vi "main.vi"() -> ()   [LabVIEW 2012]
uses:
  <vilib>/Utility/error.llb/DialogType.ctl
  <instrlib>/Tektronix DPO MSO 2000 4000 Series/Public/Configure/Configure Trigger (Edge).vi
  <instrlib>/Tektronix DPO MSO 2000 4000 Series/Public/Data/Data_Low Level/Fetch Waveform (Waveform Data Type).vi
  <vilib>/regexp/Match Regular Expression.xnode
  <instrlib>/Tektronix DPO MSO 2000 4000 Series/Tektronix DPO MSO 2000 4000 Series.lvlib
panel:
  in  "tabs":T1(tab)=enum."Scope"
  in  "frames":i32=20 caption="Repeated Frames"
  out "current frame":i32=20 caption="Current Frame"
  in  "repetition rate":dbl caption="Max Repetition Rate (mHz)"
  in  "dio64:resource name":refnum<visa-resource-name>="PXI4::0::INSTR"
  out "chop display":picture[](array[picture])=[bytes[78], bytes[76], bytes[76], bytes[80], bytes[84], bytes[72], bytes[72]] caption="Chop Display"
  in  "dio64":T2(array[cluster])=[{"Task"="Gas Pulse", "begin time"=19.288099999999993, "begin edge"=TRUE, "begin reference"="T0", "end time"=0.045, "end edge"=TRUE, "end reference"="<SELF>", "Chops"=[FALSE, FALSE, FALSE, FALSE, FALSE, FALSE, FALSE, FALSE, FALSE, FALSE, FALSE, FALSE]}, {"Task"="Abby Flashlamp", "begin time"=-0.001, "begin edge"=TRUE, "begin reference"="Gas Pulse", "end time"=0.01, "end edge"=TRUE, "end reference"="<SELF>", "Chops"=[FALSE, FALSE, FALSE, FALSE, FALSE, FALSE, FALSE, FALSE, FALSE, FALSE, FALSE, FALSE]}, {"Task"="Abby Q-switch", "begin time"=0.11509999999999998, "begin edge"=FALSE, "begin reference"="Abby Flashlamp", "end time"=0.01, "end edge"=TRUE, "end reference"="<SELF>", "Chops"=[FALSE, FALSE, FALSE, FALSE, FALSE, FALSE, FALSE, FALSE, FALSE, FALSE, FALSE, FALSE]}, {"Task"="Trap", "begin time"=20.1722, "begin edge"=TRUE, "begin reference"="T0", "end time"=500.12, "end edge"=TRUE, "end reference"="<SELF>", "Chops"=[FALSE, FALSE, FALSE, FALSE, FALSE, FALSE, FALSE, FALSE, FALSE, FALSE, FALSE, FALSE]}, {"Task"="Zero DAC", "begin time"=-0.04, "begin edge"=FALSE, "begin reference"="Zero DAC", "end time"=0.0, "end edge"=TRUE, "end reference"="Stop Ions", "Chops"=[FALSE, FALSE, FALSE, FALSE, FALSE, FALSE, FALSE, FALSE, FALSE, FALSE, FALSE, FALSE]}, {"Task"="Stop Ions", "begin time"=-0.001, "begin edge"=FALSE, "begin reference"="Stop Ions", "end time"=0.0, "end edge"=TRUE, "end reference"="Trap", "Chops"=[FALSE, FALSE, FALSE, FALSE, FALSE, FALSE, FALSE, FALSE, FALSE, FALSE, FALSE, FALSE]}, {"Task"="Kick to MCP", "begin time"=0.0, "begin edge"=FALSE, "begin reference"="Trap", "end time"=0.005, "end edge"=TRUE, "end reference"="<SELF>", "Chops"=[FALSE, FALSE, FALSE, FALSE, FALSE, FALSE, FALSE, FALSE, FALSE, FALSE, FALSE, FALSE]}, {"Task"="Img MCP Trigger", "begin time"=0.07001, "begin edge"=FALSE, "begin reference"="Kick to MCP", "end time"=0.01, "end edge"=TRUE, "end reference"="<SELF>", "Chops"=[TRUE, TRUE, TRUE, TRUE, TRUE, TRUE, FALSE, FALSE, FALSE, FALSE, FALSE, FALSE]}, {"Task"="Framegrabber Trigger", "begin time"=-18.0, "begin edge"=TRUE, "begin reference"="Img MCP Trigger", "end time"=0.01, "end edge"=TRUE, "end reference"="<SELF>", "Chops"=[TRUE, TRUE, TRUE, TRUE, TRUE, TRUE, FALSE, FALSE, FALSE, FALSE, FALSE, FALSE]}, {"Task"="Trigger Scope", "begin time"=0.015000000000000006, "begin edge"=FALSE, "begin reference"="Trap", "end time"=0.01, "end edge"=TRUE, "end reference"="<SELF>", "Chops"=[FALSE, FALSE, FALSE, FALSE, FALSE, FALSE, TRUE, FALSE, FALSE, FALSE, FALSE, FALSE]}, {"Task"="Trigger DAC", "begin time"=-1.0, "begin edge"=TRUE, "begin reference"="Trap", "end time"=0.01, "end edge"=TRUE, "end reference"="<SELF>", "Chops"=[FALSE, FALSE, FALSE, FALSE, FALSE, FALSE, FALSE, FALSE, FALSE, FALSE, FALSE, FALSE]}, {"Task"="Zero DAC", "begin time"=0.0, "begin edge"=FALSE, "begin reference"="Kick to MCP", "end time"=10.0, "end edge"=FALSE, "end reference"="Kick to MCP", "Chops"=[FALSE, FALSE, FALSE, FALSE, FALSE, FALSE, FALSE, FALSE, FALSE, FALSE, FALSE, FALSE]}, {"Task"="IOUpdate", "begin time"=-1.9976, "begin edge"=TRUE, "begin reference"="Trap", "end time"=0.01, "end edge"=TRUE, "end reference"="<SELF>", "Chops"=[FALSE, FALSE, FALSE, FALSE, FALSE, FALSE, FALSE, FALSE, FALSE, FALSE, FALSE, FALSE]}, {"Task"="Jessica Shutter", "begin time"=-20.0, "begin edge"=TRUE, "begin reference"="Trap", "end time"=100.0, "end edge"=TRUE, "end reference"="<SELF>", "Chops"=[FALSE, FALSE, FALSE, FALSE, FALSE, FALSE, FALSE, FALSE, FALSE, FALSE, FALSE, FALSE]}, {"Task"="Bertha UV Shutter", "begin time"=-20.0, "begin edge"=TRUE, "begin reference"="Trap", "end time"=100.0, "end edge"=TRUE, "end reference"="<SELF>", "Chops"=[FALSE, FALSE, FALSE, FALSE, FALSE, FALSE, FALSE, FALSE, FALSE, FALSE, FALSE, FALSE]}, {"Task"="Scope trigger 2", "begin time"=0.0, "begin edge"=FALSE, "begin reference"="Trap", "end time"=0.01, "end edge"=TRUE, "end reference"="<SELF>", "Chops"=[TRUE, TRUE, TRUE, FALSE, FALSE, FALSE, FALSE, FALSE, FALSE, FALSE, FALSE, FALSE]}, {"Task"="DDS Ramp 1", "begin time"=11.0, "begin edge"=TRUE, "begin reference"="Trap", "end time"=-1.0, "end edge"=TRUE, "end reference"="Unchillax", "Chops"=[FALSE, FALSE, FALSE, FALSE, TRUE, TRUE, TRUE, FALSE, FALSE, FALSE, FALSE, FALSE]}, {"Task"="Stella Fiber Switch", "begin time"=12.0, "begin edge"=TRUE, "begin reference"="Trap", "end time"=80.0, "end edge"=TRUE, "end reference"="<SELF>", "Chops"=[FALSE, FALSE, FALSE, TRUE, TRUE, TRUE, TRUE, FALSE, FALSE, FALSE, FALSE, FALSE]}, {"Task"="Toptica Fiber Switch", "begin time"=0.0, "begin edge"=TRUE, "begin reference"="Stella Fiber Switch", "end time"=85.0, "end edge"=TRUE, "end reference"="<SELF>", "Chops"=[FALSE, FALSE, FALSE, TRUE, TRUE, TRUE, TRUE, FALSE, FALSE, FALSE, FALSE, FALSE]}, {"Task"="Scope trigger 2 transfer", "begin time"=0.0, "begin edge"=FALSE, "begin reference"="Stella Fiber Switch", "end time"=0.01, "end edge"=TRUE, "end reference"="<SELF>", "Chops"=[TRUE, TRUE, FALSE, TRUE, TRUE, TRUE, TRUE, FALSE, FALSE, FALSE, FALSE, FALSE]}, {"Task"="Change Toptica Wavelength", "begin time"=-10.0, "begin edge"=TRUE, "begin reference"="Trigger Depletion", "end time"=100.0, "end edge"=FALSE, "end reference"="Trigger Depletion 2", "Chops"=[FALSE, FALSE, FALSE, FALSE, TRUE, TRUE, TRUE, FALSE, FALSE, FALSE, FALSE, FALSE]}, {"Task"="Trigger Depletion", "begin time"=110.0, "begin edge"=TRUE, "begin reference"="Trap", "end time"=3.0, "end edge"=TRUE, "end reference"="<SELF>", "Chops"=[FALSE, FALSE, TRUE, TRUE, TRUE, TRUE, TRUE, FALSE, FALSE, FALSE, FALSE, FALSE]}, {"Task"="Trigger Depletion 2", "begin time"=6.0, "begin edge"=FALSE, "begin reference"="Pi/2 Pulse 2", "end time"=3.0, "end edge"=TRUE, "end reference"="<SELF>", "Chops"=[TRUE, FALSE, TRUE, TRUE, TRUE, TRUE, TRUE, FALSE, FALSE, FALSE, FALSE, FALSE]}, {"Task"="Trigger Depletion 2-dephase", "begin time"=0.002, "begin edge"=TRUE, "begin reference"="Trigger Depletion 2", "end time"=3.0, "end edge"=TRUE, "end reference"="<SELF>", "Chops"=[FALSE, TRUE, TRUE, TRUE, TRUE, TRUE, TRUE, FALSE, FALSE, FALSE, FALSE, FALSE]}, {"Task"="Scope trigger 2 depletion", "begin time"=0.0, "begin edge"=TRUE, "begin reference"="Trigger Depletion", "end time"=0.01, "end edge"=TRUE, "end reference"="<SELF>", "Chops"=[FALSE, FALSE, TRUE, TRUE, TRUE, TRUE, TRUE, FALSE, FALSE, FALSE, FALSE, FALSE]}, {"Task"="Cora Shutter", "begin time"=0.0, "begin edge"=TRUE, "begin reference"="266nm Shutter", "end time"=1.0, "end edge"=FALSE, "end reference"="Trap", "Chops"=[FALSE, FALSE, FALSE, FALSE, TRUE, TRUE, TRUE, FALSE, FALSE, FALSE, FALSE, FALSE]}, {"Task"="266nm Shutter", "begin time"=-20.0, "begin edge"=TRUE, "begin reference"="End Ramp", "end time"=0.0, "end edge"=FALSE, "end reference"="Cora Shutter", "Chops"=[FALSE, FALSE, FALSE, FALSE, FALSE, TRUE, TRUE, FALSE, FALSE, FALSE, FALSE, FALSE]}, {"Task"="Chillax", "begin time"=-1.0, "begin edge"=TRUE, "begin reference"="Trap", "end time"=0.01, "end edge"=TRUE, "end reference"="<SELF>", "Chops"=[FALSE, FALSE, FALSE, FALSE, FALSE, FALSE, FALSE, FALSE, FALSE, FALSE, FALSE, FALSE]}, {"Task"="Unchillax", "begin time"=-6.0, "begin edge"=TRUE, "begin reference"="End Ramp", "end time"=0.01, "end edge"=TRUE, "end reference"="<SELF>", "Chops"=[FALSE, FALSE, FALSE, FALSE, FALSE, TRUE, TRUE, FALSE, FALSE, FALSE, FALSE, FALSE]}, {"Task"="End Ramp", "begin time"=-102.0, "begin edge"=FALSE, "begin reference"="Trap", "end time"=0.01, "end edge"=TRUE, "end reference"="<SELF>", "Chops"=[FALSE, FALSE, FALSE, FALSE, FALSE, TRUE, TRUE, FALSE, FALSE, FALSE, FALSE, FALSE]}, {"Task"="End Ramp 2", "begin time"=33.33, "begin edge"=TRUE, "begin reference"="End Ramp", "end time"=33.34, "end edge"=TRUE, "end reference"="End Ramp", "Chops"=[FALSE, FALSE, FALSE, FALSE, FALSE, TRUE, TRUE, FALSE, FALSE, FALSE, FALSE, FALSE]}, {"Task"="End Ramp 2", "begin time"=66.67, "begin edge"=TRUE, "begin reference"="End Ramp", "end time"=66.68, "end edge"=TRUE, "end reference"="End Ramp", "Chops"=[FALSE, FALSE, FALSE, FALSE, FALSE, TRUE, TRUE, FALSE, FALSE, FALSE, FALSE, FALSE]}, {"Task"="End Ramp 2", "begin time"=100.0, "begin edge"=TRUE, "begin reference"="End Ramp", "end time"=100.01, "end edge"=TRUE, "end reference"="End Ramp", "Chops"=[FALSE, FALSE, FALSE, FALSE, FALSE, TRUE, TRUE, FALSE, FALSE, FALSE, FALSE, FALSE]}, {"Task"="Pi/2 Pulse", "begin time"=5.0, "begin edge"=FALSE, "begin reference"="Trigger Depletion", "end time"=0.95, "end edge"=TRUE, "end reference"="<SELF>", "Chops"=[FALSE, FALSE, FALSE, FALSE, TRUE, TRUE, TRUE, FALSE, FALSE, FALSE, FALSE, FALSE]}, {"Task"="Pi/2 Pulse 2", "begin time"=256.0, "begin edge"=FALSE, "begin reference"="Pi/2 Pulse", "end time"=0.95, "end edge"=TRUE, "end reference"="<SELF>", "Chops"=[FALSE, FALSE, FALSE, FALSE, TRUE, TRUE, TRUE, FALSE, FALSE, FALSE, FALSE, FALSE]}] caption="DIO64" {"end time" format="%#_8g"; "begin time" format="%#_8g"}
  in  "dio64:tasks":T3(array[cluster])=[{"Name"="Gas Pulse", "DIO64 Line 1"=[FALSE, FALSE, FALSE, FALSE, FALSE, FALSE, FALSE, FALSE, FALSE, FALSE, FALSE, FALSE, FALSE, FALSE, TRUE, FALSE], "DIO64 Line 2"=[FALSE, FALSE, FALSE, FALSE, FALSE, FALSE, FALSE, FALSE, FALSE, FALSE, FALSE, FALSE, FALSE, FALSE, FALSE, FALSE], "DIO64 Line 3"=[FALSE, FALSE, FALSE, FALSE, FALSE, FALSE, FALSE, FALSE, FALSE, FALSE, FALSE, FALSE, FALSE, FALSE, FALSE, FALSE], "DIO64 Line 4"=[FALSE, FALSE, FALSE, FALSE, FALSE, FALSE, FALSE, FALSE, FALSE, FALSE, FALSE, FALSE, FALSE, FALSE, FALSE, FALSE]}, {"Name"="Abby Flashlamp", "DIO64 Line 1"=[FALSE, FALSE, FALSE, TRUE, FALSE, FALSE, FALSE, FALSE, FALSE, FALSE, FALSE, FALSE, FALSE, FALSE, FALSE, FALSE], "DIO64 Line 2"=[FALSE, FALSE, FALSE, FALSE, FALSE, FALSE, FALSE, FALSE, FALSE, FALSE, FALSE, FALSE, FALSE, FALSE, FALSE, FALSE], "DIO64 Line 3"=[FALSE, FALSE, FALSE, FALSE, FALSE, FALSE, FALSE, FALSE, FALSE, FALSE, FALSE, FALSE, FALSE, FALSE, FALSE, FALSE], "DIO64 Line 4"=[FALSE, FALSE, FALSE, FALSE, FALSE, FALSE, FALSE, FALSE, FALSE, FALSE, FALSE, FALSE, FALSE, FALSE, FALSE, FALSE]}, {"Name"="Abby Q-switch", "DIO64 Line 1"=[FALSE, FALSE, FALSE, FALSE, TRUE, FALSE, FALSE, FALSE, FALSE, FALSE, FALSE, FALSE, FALSE, FALSE, FALSE, FALSE], "DIO64 Line 2"=[FALSE, FALSE, FALSE, FALSE, FALSE, FALSE, FALSE, FALSE, FALSE, FALSE, FALSE, FALSE, FALSE, FALSE, FALSE, FALSE], "DIO64 Line 3"=[FALSE, FALSE, FALSE, FALSE, FALSE, FALSE, FALSE, FALSE, FALSE, FALSE, FALSE, FALSE, FALSE, FALSE, FALSE, FALSE], "DIO64 Line 4"=[FALSE, FALSE, FALSE, FALSE, FALSE, FALSE, FALSE, FALSE, FALSE, FALSE, FALSE, FALSE, FALSE, FALSE, FALSE, FALSE]}, {"Name"="Stop Ions", "DIO64 Line 1"=[FALSE, FALSE, FALSE, FALSE, FALSE, FALSE, FALSE, FALSE, FALSE, TRUE, FALSE, FALSE, FALSE, FALSE, FALSE, FALSE], "DIO64 Line 2"=[FALSE, FALSE, FALSE, FALSE, FALSE, FALSE, FALSE, FALSE, FALSE, FALSE, FALSE, FALSE, FALSE, FALSE, FALSE, FALSE], "DIO64 Line 3"=[FALSE, FALSE, FALSE, FALSE, FALSE, FALSE, FALSE, FALSE, FALSE, FALSE, FALSE, FALSE, FALSE, FALSE, FALSE, FALSE], "DIO64 Line 4"=[FALSE, FALSE, FALSE, FALSE, FALSE, FALSE, FALSE, FALSE, FALSE, FALSE, FALSE, FALSE, FALSE, FALSE, FALSE, FALSE]}, {"Name"="Trap", "DIO64 Line 1"=[FALSE, FALSE, FALSE, FALSE, FALSE, FALSE, TRUE, FALSE, FALSE, FALSE, FALSE, FALSE, FALSE, FALSE, FALSE, FALSE], "DIO64 Line 2"=[FALSE, FALSE, FALSE, FALSE, TRUE, FALSE, FALSE, FALSE, FALSE, FALSE, FALSE, FALSE, FALSE, TRUE, FALSE, FALSE], "DIO64 Line 3"=[FALSE, FALSE, FALSE, TRUE, FALSE, FALSE, FALSE, FALSE, FALSE, FALSE, FALSE, FALSE, FALSE, FALSE, FALSE, FALSE], "DIO64 Line 4"=[FALSE, FALSE, FALSE, FALSE, FALSE, FALSE, FALSE, FALSE, FALSE, FALSE, FALSE, FALSE, FALSE, FALSE, FALSE, TRUE]}, {"Name"="Zero DAC", "DIO64 Line 1"=[FALSE, FALSE, FALSE, FALSE, FALSE, FALSE, FALSE, FALSE, FALSE, TRUE, TRUE, FALSE, FALSE, FALSE, FALSE, FALSE], "DIO64 Line 2"=[FALSE, FALSE, FALSE, FALSE, FALSE, FALSE, FALSE, FALSE, FALSE, FALSE, FALSE, FALSE, FALSE, FALSE, FALSE, FALSE], "DIO64 Line 3"=[FALSE, FALSE, FALSE, FALSE, FALSE, FALSE, FALSE, FALSE, FALSE, FALSE, FALSE, FALSE, FALSE, FALSE, FALSE, FALSE], "DIO64 Line 4"=[FALSE, FALSE, FALSE, FALSE, FALSE, FALSE, FALSE, FALSE, FALSE, FALSE, FALSE, FALSE, FALSE, FALSE, FALSE, FALSE]}, {"Name"="Kick to MCP", "DIO64 Line 1"=[FALSE, FALSE, FALSE, FALSE, FALSE, FALSE, FALSE, FALSE, FALSE, TRUE, FALSE, FALSE, FALSE, FALSE, FALSE, FALSE], "DIO64 Line 2"=[FALSE, FALSE, FALSE, FALSE, FALSE, FALSE, FALSE, FALSE, FALSE, FALSE, FALSE, FALSE, FALSE, FALSE, FALSE, FALSE], "DIO64 Line 3"=[FALSE, FALSE, FALSE, FALSE, FALSE, FALSE, FALSE, FALSE, FALSE, FALSE, FALSE, FALSE, FALSE, FALSE, FALSE, FALSE], "DIO64 Line 4"=[FALSE, FALSE, FALSE, FALSE, FALSE, FALSE, FALSE, FALSE, FALSE, FALSE, FALSE, FALSE, FALSE, FALSE, FALSE, FALSE]}, {"Name"="Trap Frequency", "DIO64 Line 1"=[FALSE, FALSE, FALSE, FALSE, FALSE, FALSE, FALSE, FALSE, FALSE, FALSE, FALSE, FALSE, FALSE, FALSE, FALSE, FALSE], "DIO64 Line 2"=[FALSE, FALSE, FALSE, FALSE, FALSE, FALSE, FALSE, FALSE, FALSE, FALSE, FALSE, FALSE, FALSE, FALSE, FALSE, FALSE], "DIO64 Line 3"=[FALSE, FALSE, FALSE, FALSE, FALSE, FALSE, FALSE, FALSE, FALSE, FALSE, FALSE, FALSE, FALSE, FALSE, FALSE, FALSE], "DIO64 Line 4"=[FALSE, FALSE, FALSE, FALSE, FALSE, FALSE, FALSE, FALSE, FALSE, FALSE, FALSE, FALSE, FALSE, FALSE, FALSE, FALSE]}, {"Name"="Trigger Scope", "DIO64 Line 1"=[FALSE, FALSE, FALSE, FALSE, FALSE, FALSE, FALSE, TRUE, FALSE, FALSE, FALSE, FALSE, FALSE, FALSE, FALSE, FALSE], "DIO64 Line 2"=[FALSE, FALSE, FALSE, FALSE, FALSE, FALSE, FALSE, FALSE, FALSE, FALSE, FALSE, FALSE, FALSE, FALSE, FALSE, FALSE], "DIO64 Line 3"=[FALSE, FALSE, FALSE, FALSE, FALSE, FALSE, FALSE, FALSE, FALSE, FALSE, FALSE, FALSE, FALSE, FALSE, FALSE, FALSE], "DIO64 Line 4"=[FALSE, TRUE, FALSE, FALSE, FALSE, FALSE, FALSE, FALSE, FALSE, FALSE, FALSE, FALSE, FALSE, FALSE, FALSE, FALSE]}, {"Name"="End Cap SW0", "DIO64 Line 1"=[FALSE, FALSE, FALSE, FALSE, FALSE, FALSE, FALSE, FALSE, FALSE, FALSE, FALSE, FALSE, FALSE, FALSE, FALSE, FALSE], "DIO64 Line 2"=[FALSE, FALSE, FALSE, FALSE, TRUE, FALSE, FALSE, FALSE, FALSE, FALSE, FALSE, FALSE, FALSE, FALSE, FALSE, FALSE], "DIO64 Line 3"=[FALSE, FALSE, FALSE, FALSE, FALSE, FALSE, FALSE, FALSE, FALSE, FALSE, FALSE, FALSE, FALSE, FALSE, FALSE, FALSE], "DIO64 Line 4"=[FALSE, FALSE, FALSE, FALSE, FALSE, FALSE, FALSE, FALSE, FALSE, FALSE, FALSE, FALSE, FALSE, FALSE, FALSE, FALSE]}, {"Name"="Framegrabber Trigger", "DIO64 Line 1"=[FALSE, FALSE, FALSE, FALSE, FALSE, FALSE, FALSE, FALSE, FALSE, FALSE, FALSE, FALSE, FALSE, FALSE, FALSE, TRUE], "DIO64 Line 2"=[FALSE, FALSE, FALSE, FALSE, FALSE, FALSE, FALSE, FALSE, FALSE, FALSE, FALSE, FALSE, FALSE, FALSE, FALSE, FALSE], "DIO64 Line 3"=[FALSE, FALSE, FALSE, FALSE, FALSE, FALSE, FALSE, FALSE, FALSE, FALSE, FALSE, FALSE, FALSE, FALSE, FALSE, FALSE], "DIO64 Line 4"=[FALSE, FALSE, TRUE, FALSE, FALSE, FALSE, FALSE, FALSE, FALSE, FALSE, FALSE, FALSE, FALSE, FALSE, FALSE, FALSE]}, {"Name"="Lisa Shutter", "DIO64 Line 1"=[FALSE, FALSE, FALSE, FALSE, FALSE, FALSE, FALSE, FALSE, FALSE, FALSE, FALSE, FALSE, FALSE, FALSE, FALSE, FALSE], "DIO64 Line 2"=[TRUE, FALSE, FALSE, FALSE, FALSE, FALSE, FALSE, FALSE, FALSE, FALSE, FALSE, FALSE, FALSE, FALSE, FALSE, FALSE], "DIO64 Line 3"=[FALSE, FALSE, FALSE, FALSE, FALSE, FALSE, FALSE, FALSE, FALSE, FALSE, FALSE, FALSE, FALSE, FALSE, FALSE, FALSE], "DIO64 Line 4"=[FALSE, FALSE, FALSE, FALSE, FALSE, FALSE, FALSE, FALSE, FALSE, FALSE, FALSE, FALSE, FALSE, FALSE, FALSE, FALSE]}, {"Name"="Trigger DAC", "DIO64 Line 1"=[FALSE, FALSE, FALSE, FALSE, FALSE, FALSE, FALSE, FALSE, FALSE, FALSE, FALSE, FALSE, FALSE, FALSE, FALSE, FALSE], "DIO64 Line 2"=[FALSE, FALSE, FALSE, FALSE, FALSE, FALSE, FALSE, FALSE, FALSE, TRUE, FALSE, FALSE, FALSE, FALSE, FALSE, FALSE], "DIO64 Line 3"=[FALSE, FALSE, FALSE, FALSE, FALSE, FALSE, FALSE, FALSE, FALSE, FALSE, FALSE, FALSE, FALSE, FALSE, FALSE, FALSE], "DIO64 Line 4"=[FALSE, FALSE, FALSE, FALSE, FALSE, FALSE, FALSE, FALSE, FALSE, FALSE, FALSE, FALSE, FALSE, FALSE, FALSE, FALSE]}, {"Name"="Jessica Shutter", "DIO64 Line 1"=[FALSE, FALSE, FALSE, FALSE, FALSE, FALSE, FALSE, FALSE, FALSE, FALSE, FALSE, FALSE, FALSE, TRUE, FALSE, FALSE], "DIO64 Line 2"=[FALSE, FALSE, FALSE, FALSE, FALSE, FALSE, FALSE, FALSE, FALSE, FALSE, FALSE, FALSE, FALSE, FALSE, FALSE, FALSE], "DIO64 Line 3"=[FALSE, FALSE, FALSE, FALSE, FALSE, FALSE, FALSE, FALSE, FALSE, FALSE, FALSE, FALSE, FALSE, FALSE, FALSE, FALSE], "DIO64 Line 4"=[FALSE, FALSE, FALSE, FALSE, FALSE, FALSE, FALSE, FALSE, FALSE, FALSE, FALSE, FALSE, FALSE, FALSE, FALSE, FALSE]}, {"Name"="Img MCP Trigger", "DIO64 Line 1"=[FALSE, FALSE, FALSE, FALSE, FALSE, TRUE, FALSE, FALSE, FALSE, FALSE, FALSE, FALSE, FALSE, FALSE, FALSE, FALSE], "DIO64 Line 2"=[FALSE, FALSE, FALSE, FALSE, FALSE, FALSE, FALSE, FALSE, FALSE, FALSE, FALSE, FALSE, FALSE, FALSE, FALSE, FALSE], "DIO64 Line 3"=[FALSE, FALSE, FALSE, FALSE, FALSE, FALSE, FALSE, FALSE, FALSE, FALSE, FALSE, FALSE, FALSE, FALSE, FALSE, FALSE], "DIO64 Line 4"=[FALSE, FALSE, FALSE, FALSE, FALSE, FALSE, FALSE, FALSE, FALSE, FALSE, FALSE, FALSE, FALSE, FALSE, FALSE, FALSE]}, {"Name"="Nothing", "DIO64 Line 1"=[FALSE, FALSE, FALSE, FALSE, FALSE, FALSE, FALSE, FALSE, FALSE, FALSE, FALSE, FALSE, FALSE, FALSE, FALSE, FALSE], "DIO64 Line 2"=[FALSE, FALSE, FALSE, FALSE, FALSE, FALSE, FALSE, FALSE, FALSE, FALSE, FALSE, FALSE, FALSE, FALSE, FALSE, FALSE], "DIO64 Line 3"=[FALSE, FALSE, FALSE, FALSE, FALSE, FALSE, FALSE, FALSE, FALSE, FALSE, FALSE, FALSE, FALSE, FALSE, FALSE, FALSE], "DIO64 Line 4"=[FALSE, FALSE, FALSE, FALSE, FALSE, FALSE, FALSE, FALSE, FALSE, FALSE, FALSE, FALSE, FALSE, FALSE, FALSE, FALSE]}, {"Name"="End Ramp", "DIO64 Line 1"=[FALSE, FALSE, FALSE, FALSE, FALSE, FALSE, FALSE, FALSE, FALSE, FALSE, FALSE, FALSE, TRUE, FALSE, FALSE, FALSE], "DIO64 Line 2"=[FALSE, FALSE, FALSE, FALSE, FALSE, FALSE, FALSE, FALSE, FALSE, FALSE, FALSE, FALSE, FALSE, FALSE, FALSE, FALSE], "DIO64 Line 3"=[FALSE, FALSE, FALSE, FALSE, FALSE, FALSE, FALSE, FALSE, FALSE, FALSE, FALSE, FALSE, FALSE, FALSE, FALSE, FALSE], "DIO64 Line 4"=[FALSE, FALSE, FALSE, FALSE, FALSE, FALSE, FALSE, FALSE, FALSE, FALSE, FALSE, FALSE, FALSE, FALSE, FALSE, FALSE]}, {"Name"="End Ramp 2", "DIO64 Line 1"=[FALSE, FALSE, FALSE, FALSE, FALSE, FALSE, FALSE, FALSE, FALSE, FALSE, FALSE, FALSE, TRUE, FALSE, FALSE, FALSE], "DIO64 Line 2"=[FALSE, FALSE, FALSE, FALSE, FALSE, FALSE, FALSE, FALSE, FALSE, FALSE, FALSE, FALSE, FALSE, FALSE, FALSE, FALSE], "DIO64 Line 3"=[FALSE, FALSE, FALSE, FALSE, FALSE, FALSE, FALSE, FALSE, FALSE, FALSE, FALSE, FALSE, FALSE, FALSE, FALSE, FALSE], "DIO64 Line 4"=[FALSE, FALSE, FALSE, FALSE, FALSE, FALSE, FALSE, FALSE, FALSE, FALSE, FALSE, FALSE, FALSE, FALSE, FALSE, FALSE]}, {"Name"="Step Bertha Scan", "DIO64 Line 1"=[FALSE, FALSE, FALSE, FALSE, FALSE, FALSE, FALSE, FALSE, FALSE, FALSE, FALSE, FALSE, FALSE, FALSE, FALSE, FALSE], "DIO64 Line 2"=[FALSE, FALSE, FALSE, FALSE, FALSE, FALSE, FALSE, FALSE, FALSE, FALSE, FALSE, TRUE, FALSE, FALSE, FALSE, FALSE], "DIO64 Line 3"=[FALSE, FALSE, FALSE, FALSE, FALSE, FALSE, FALSE, FALSE, FALSE, FALSE, FALSE, FALSE, FALSE, FALSE, FALSE, FALSE], "DIO64 Line 4"=[FALSE, FALSE, FALSE, FALSE, FALSE, FALSE, FALSE, FALSE, FALSE, FALSE, FALSE, FALSE, FALSE, FALSE, FALSE, FALSE]}, {"Name"="Bertha UV Shutter", "DIO64 Line 1"=[FALSE, FALSE, FALSE, FALSE, FALSE, FALSE, FALSE, FALSE, FALSE, FALSE, FALSE, FALSE, FALSE, FALSE, FALSE, FALSE], "DIO64 Line 2"=[FALSE, FALSE, FALSE, FALSE, FALSE, FALSE, FALSE, FALSE, FALSE, FALSE, FALSE, FALSE, FALSE, FALSE, FALSE, TRUE], "DIO64 Line 3"=[FALSE, FALSE, FALSE, FALSE, FALSE, FALSE, FALSE, FALSE, FALSE, FALSE, FALSE, FALSE, FALSE, FALSE, FALSE, FALSE], "DIO64 Line 4"=[FALSE, FALSE, FALSE, FALSE, FALSE, FALSE, FALSE, FALSE, FALSE, FALSE, FALSE, FALSE, FALSE, FALSE, FALSE, FALSE]}, {"Name"="Kick to Fast MCP TOFMS", "DIO64 Line 1"=[FALSE, FALSE, FALSE, FALSE, FALSE, TRUE, FALSE, FALSE, FALSE, FALSE, FALSE, FALSE, FALSE, FALSE, FALSE, FALSE], "DIO64 Line 2"=[FALSE, FALSE, FALSE, FALSE, FALSE, FALSE, FALSE, FALSE, FALSE, FALSE, FALSE, FALSE, FALSE, FALSE, FALSE, FALSE], "DIO64 Line 3"=[FALSE, FALSE, FALSE, FALSE, FALSE, FALSE, FALSE, FALSE, FALSE, FALSE, FALSE, FALSE, FALSE, FALSE, FALSE, FALSE], "DIO64 Line 4"=[FALSE, FALSE, FALSE, FALSE, FALSE, FALSE, FALSE, FALSE, FALSE, FALSE, FALSE, FALSE, FALSE, FALSE, FALSE, FALSE]}, {"Name"="End Cap SW1", "DIO64 Line 1"=[FALSE, FALSE, FALSE, FALSE, FALSE, FALSE, FALSE, FALSE, FALSE, FALSE, FALSE, FALSE, FALSE, FALSE, FALSE, FALSE], "DIO64 Line 2"=[FALSE, FALSE, FALSE, FALSE, FALSE, FALSE, FALSE, FALSE, FALSE, FALSE, FALSE, FALSE, FALSE, TRUE, FALSE, FALSE], "DIO64 Line 3"=[FALSE, FALSE, FALSE, FALSE, FALSE, FALSE, FALSE, FALSE, FALSE, FALSE, FALSE, FALSE, FALSE, FALSE, FALSE, FALSE], "DIO64 Line 4"=[FALSE, FALSE, FALSE, FALSE, FALSE, FALSE, FALSE, FALSE, FALSE, FALSE, FALSE, FALSE, FALSE, FALSE, FALSE, FALSE]}, {"Name"="Scope trigger 2", "DIO64 Line 1"=[FALSE, FALSE, FALSE, FALSE, FALSE, FALSE, FALSE, FALSE, FALSE, FALSE, FALSE, FALSE, FALSE, FALSE, FALSE, FALSE], "DIO64 Line 2"=[FALSE, FALSE, FALSE, FALSE, FALSE, FALSE, FALSE, FALSE, FALSE, FALSE, FALSE, TRUE, FALSE, FALSE, FALSE, FALSE], "DIO64 Line 3"=[FALSE, FALSE, FALSE, FALSE, FALSE, FALSE, FALSE, FALSE, FALSE, FALSE, FALSE, FALSE, FALSE, FALSE, FALSE, FALSE], "DIO64 Line 4"=[FALSE, FALSE, FALSE, FALSE, FALSE, FALSE, FALSE, FALSE, FALSE, FALSE, FALSE, FALSE, FALSE, FALSE, FALSE, FALSE]}, {"Name"="266nm Shutter", "DIO64 Line 1"=[FALSE, FALSE, FALSE, FALSE, FALSE, FALSE, FALSE, FALSE, FALSE, FALSE, FALSE, FALSE, FALSE, FALSE, FALSE, FALSE], "DIO64 Line 2"=[FALSE, FALSE, FALSE, FALSE, FALSE, TRUE, FALSE, FALSE, FALSE, FALSE, FALSE, FALSE, FALSE, FALSE, FALSE, FALSE], "DIO64 Line 3"=[FALSE, FALSE, FALSE, FALSE, FALSE, FALSE, FALSE, FALSE, FALSE, FALSE, FALSE, FALSE, FALSE, FALSE, FALSE, FALSE], "DIO64 Line 4"=[FALSE, FALSE, FALSE, FALSE, FALSE, FALSE, FALSE, FALSE, FALSE, FALSE, FALSE, FALSE, FALSE, FALSE, FALSE, FALSE]}, {"Name"="532/1064nm Shutter", "DIO64 Line 1"=[FALSE, FALSE, FALSE, FALSE, FALSE, FALSE, FALSE, FALSE, FALSE, FALSE, FALSE, FALSE, FALSE, FALSE, FALSE, FALSE], "DIO64 Line 2"=[FALSE, FALSE, FALSE, FALSE, FALSE, FALSE, TRUE, FALSE, FALSE, FALSE, FALSE, FALSE, FALSE, FALSE, FALSE, FALSE], "DIO64 Line 3"=[FALSE, FALSE, FALSE, FALSE, FALSE, FALSE, FALSE, FALSE, FALSE, FALSE, FALSE, FALSE, FALSE, FALSE, FALSE, FALSE], "DIO64 Line 4"=[FALSE, FALSE, FALSE, FALSE, FALSE, FALSE, FALSE, FALSE, FALSE, FALSE, FALSE, FALSE, FALSE, FALSE, FALSE, FALSE]}, {"Name"="Bertha Fund Shutter", "DIO64 Line 1"=[FALSE, FALSE, FALSE, FALSE, FALSE, FALSE, FALSE, FALSE, FALSE, FALSE, FALSE, FALSE, FALSE, FALSE, FALSE, FALSE], "DIO64 Line 2"=[FALSE, FALSE, FALSE, FALSE, FALSE, FALSE, FALSE, FALSE, FALSE, FALSE, FALSE, FALSE, FALSE, FALSE, FALSE, FALSE], "DIO64 Line 3"=[FALSE, FALSE, FALSE, FALSE, FALSE, FALSE, FALSE, FALSE, FALSE, FALSE, FALSE, FALSE, FALSE, FALSE, FALSE, FALSE], "DIO64 Line 4"=[FALSE, FALSE, FALSE, FALSE, FALSE, FALSE, FALSE, FALSE, FALSE, FALSE, FALSE, FALSE, FALSE, FALSE, FALSE, FALSE]}, {"Name"="toptica aom switch", "DIO64 Line 1"=[FALSE, TRUE, FALSE, FALSE, FALSE, FALSE, FALSE, FALSE, FALSE, FALSE, FALSE, FALSE, FALSE, FALSE, FALSE, FALSE], "DIO64 Line 2"=[FALSE, FALSE, FALSE, FALSE, FALSE, FALSE, FALSE, FALSE, FALSE, FALSE, FALSE, FALSE, FALSE, FALSE, FALSE, FALSE], "DIO64 Line 3"=[FALSE, FALSE, FALSE, FALSE, FALSE, FALSE, FALSE, FALSE, FALSE, FALSE, FALSE, TRUE, FALSE, FALSE, FALSE, FALSE], "DIO64 Line 4"=[FALSE, FALSE, FALSE, FALSE, FALSE, FALSE, FALSE, FALSE, FALSE, FALSE, FALSE, FALSE, FALSE, FALSE, FALSE, FALSE]}, {"Name"="Stop Voltage", "DIO64 Line 1"=[FALSE, FALSE, FALSE, FALSE, FALSE, FALSE, FALSE, FALSE, FALSE, FALSE, FALSE, FALSE, FALSE, FALSE, FALSE, FALSE], "DIO64 Line 2"=[FALSE, FALSE, FALSE, FALSE, TRUE, FALSE, FALSE, FALSE, FALSE, FALSE, FALSE, FALSE, FALSE, FALSE, FALSE, FALSE], "DIO64 Line 3"=[FALSE, FALSE, FALSE, FALSE, FALSE, FALSE, FALSE, FALSE, FALSE, FALSE, FALSE, FALSE, FALSE, FALSE, FALSE, FALSE], "DIO64 Line 4"=[FALSE, FALSE, FALSE, FALSE, FALSE, FALSE, FALSE, FALSE, FALSE, FALSE, FALSE, FALSE, FALSE, FALSE, FALSE, FALSE]}, {"Name"="Kick Voltage", "DIO64 Line 1"=[FALSE, FALSE, FALSE, FALSE, FALSE, FALSE, FALSE, FALSE, FALSE, FALSE, FALSE, FALSE, FALSE, FALSE, FALSE, FALSE], "DIO64 Line 2"=[FALSE, FALSE, FALSE, FALSE, FALSE, FALSE, FALSE, FALSE, FALSE, FALSE, FALSE, FALSE, FALSE, FALSE, FALSE, FALSE], "DIO64 Line 3"=[FALSE, FALSE, FALSE, FALSE, FALSE, FALSE, FALSE, FALSE, FALSE, FALSE, FALSE, FALSE, FALSE, FALSE, FALSE, FALSE], "DIO64 Line 4"=[FALSE, FALSE, FALSE, FALSE, FALSE, FALSE, FALSE, FALSE, FALSE, FALSE, FALSE, FALSE, FALSE, FALSE, FALSE, FALSE]}, {"Name"="Stella Fiber Switch", "DIO64 Line 1"=[FALSE, FALSE, FALSE, FALSE, FALSE, FALSE, FALSE, FALSE, FALSE, FALSE, FALSE, FALSE, FALSE, FALSE, FALSE, FALSE], "DIO64 Line 2"=[FALSE, FALSE, FALSE, FALSE, FALSE, FALSE, FALSE, FALSE, FALSE, FALSE, FALSE, FALSE, FALSE, FALSE, TRUE, FALSE], "DIO64 Line 3"=[FALSE, FALSE, FALSE, FALSE, FALSE, FALSE, FALSE, FALSE, FALSE, FALSE, FALSE, FALSE, FALSE, FALSE, FALSE, FALSE], "DIO64 Line 4"=[FALSE, FALSE, FALSE, FALSE, FALSE, FALSE, FALSE, FALSE, FALSE, FALSE, FALSE, FALSE, FALSE, FALSE, FALSE, FALSE]}, {"Name"="Trigger Depletion 2-dephase", "DIO64 Line 1"=[FALSE, FALSE, FALSE, FALSE, FALSE, FALSE, FALSE, FALSE, FALSE, FALSE, FALSE, FALSE, FALSE, FALSE, FALSE, FALSE], "DIO64 Line 2"=[FALSE, FALSE, FALSE, FALSE, FALSE, FALSE, FALSE, FALSE, TRUE, FALSE, FALSE, FALSE, FALSE, FALSE, FALSE, FALSE], "DIO64 Line 3"=[FALSE, FALSE, FALSE, FALSE, FALSE, FALSE, FALSE, FALSE, FALSE, FALSE, FALSE, FALSE, FALSE, FALSE, FALSE, FALSE], "DIO64 Line 4"=[FALSE, FALSE, FALSE, FALSE, FALSE, FALSE, FALSE, FALSE, FALSE, FALSE, FALSE, FALSE, FALSE, FALSE, FALSE, FALSE]}, {"Name"="Cora Shutter", "DIO64 Line 1"=[FALSE, FALSE, FALSE, FALSE, FALSE, FALSE, FALSE, FALSE, FALSE, FALSE, FALSE, FALSE, FALSE, FALSE, FALSE, FALSE], "DIO64 Line 2"=[FALSE, TRUE, FALSE, FALSE, FALSE, FALSE, FALSE, FALSE, FALSE, FALSE, FALSE, FALSE, FALSE, FALSE, FALSE, FALSE], "DIO64 Line 3"=[FALSE, FALSE, FALSE, FALSE, FALSE, FALSE, FALSE, FALSE, FALSE, FALSE, FALSE, FALSE, FALSE, FALSE, FALSE, FALSE], "DIO64 Line 4"=[FALSE, FALSE, FALSE, FALSE, FALSE, FALSE, FALSE, FALSE, FALSE, FALSE, FALSE, FALSE, FALSE, FALSE, FALSE, FALSE]}, {"Name"="Step Cora Scan", "DIO64 Line 1"=[FALSE, FALSE, FALSE, FALSE, FALSE, FALSE, FALSE, FALSE, TRUE, FALSE, FALSE, FALSE, FALSE, FALSE, FALSE, FALSE], "DIO64 Line 2"=[FALSE, FALSE, FALSE, FALSE, FALSE, FALSE, FALSE, FALSE, FALSE, FALSE, FALSE, FALSE, FALSE, FALSE, FALSE, FALSE], "DIO64 Line 3"=[FALSE, FALSE, FALSE, FALSE, FALSE, FALSE, FALSE, FALSE, FALSE, FALSE, FALSE, FALSE, FALSE, FALSE, FALSE, FALSE], "DIO64 Line 4"=[FALSE, FALSE, FALSE, FALSE, FALSE, FALSE, FALSE, FALSE, FALSE, FALSE, FALSE, FALSE, FALSE, FALSE, FALSE, FALSE]}, {"Name"="DDS Ramp 1", "DIO64 Line 1"=[FALSE, FALSE, FALSE, FALSE, FALSE, FALSE, FALSE, FALSE, FALSE, FALSE, FALSE, FALSE, FALSE, FALSE, FALSE, FALSE], "DIO64 Line 2"=[TRUE, FALSE, FALSE, FALSE, FALSE, FALSE, FALSE, FALSE, FALSE, FALSE, FALSE, FALSE, FALSE, FALSE, FALSE, FALSE], "DIO64 Line 3"=[FALSE, FALSE, FALSE, FALSE, FALSE, FALSE, FALSE, FALSE, FALSE, FALSE, FALSE, FALSE, FALSE, FALSE, FALSE, FALSE], "DIO64 Line 4"=[FALSE, FALSE, FALSE, FALSE, FALSE, FALSE, FALSE, FALSE, FALSE, FALSE, FALSE, FALSE, FALSE, FALSE, FALSE, FALSE]}, {"Name"="Toptica Fiber Switch", "DIO64 Line 1"=[FALSE, FALSE, FALSE, FALSE, FALSE, FALSE, FALSE, FALSE, FALSE, FALSE, FALSE, TRUE, FALSE, FALSE, FALSE, FALSE], "DIO64 Line 2"=[FALSE, FALSE, FALSE, FALSE, FALSE, FALSE, FALSE, FALSE, FALSE, FALSE, FALSE, FALSE, FALSE, FALSE, FALSE, FALSE], "DIO64 Line 3"=[FALSE, FALSE, FALSE, FALSE, FALSE, FALSE, FALSE, FALSE, FALSE, FALSE, FALSE, FALSE, FALSE, FALSE, FALSE, FALSE], "DIO64 Line 4"=[FALSE, FALSE, FALSE, FALSE, FALSE, FALSE, FALSE, FALSE, FALSE, FALSE, FALSE, FALSE, FALSE, FALSE, FALSE, FALSE]}, {"Name"="Trigger Rotating", "DIO64 Line 1"=[FALSE, FALSE, FALSE, FALSE, FALSE, FALSE, FALSE, FALSE, FALSE, FALSE, FALSE, FALSE, FALSE, FALSE, FALSE, FALSE], "DIO64 Line 2"=[FALSE, FALSE, TRUE, FALSE, FALSE, FALSE, FALSE, FALSE, FALSE, FALSE, FALSE, FALSE, FALSE, FALSE, FALSE, FALSE], "DIO64 Line 3"=[FALSE, FALSE, FALSE, FALSE, FALSE, FALSE, FALSE, FALSE, FALSE, FALSE, FALSE, FALSE, FALSE, FALSE, FALSE, FALSE], "DIO64 Line 4"=[FALSE, FALSE, FALSE, FALSE, FALSE, FALSE, FALSE, FALSE, FALSE, FALSE, FALSE, FALSE, FALSE, FALSE, FALSE, FALSE]}, {"Name"="IOUpdate", "DIO64 Line 1"=[FALSE, FALSE, FALSE, FALSE, FALSE, FALSE, FALSE, FALSE, FALSE, FALSE, FALSE, FALSE, FALSE, FALSE, FALSE, FALSE], "DIO64 Line 2"=[FALSE, FALSE, FALSE, FALSE, FALSE, FALSE, FALSE, FALSE, FALSE, FALSE, FALSE, FALSE, FALSE, FALSE, FALSE, FALSE], "DIO64 Line 3"=[FALSE, FALSE, FALSE, FALSE, FALSE, FALSE, FALSE, FALSE, FALSE, FALSE, FALSE, FALSE, FALSE, FALSE, FALSE, FALSE], "DIO64 Line 4"=[TRUE, FALSE, FALSE, FALSE, FALSE, FALSE, FALSE, FALSE, FALSE, FALSE, FALSE, FALSE, FALSE, FALSE, FALSE, FALSE]}, {"Name"="Trigger Depletion", "DIO64 Line 1"=[FALSE, FALSE, FALSE, FALSE, FALSE, FALSE, FALSE, FALSE, FALSE, FALSE, FALSE, FALSE, FALSE, FALSE, FALSE, FALSE], "DIO64 Line 2"=[FALSE, FALSE, FALSE, FALSE, FALSE, FALSE, FALSE, FALSE, TRUE, FALSE, FALSE, FALSE, FALSE, FALSE, FALSE, FALSE], "DIO64 Line 3"=[FALSE, FALSE, FALSE, FALSE, FALSE, FALSE, FALSE, FALSE, FALSE, FALSE, FALSE, FALSE, FALSE, FALSE, FALSE, FALSE], "DIO64 Line 4"=[FALSE, FALSE, FALSE, FALSE, FALSE, FALSE, FALSE, FALSE, FALSE, FALSE, FALSE, FALSE, FALSE, FALSE, FALSE, FALSE]}, {"Name"="Trigger Depletion 2", "DIO64 Line 1"=[FALSE, FALSE, FALSE, FALSE, FALSE, FALSE, FALSE, FALSE, FALSE, FALSE, FALSE, FALSE, FALSE, FALSE, FALSE, FALSE], "DIO64 Line 2"=[FALSE, FALSE, FALSE, FALSE, FALSE, FALSE, FALSE, FALSE, TRUE, FALSE, FALSE, FALSE, FALSE, FALSE, FALSE, FALSE], "DIO64 Line 3"=[FALSE, FALSE, FALSE, FALSE, FALSE, FALSE, FALSE, FALSE, FALSE, FALSE, FALSE, FALSE, FALSE, FALSE, FALSE, FALSE], "DIO64 Line 4"=[FALSE, FALSE, FALSE, FALSE, FALSE, FALSE, FALSE, FALSE, FALSE, FALSE, FALSE, FALSE, FALSE, FALSE, FALSE, FALSE]}, {"Name"="Vertical Depletion", "DIO64 Line 1"=[FALSE, FALSE, FALSE, FALSE, FALSE, FALSE, FALSE, FALSE, FALSE, FALSE, FALSE, TRUE, FALSE, FALSE, FALSE, FALSE], "DIO64 Line 2"=[FALSE, FALSE, FALSE, FALSE, FALSE, FALSE, FALSE, FALSE, FALSE, FALSE, FALSE, FALSE, FALSE, FALSE, FALSE, FALSE], "DIO64 Line 3"=[FALSE, FALSE, FALSE, FALSE, FALSE, FALSE, FALSE, FALSE, FALSE, FALSE, FALSE, FALSE, FALSE, FALSE, FALSE, FALSE], "DIO64 Line 4"=[FALSE, FALSE, FALSE, FALSE, FALSE, FALSE, FALSE, FALSE, FALSE, FALSE, FALSE, FALSE, FALSE, FALSE, FALSE, FALSE]}, {"Name"="Scope trigger 2 transfer", "DIO64 Line 1"=[FALSE, FALSE, FALSE, FALSE, FALSE, FALSE, FALSE, FALSE, FALSE, FALSE, FALSE, FALSE, FALSE, FALSE, FALSE, FALSE], "DIO64 Line 2"=[FALSE, FALSE, FALSE, FALSE, FALSE, FALSE, FALSE, FALSE, FALSE, FALSE, FALSE, TRUE, FALSE, FALSE, FALSE, FALSE], "DIO64 Line 3"=[FALSE, FALSE, FALSE, FALSE, FALSE, FALSE, FALSE, FALSE, FALSE, FALSE, FALSE, FALSE, FALSE, FALSE, FALSE, FALSE], "DIO64 Line 4"=[FALSE, FALSE, FALSE, FALSE, FALSE, FALSE, FALSE, FALSE, FALSE, FALSE, FALSE, FALSE, FALSE, FALSE, FALSE, FALSE]}, {"Name"="Unchillax", "DIO64 Line 1"=[FALSE, FALSE, FALSE, FALSE, FALSE, FALSE, FALSE, FALSE, FALSE, FALSE, FALSE, FALSE, FALSE, FALSE, FALSE, FALSE], "DIO64 Line 2"=[FALSE, FALSE, FALSE, FALSE, FALSE, FALSE, FALSE, FALSE, FALSE, FALSE, FALSE, FALSE, FALSE, FALSE, FALSE, FALSE], "DIO64 Line 3"=[TRUE, FALSE, FALSE, FALSE, FALSE, FALSE, FALSE, FALSE, FALSE, FALSE, FALSE, FALSE, FALSE, FALSE, FALSE, FALSE], "DIO64 Line 4"=[FALSE, FALSE, FALSE, FALSE, FALSE, FALSE, FALSE, FALSE, FALSE, FALSE, FALSE, FALSE, FALSE, FALSE, FALSE, FALSE]}, {"Name"="Pi/2 Pulse", "DIO64 Line 1"=[FALSE, FALSE, FALSE, FALSE, FALSE, FALSE, FALSE, FALSE, FALSE, FALSE, FALSE, FALSE, FALSE, FALSE, FALSE, FALSE], "DIO64 Line 2"=[FALSE, FALSE, FALSE, FALSE, FALSE, FALSE, FALSE, FALSE, FALSE, FALSE, FALSE, FALSE, TRUE, FALSE, FALSE, FALSE], "DIO64 Line 3"=[FALSE, FALSE, FALSE, FALSE, FALSE, FALSE, FALSE, FALSE, FALSE, FALSE, FALSE, FALSE, FALSE, FALSE, FALSE, FALSE], "DIO64 Line 4"=[FALSE, FALSE, FALSE, FALSE, FALSE, FALSE, FALSE, FALSE, FALSE, FALSE, FALSE, FALSE, FALSE, FALSE, FALSE, FALSE]}, {"Name"="Pi/2 Pulse 2", "DIO64 Line 1"=[FALSE, FALSE, FALSE, FALSE, FALSE, FALSE, FALSE, FALSE, FALSE, FALSE, FALSE, FALSE, FALSE, FALSE, FALSE, FALSE], "DIO64 Line 2"=[FALSE, FALSE, FALSE, FALSE, FALSE, FALSE, FALSE, FALSE, FALSE, FALSE, FALSE, FALSE, TRUE, FALSE, FALSE, FALSE], "DIO64 Line 3"=[FALSE, FALSE, FALSE, FALSE, FALSE, FALSE, FALSE, FALSE, FALSE, FALSE, FALSE, FALSE, FALSE, FALSE, FALSE, FALSE], "DIO64 Line 4"=[FALSE, FALSE, FALSE, FALSE, FALSE, FALSE, FALSE, FALSE, FALSE, FALSE, FALSE, FALSE, FALSE, FALSE, FALSE, FALSE]}, {"Name"="Scope trigger 2 depletion", "DIO64 Line 1"=[FALSE, FALSE, FALSE, FALSE, FALSE, FALSE, FALSE, FALSE, FALSE, FALSE, FALSE, FALSE, FALSE, FALSE, FALSE, FALSE], "DIO64 Line 2"=[FALSE, FALSE, FALSE, FALSE, FALSE, FALSE, FALSE, FALSE, FALSE, FALSE, FALSE, TRUE, FALSE, FALSE, FALSE, FALSE], "DIO64 Line 3"=[FALSE, FALSE, FALSE, FALSE, FALSE, FALSE, FALSE, FALSE, FALSE, FALSE, FALSE, FALSE, FALSE, FALSE, FALSE, FALSE], "DIO64 Line 4"=[FALSE, FALSE, FALSE, FALSE, FALSE, FALSE, FALSE, FALSE, FALSE, FALSE, FALSE, FALSE, FALSE, FALSE, FALSE, FALSE]}, {"Name"="Chillax", "DIO64 Line 1"=[FALSE, FALSE, FALSE, FALSE, FALSE, FALSE, FALSE, FALSE, FALSE, FALSE, FALSE, FALSE, FALSE, FALSE, FALSE, FALSE], "DIO64 Line 2"=[FALSE, FALSE, FALSE, FALSE, FALSE, FALSE, FALSE, FALSE, FALSE, FALSE, FALSE, FALSE, FALSE, FALSE, FALSE, FALSE], "DIO64 Line 3"=[FALSE, TRUE, FALSE, FALSE, FALSE, FALSE, FALSE, FALSE, FALSE, FALSE, FALSE, FALSE, FALSE, FALSE, FALSE, FALSE], "DIO64 Line 4"=[FALSE, FALSE, FALSE, FALSE, FALSE, FALSE, FALSE, FALSE, FALSE, FALSE, FALSE, FALSE, FALSE, FALSE, FALSE, FALSE]}, {"Name"="Trigger Rotating 2", "DIO64 Line 1"=[FALSE, FALSE, FALSE, FALSE, FALSE, FALSE, FALSE, FALSE, FALSE, FALSE, FALSE, FALSE, FALSE, FALSE, FALSE, FALSE], "DIO64 Line 2"=[TRUE, FALSE, FALSE, FALSE, FALSE, FALSE, FALSE, FALSE, FALSE, FALSE, FALSE, FALSE, FALSE, FALSE, FALSE, FALSE], "DIO64 Line 3"=[FALSE, FALSE, FALSE, FALSE, FALSE, FALSE, FALSE, FALSE, FALSE, FALSE, FALSE, FALSE, FALSE, FALSE, FALSE, FALSE], "DIO64 Line 4"=[FALSE, FALSE, FALSE, FALSE, FALSE, FALSE, FALSE, FALSE, FALSE, FALSE, FALSE, FALSE, FALSE, FALSE, FALSE, FALSE]}, {"Name"="Ramp rotating", "DIO64 Line 1"=[FALSE, FALSE, FALSE, FALSE, FALSE, FALSE, FALSE, FALSE, FALSE, FALSE, FALSE, FALSE, FALSE, FALSE, FALSE, FALSE], "DIO64 Line 2"=[FALSE, FALSE, FALSE, FALSE, FALSE, FALSE, FALSE, FALSE, FALSE, FALSE, TRUE, FALSE, FALSE, FALSE, FALSE, FALSE], "DIO64 Line 3"=[FALSE, FALSE, FALSE, FALSE, FALSE, FALSE, FALSE, FALSE, FALSE, FALSE, FALSE, FALSE, FALSE, FALSE, FALSE, FALSE], "DIO64 Line 4"=[FALSE, FALSE, FALSE, FALSE, FALSE, FALSE, FALSE, FALSE, FALSE, FALSE, FALSE, FALSE, FALSE, FALSE, FALSE, FALSE]}, {"Name"="Squeeze trap", "DIO64 Line 1"=[FALSE, FALSE, FALSE, FALSE, FALSE, FALSE, FALSE, FALSE, FALSE, FALSE, FALSE, FALSE, TRUE, FALSE, FALSE, FALSE], "DIO64 Line 2"=[FALSE, FALSE, FALSE, FALSE, FALSE, FALSE, FALSE, FALSE, FALSE, FALSE, FALSE, FALSE, FALSE, FALSE, FALSE, FALSE], "DIO64 Line 3"=[FALSE, FALSE, FALSE, FALSE, FALSE, FALSE, FALSE, FALSE, FALSE, FALSE, FALSE, FALSE, FALSE, FALSE, FALSE, FALSE], "DIO64 Line 4"=[FALSE, FALSE, FALSE, FALSE, FALSE, FALSE, FALSE, FALSE, FALSE, FALSE, FALSE, FALSE, FALSE, FALSE, FALSE, FALSE]}, {"Name"="Change Toptica Wavelength", "DIO64 Line 1"=[FALSE, FALSE, FALSE, FALSE, FALSE, FALSE, FALSE, FALSE, FALSE, FALSE, FALSE, FALSE, FALSE, FALSE, FALSE, FALSE], "DIO64 Line 2"=[FALSE, FALSE, FALSE, TRUE, FALSE, FALSE, FALSE, FALSE, FALSE, FALSE, FALSE, FALSE, FALSE, FALSE, FALSE, FALSE], "DIO64 Line 3"=[FALSE, FALSE, FALSE, FALSE, FALSE, FALSE, FALSE, FALSE, FALSE, FALSE, FALSE, FALSE, FALSE, FALSE, FALSE, FALSE], "DIO64 Line 4"=[FALSE, FALSE, FALSE, FALSE, FALSE, FALSE, FALSE, FALSE, FALSE, FALSE, FALSE, FALSE, FALSE, FALSE, FALSE, FALSE]}, {"Name"="Disable Topica Lock", "DIO64 Line 1"=[FALSE, FALSE, FALSE, FALSE, FALSE, FALSE, FALSE, FALSE, FALSE, FALSE, FALSE, FALSE, FALSE, FALSE, FALSE, FALSE], "DIO64 Line 2"=[FALSE, FALSE, FALSE, FALSE, FALSE, FALSE, TRUE, FALSE, FALSE, FALSE, FALSE, FALSE, FALSE, FALSE, FALSE, FALSE], "DIO64 Line 3"=[FALSE, FALSE, FALSE, FALSE, FALSE, FALSE, FALSE, FALSE, FALSE, FALSE, FALSE, FALSE, FALSE, FALSE, FALSE, FALSE], "DIO64 Line 4"=[FALSE, FALSE, FALSE, FALSE, FALSE, FALSE, FALSE, FALSE, FALSE, FALSE, FALSE, FALSE, FALSE, FALSE, FALSE, FALSE]}, {"Name"="Microwave On", "DIO64 Line 1"=[FALSE, FALSE, FALSE, FALSE, FALSE, FALSE, FALSE, FALSE, FALSE, FALSE, FALSE, FALSE, FALSE, FALSE, FALSE, FALSE], "DIO64 Line 2"=[FALSE, FALSE, FALSE, FALSE, FALSE, FALSE, FALSE, FALSE, FALSE, FALSE, FALSE, FALSE, FALSE, FALSE, FALSE, FALSE], "DIO64 Line 3"=[FALSE, FALSE, FALSE, FALSE, TRUE, FALSE, FALSE, FALSE, FALSE, FALSE, FALSE, FALSE, FALSE, FALSE, FALSE, FALSE], "DIO64 Line 4"=[FALSE, FALSE, FALSE, FALSE, FALSE, FALSE, FALSE, FALSE, FALSE, FALSE, FALSE, FALSE, FALSE, FALSE, FALSE, FALSE]}, {"Name"="Microwave Sweep", "DIO64 Line 1"=[FALSE, FALSE, FALSE, FALSE, FALSE, FALSE, FALSE, FALSE, FALSE, FALSE, FALSE, FALSE, FALSE, FALSE, FALSE, FALSE], "DIO64 Line 2"=[FALSE, FALSE, FALSE, FALSE, FALSE, FALSE, FALSE, FALSE, FALSE, FALSE, FALSE, FALSE, FALSE, FALSE, FALSE, FALSE], "DIO64 Line 3"=[FALSE, FALSE, FALSE, FALSE, FALSE, TRUE, FALSE, FALSE, FALSE, FALSE, FALSE, FALSE, FALSE, FALSE, FALSE, FALSE], "DIO64 Line 4"=[FALSE, FALSE, FALSE, FALSE, FALSE, FALSE, FALSE, FALSE, FALSE, FALSE, FALSE, FALSE, FALSE, FALSE, FALSE, FALSE]}, {"Name"="Depletion Shutter", "DIO64 Line 1"=[FALSE, FALSE, FALSE, FALSE, FALSE, FALSE, FALSE, FALSE, FALSE, FALSE, FALSE, FALSE, FALSE, FALSE, FALSE, FALSE], "DIO64 Line 2"=[FALSE, FALSE, FALSE, FALSE, FALSE, FALSE, FALSE, TRUE, FALSE, FALSE, FALSE, FALSE, FALSE, FALSE, FALSE, FALSE], "DIO64 Line 3"=[FALSE, FALSE, FALSE, FALSE, FALSE, FALSE, FALSE, FALSE, FALSE, FALSE, FALSE, FALSE, FALSE, FALSE, FALSE, FALSE], "DIO64 Line 4"=[FALSE, FALSE, FALSE, FALSE, FALSE, FALSE, FALSE, FALSE, FALSE, FALSE, FALSE, FALSE, FALSE, FALSE, FALSE, FALSE]}, {"Name"="Depletion Shutter 2", "DIO64 Line 1"=[FALSE, FALSE, FALSE, FALSE, FALSE, FALSE, FALSE, FALSE, FALSE, FALSE, FALSE, FALSE, FALSE, FALSE, FALSE, FALSE], "DIO64 Line 2"=[FALSE, FALSE, FALSE, FALSE, FALSE, FALSE, FALSE, TRUE, FALSE, FALSE, FALSE, FALSE, FALSE, FALSE, FALSE, FALSE], "DIO64 Line 3"=[FALSE, FALSE, FALSE, FALSE, FALSE, FALSE, FALSE, FALSE, FALSE, FALSE, FALSE, FALSE, FALSE, FALSE, FALSE, FALSE], "DIO64 Line 4"=[FALSE, FALSE, FALSE, FALSE, FALSE, FALSE, FALSE, FALSE, FALSE, FALSE, FALSE, FALSE, FALSE, FALSE, FALSE, FALSE]}] caption="DIO64 Tasks"
  out "dio64:channel display":T4={"Channel 1"=[bytes[74], bytes[92], bytes[92], bytes[88], bytes[88], bytes[90], bytes[82], bytes[88], bytes[84], bytes[80], bytes[80], bytes[88], bytes[82], bytes[90], bytes[90], bytes[90]], "Channel 2"=[bytes[86], bytes[86], bytes[86], bytes[100], bytes[86], bytes[88], bytes[90], bytes[90], bytes[92], bytes[86], bytes[88], bytes[86], bytes[86], bytes[86], bytes[88], bytes[92]], "Channel 3"=[bytes[82], bytes[82], bytes[74], bytes[84], bytes[74], bytes[74], bytes[74], bytes[74], bytes[88], bytes[74], bytes[74], bytes[74], bytes[74], bytes[74], bytes[74], bytes[74]], "Channel 4"=[bytes[84], bytes[74], bytes[74], bytes[74], bytes[74], bytes[74], bytes[74], bytes[74], bytes[74], bytes[74], bytes[74], bytes[74], bytes[74], bytes[74], bytes[74], bytes[74]]}
  in  "dio64:chops":cluster{"Chops":u16[]}[](array[cluster])=[{"Chops"=[0, 1]}, {"Chops"=[2, 3]}] caption="Chops"
  in  "dio64:chop labels":string[](array[string])=["Antiphase", "Inphase", "Transfer", "Dissociation", "Not Dissociation", "Fast", "IMG"] caption="DIO64 Chop Labels"
  in  "dio64:channel labels":T5(array[cluster])=[[{"Channel"="A00:", "Name"="", "plot"=FALSE}, {"Channel"="B00:", "Name"="DDS Ramp 0-1", "plot"=TRUE}, {"Channel"="C00:", "Name"="Unrelax", "plot"=TRUE}, {"Channel"="D00:", "Name"="I/O Update", "plot"=FALSE}], [{"Channel"="A01:", "Name"="Stella AOM shutter", "plot"=FALSE}, {"Channel"="B01:", "Name"="Cora Shutter", "plot"=FALSE}, {"Channel"="C01:", "Name"="Chillax", "plot"=TRUE}, {"Channel"="D01:", "Name"="", "plot"=FALSE}], [{"Channel"="A02:", "Name"="Depletion shutter", "plot"=FALSE}, {"Channel"="B02:", "Name"="DDS Ramp 2-3", "plot"=FALSE}, {"Channel"="C02:", "Name"="", "plot"=FALSE}, {"Channel"="D02:", "Name"="", "plot"=FALSE}], [{"Channel"="A03:", "Name"="Abby Flashlamp", "plot"=FALSE}, {"Channel"="B03:", "Name"="Toptica wavelength switch", "plot"=TRUE}, {"Channel"="C03:", "Name"="Trap Gate", "plot"=FALSE}, {"Channel"="D03:", "Name"="", "plot"=FALSE}], [{"Channel"="A04:", "Name"="Abby Q-Switch", "plot"=FALSE}, {"Channel"="B04:", "Name"="End Cap SW0", "plot"=FALSE}, {"Channel"="C04:", "Name"="", "plot"=FALSE}, {"Channel"="D04:", "Name"="", "plot"=FALSE}], [{"Channel"="A05:", "Name"="Img MCP Trigger", "plot"=FALSE}, {"Channel"="B05:", "Name"="266nm Shutter", "plot"=TRUE}, {"Channel"="C05:", "Name"="", "plot"=FALSE}, {"Channel"="D05:", "Name"="", "plot"=FALSE}], [{"Channel"="A06:", "Name"="Trap DDS", "plot"=TRUE}, {"Channel"="B06:", "Name"="B field switch 1", "plot"=FALSE}, {"Channel"="C06:", "Name"="", "plot"=FALSE}, {"Channel"="D06:", "Name"="", "plot"=FALSE}], [{"Channel"="A07:", "Name"="Trigger Scope", "plot"=FALSE}, {"Channel"="B07:", "Name"="B field switch 2", "plot"=FALSE}, {"Channel"="C07:", "Name"="", "plot"=FALSE}, {"Channel"="D07:", "Name"="", "plot"=FALSE}], [{"Channel"="A08:", "Name"="Cora Scan", "plot"=FALSE}, {"Channel"="B08:", "Name"="Trigger Depletion", "plot"=TRUE}, {"Channel"="C08:", "Name"="Far align tool", "plot"=FALSE}, {"Channel"="D08:", "Name"="", "plot"=FALSE}], [{"Channel"="A09:", "Name"="DAC A0", "plot"=FALSE}, {"Channel"="B09:", "Name"="Trigger DAC", "plot"=FALSE}, {"Channel"="C09:", "Name"="", "plot"=FALSE}, {"Channel"="D09:", "Name"="", "plot"=FALSE}], [{"Channel"="A10:", "Name"="DAC A1", "plot"=FALSE}, {"Channel"="B10:", "Name"="DDS Ramp 8-9 ", "plot"=TRUE}, {"Channel"="C10:", "Name"="", "plot"=FALSE}, {"Channel"="D10:", "Name"="", "plot"=FALSE}], [{"Channel"="A11:", "Name"="Toptica Switch", "plot"=TRUE}, {"Channel"="B11:", "Name"="Bertha Scan", "plot"=FALSE}, {"Channel"="C11:", "Name"="", "plot"=FALSE}, {"Channel"="D11:", "Name"="", "plot"=FALSE}], [{"Channel"="A12:", "Name"="End Ramp", "plot"=TRUE}, {"Channel"="B12:", "Name"="DDS Ramp 6-7", "plot"=TRUE}, {"Channel"="C12:", "Name"="", "plot"=FALSE}, {"Channel"="D12:", "Name"="", "plot"=FALSE}], [{"Channel"="A13:", "Name"="Jessica Shutter", "plot"=FALSE}, {"Channel"="B13:", "Name"="End Cap SW1", "plot"=FALSE}, {"Channel"="C13:", "Name"="", "plot"=FALSE}, {"Channel"="D13:", "Name"="", "plot"=FALSE}], [{"Channel"="A14:", "Name"="Gas Pulse Valve", "plot"=FALSE}, {"Channel"="B14:", "Name"="Stella Switch", "plot"=TRUE}, {"Channel"="C14:", "Name"="", "plot"=FALSE}, {"Channel"="D14:", "Name"="", "plot"=FALSE}], [{"Channel"="A15:", "Name"="MCP Framegrabber", "plot"=FALSE}, {"Channel"="B15:", "Name"="Bertha UV Shutter", "plot"=TRUE}, {"Channel"="C15:", "Name"="", "plot"=FALSE}, {"Channel"="D15:", "Name"="", "plot"=FALSE}]] caption="DIO64 Channel Labels"
  in  "dio64:display chop":u32(ring)=5 caption="Display Chop"
  in  "dio64:update display":bool caption="update"
  out "dio64:timing graph":cluster{dbl[], dbl[]}[](graph)=[{[0.0, 0.17220000000000013, 18.1746, 18.1846, 19.1722, 19.1822, 19.28709999999999, 19.288099999999993, 19.297099999999993, 19.333099999999995, 19.41219999999999, 19.422199999999993, 20.1312, 20.1712, 20.1722, 31.1722, 32.172200000000004, 100.1722, 112.1722, 112.18220000000001, 117.1722, 120.1722, 130.1722, 130.1822, 133.1722, 138.1722, 139.1222, 395.12219999999996, 396.07219999999995, 398.2922, 402.07219999999995, 402.07419999999996, 405.07219999999995, 405.07419999999996, 411.2922, 412.2922, 412.30219999999997, 418.2922, 418.30219999999997, 451.62219999999996, 451.6322, 484.9622, 484.9722, 502.36721, 502.37721, 505.07219999999995, 518.2922, 518.3022, 520.2922, 520.2972, 520.3022, 520.3072, 520.3172, 520.36721, 520.37721, 521.2922], [0.0, 0.0, 0.0, 0.0, 0.0, 0.0, 0.0, 0.0, 0.0, 0.0, 0.0, 0.0, 0.0, 0.0, 1.0, 1.0, 1.0, 1.0, 1.0, 1.0, 1.0, 1.0, 1.0, 1.0, 1.0, 1.0, 1.0, 1.0, 1.0, 1.0, 1.0, 1.0, 1.0, 1.0, 1.0, 1.0, 1.0, 1.0, 1.0, 1.0, 1.0, 1.0, 1.0, 1.0, 1.0, 1.0, 1.0, 1.0, 0.0, 0.0, 0.0, 0.0, 0.0, 0.0, 0.0, 0.0]}, {[0.0, 0.17220000000000013, 18.1746, 18.1846, 19.1722, 19.1822, 19.28709999999999, 19.288099999999993, 19.297099999999993, 19.333099999999995, 19.41219999999999, 19.422199999999993, 20.1312, 20.1712, 20.1722, 31.1722, 32.172200000000004, 100.1722, 112.1722, 112.18220000000001, 117.1722, 120.1722, 130.1722, 130.1822, 133.1722, 138.1722, 139.1222, 395.12219999999996, 396.07219999999995, 398.2922, 402.07219999999995, 402.07419999999996, 405.07219999999995, 405.07419999999996, 411.2922, 412.2922, 412.30219999999997, 418.2922, 418.30219999999997, 451.62219999999996, 451.6322, 484.9622, 484.9722, 502.36721, 502.37721, 505.07219999999995, 518.2922, 518.3022, 520.2922, 520.2972, 520.3022, 520.3072, 520.3172, 520.36721, 520.37721, 521.2922], [-1.2, -1.2, -1.2, -1.2, -1.2, -1.2, -1.2, -1.2, -1.2, -1.2, -1.2, -1.2, -1.2, -1.2, -1.2, -1.2, -1.2, -1.2, -1.2, -1.2, -1.2, -1.2, -1.2, -1.2, -1.2, -1.2, -1.2, -1.2, -1.2, -1.2, -1.2, -1.2, -1.2, -1.2, -1.2, -1.2, -1.2, -1.2, -1.2, -1.2, -1.2, -1.2, -1.2, -1.2, -1.2, -1.2, -1.2, -1.2, -1.2, -1.2, -1.2, -1.2, -1.2, -1.2, -1.2, -1.2]}, {[0.0, 0.17220000000000013, 18.1746, 18.1846, 19.1722, 19.1822, 19.28709999999999, 19.288099999999993, 19.297099999999993, 19.333099999999995, 19.41219999999999, 19.422199999999993, 20.1312, 20.1712, 20.1722, 31.1722, 32.172200000000004, 100.1722, 112.1722, 112.18220000000001, 117.1722, 120.1722, 130.1722, 130.1822, 133.1722, 138.1722, 139.1222, 395.12219999999996, 396.07219999999995, 398.2922, 402.07219999999995, 402.07419999999996, 405.07219999999995, 405.07419999999996, 411.2922, 412.2922, 412.30219999999997, 418.2922, 418.30219999999997, 451.62219999999996, 451.6322, 484.9622, 484.9722, 502.36721, 502.37721, 505.07219999999995, 518.2922, 518.3022, 520.2922, 520.2972, 520.3022, 520.3072, 520.3172, 520.36721, 520.37721, 521.2922], [-2.4, -2.4, -2.4, -2.4, -2.4, -2.4, -2.4, -2.4, -2.4, -2.4, -2.4, -2.4, -2.4, -2.4, -2.4, -2.4, -2.4, -2.4, -2.4, -2.4, -2.4, -2.4, -2.4, -2.4, -2.4, -2.4, -2.4, -2.4, -2.4, -2.4, -2.4, -2.4, -2.4, -2.4, -2.4, -2.4, -2.4, -2.4, -2.4, -2.4, -2.4, -2.4, -2.4, -2.4, -2.4, -2.4, -2.4, -2.4, -2.4, -2.4, -2.4, -2.4, -2.4, -2.4, -2.4, -2.4]}, {[0.0, 0.17220000000000013, 18.1746, 18.1846, 19.1722, 19.1822, 19.28709999999999, 19.288099999999993, 19.297099999999993, 19.333099999999995, 19.41219999999999, 19.422199999999993, 20.1312, 20.1712, 20.1722, 31.1722, 32.172200000000004, 100.1722, 112.1722, 112.18220000000001, 117.1722, 120.1722, 130.1722, 130.1822, 133.1722, 138.1722, 139.1222, 395.12219999999996, 396.07219999999995, 398.2922, 402.07219999999995, 402.07419999999996, 405.07219999999995, 405.07419999999996, 411.2922, 412.2922, 412.30219999999997, 418.2922, 418.30219999999997, 451.62219999999996, 451.6322, 484.9622, 484.9722, 502.36721, 502.37721, 505.07219999999995, 518.2922, 518.3022, 520.2922, 520.2972, 520.3022, 520.3072, 520.3172, 520.36721, 520.37721, 521.2922], [-3.5999999999999996, -3.5999999999999996, -3.5999999999999996, -3.5999999999999996, -3.5999999999999996, -3.5999999999999996, -3.5999999999999996, -3.5999999999999996, -3.5999999999999996, -3.5999999999999996, -3.5999999999999996, -3.5999999999999996, -3.5999999999999996, -3.5999999999999996, -3.5999999999999996, -3.5999999999999996, -3.5999999999999996, -3.5999999999999996, -3.5999999999999996, -3.5999999999999996, -3.5999999999999996, -3.5999999999999996, -3.5999999999999996, -3.5999999999999996, -3.5999999999999996, -3.5999999999999996, -3.5999999999999996, -3.5999999999999996, -3.5999999999999996, -3.5999999999999996, -3.5999999999999996, -3.5999999999999996, -3.5999999999999996, -3.5999999999999996, -3.5999999999999996, -3.5999999999999996, -3.5999999999999996, -3.5999999999999996, -3.5999999999999996, -3.5999999999999996, -3.5999999999999996, -3.5999999999999996, -3.5999999999999996, -3.5999999999999996, -3.5999999999999996, -3.5999999999999996, -3.5999999999999996, -3.5999999999999996, -3.5999999999999996, -3.5999999999999996, -3.5999999999999996, -3.5999999999999996, -3.5999999999999996, -3.5999999999999996, -3.5999999999999996, -3.5999999999999996]}, {[0.0, 0.17220000000000013, 18.1746, 18.1846, 19.1722, 19.1822, 19.28709999999999, 19.288099999999993, 19.297099999999993, 19.333099999999995, 19.41219999999999, 19.422199999999993, 20.1312, 20.1712, 20.1722, 31.1722, 32.172200000000004, 100.1722, 112.1722, 112.18220000000001, 117.1722, 120.1722, 130.1722, 130.1822, 133.1722, 138.1722, 139.1222, 395.12219999999996, 396.07219999999995, 398.2922, 402.07219999999995, 402.07419999999996, 405.07219999999995, 405.07419999999996, 411.2922, 412.2922, 412.30219999999997, 418.2922, 418.30219999999997, 451.62219999999996, 451.6322, 484.9622, 484.9722, 502.36721, 502.37721, 505.07219999999995, 518.2922, 518.3022, 520.2922, 520.2972, 520.3022, 520.3072, 520.3172, 520.36721, 520.37721, 521.2922], [-4.8, -4.8, -4.8, -4.8, -4.8, -4.8, -4.8, -4.8, -4.8, -4.8, -4.8, -4.8, -4.8, -4.8, -4.8, -4.8, -4.8, -4.8, -4.8, -4.8, -4.8, -4.8, -4.8, -4.8, -4.8, -4.8, -4.8, -4.8, -4.8, -4.8, -4.8, -4.8, -4.8, -4.8, -4.8, -4.8, -4.8, -4.8, -4.8, -4.8, -4.8, -4.8, -4.8, -4.8, -4.8, -4.8, -4.8, -4.8, -4.8, -4.8, -4.8, -4.8, -4.8, -4.8, -4.8, -4.8]}, {[0.0, 0.17220000000000013, 18.1746, 18.1846, 19.1722, 19.1822, 19.28709999999999, 19.288099999999993, 19.297099999999993, 19.333099999999995, 19.41219999999999, 19.422199999999993, 20.1312, 20.1712, 20.1722, 31.1722, 32.172200000000004, 100.1722, 112.1722, 112.18220000000001, 117.1722, 120.1722, 130.1722, 130.1822, 133.1722, 138.1722, 139.1222, 395.12219999999996, 396.07219999999995, 398.2922, 402.07219999999995, 402.07419999999996, 405.07219999999995, 405.07419999999996, 411.2922, 412.2922, 412.30219999999997, 418.2922, 418.30219999999997, 451.62219999999996, 451.6322, 484.9622, 484.9722, 502.36721, 502.37721, 505.07219999999995, 518.2922, 518.3022, 520.2922, 520.2972, 520.3022, 520.3072, 520.3172, 520.36721, 520.37721, 521.2922], [-6.0, -6.0, -6.0, -6.0, -6.0, -6.0, -6.0, -6.0, -6.0, -6.0, -6.0, -6.0, -6.0, -6.0, -6.0, -6.0, -6.0, -6.0, -6.0, -6.0, -6.0, -6.0, -6.0, -6.0, -6.0, -6.0, -6.0, -6.0, -6.0, -6.0, -6.0, -6.0, -6.0, -6.0, -6.0, -6.0, -6.0, -6.0, -6.0, -6.0, -6.0, -6.0, -6.0, -6.0, -6.0, -6.0, -6.0, -6.0, -6.0, -6.0, -6.0, -6.0, -6.0, -6.0, -6.0, -6.0]}, {[0.0, 0.17220000000000013, 18.1746, 18.1846, 19.1722, 19.1822, 19.28709999999999, 19.288099999999993, 19.297099999999993, 19.333099999999995, 19.41219999999999, 19.422199999999993, 20.1312, 20.1712, 20.1722, 31.1722, 32.172200000000004, 100.1722, 112.1722, 112.18220000000001, 117.1722, 120.1722, 130.1722, 130.1822, 133.1722, 138.1722, 139.1222, 395.12219999999996, 396.07219999999995, 398.2922, 402.07219999999995, 402.07419999999996, 405.07219999999995, 405.07419999999996, 411.2922, 412.2922, 412.30219999999997, 418.2922, 418.30219999999997, 451.62219999999996, 451.6322, 484.9622, 484.9722, 502.36721, 502.37721, 505.07219999999995, 518.2922, 518.3022, 520.2922, 520.2972, 520.3022, 520.3072, 520.3172, 520.36721, 520.37721, 521.2922], [-7.2, -7.2, -7.2, -7.2, -7.2, -7.2, -7.2, -7.2, -7.2, -7.2, -7.2, -7.2, -7.2, -7.2, -7.2, -7.2, -7.2, -7.2, -7.2, -7.2, -7.2, -7.2, -7.2, -7.2, -7.2, -7.2, -7.2, -7.2, -7.2, -7.2, -7.2, -7.2, -7.2, -7.2, -7.2, -7.2, -7.2, -7.2, -7.2, -7.2, -7.2, -7.2, -7.2, -7.2, -7.2, -7.2, -7.2, -7.2, -7.2, -7.2, -7.2, -7.2, -7.2, -7.2, -7.2, -7.2]}, {[0.0, 0.17220000000000013, 18.1746, 18.1846, 19.1722, 19.1822, 19.28709999999999, 19.288099999999993, 19.297099999999993, 19.333099999999995, 19.41219999999999, 19.422199999999993, 20.1312, 20.1712, 20.1722, 31.1722, 32.172200000000004, 100.1722, 112.1722, 112.18220000000001, 117.1722, 120.1722, 130.1722, 130.1822, 133.1722, 138.1722, 139.1222, 395.12219999999996, 396.07219999999995, 398.2922, 402.07219999999995, 402.07419999999996, 405.07219999999995, 405.07419999999996, 411.2922, 412.2922, 412.30219999999997, 418.2922, 418.30219999999997, 451.62219999999996, 451.6322, 484.9622, 484.9722, 502.36721, 502.37721, 505.07219999999995, 518.2922, 518.3022, 520.2922, 520.2972, 520.3022, 520.3072, 520.3172, 520.36721, 520.37721, 521.2922], [-8.4, -8.4, -8.4, -8.4, -8.4, -8.4, -8.4, -8.4, -8.4, -8.4, -8.4, -8.4, -8.4, -8.4, -8.4, -8.4, -8.4, -8.4, -8.4, -8.4, -8.4, -8.4, -8.4, -8.4, -8.4, -8.4, -8.4, -8.4, -8.4, -8.4, -8.4, -8.4, -8.4, -8.4, -8.4, -8.4, -8.4, -8.4, -8.4, -8.4, -8.4, -8.4, -8.4, -8.4, -8.4, -8.4, -8.4, -8.4, -8.4, -8.4, -8.4, -8.4, -8.4, -8.4, -8.4, -8.4]}, {[0.0, 0.17220000000000013, 18.1746, 18.1846, 19.1722, 19.1822, 19.28709999999999, 19.288099999999993, 19.297099999999993, 19.333099999999995, 19.41219999999999, 19.422199999999993, 20.1312, 20.1712, 20.1722, 31.1722, 32.172200000000004, 100.1722, 112.1722, 112.18220000000001, 117.1722, 120.1722, 130.1722, 130.1822, 133.1722, 138.1722, 139.1222, 395.12219999999996, 396.07219999999995, 398.2922, 402.07219999999995, 402.07419999999996, 405.07219999999995, 405.07419999999996, 411.2922, 412.2922, 412.30219999999997, 418.2922, 418.30219999999997, 451.62219999999996, 451.6322, 484.9622, 484.9722, 502.36721, 502.37721, 505.07219999999995, 518.2922, 518.3022, 520.2922, 520.2972, 520.3022, 520.3072, 520.3172, 520.36721, 520.37721, 521.2922], [-9.6, -9.6, -9.6, -9.6, -9.6, -9.6, -9.6, -9.6, -9.6, -9.6, -9.6, -9.6, -9.6, -9.6, -9.6, -9.6, -9.6, -9.6, -9.6, -9.6, -9.6, -9.6, -9.6, -9.6, -9.6, -9.6, -9.6, -9.6, -9.6, -9.6, -9.6, -9.6, -9.6, -9.6, -9.6, -9.6, -9.6, -9.6, -9.6, -9.6, -9.6, -9.6, -9.6, -9.6, -9.6, -9.6, -9.6, -9.6, -9.6, -9.6, -9.6, -9.6, -9.6, -9.6, -9.6, -9.6]}, {[0.0, 0.17220000000000013, 18.1746, 18.1846, 19.1722, 19.1822, 19.28709999999999, 19.288099999999993, 19.297099999999993, 19.333099999999995, 19.41219999999999, 19.422199999999993, 20.1312, 20.1712, 20.1722, 31.1722, 32.172200000000004, 100.1722, 112.1722, 112.18220000000001, 117.1722, 120.1722, 130.1722, 130.1822, 133.1722, 138.1722, 139.1222, 395.12219999999996, 396.07219999999995, 398.2922, 402.07219999999995, 402.07419999999996, 405.07219999999995, 405.07419999999996, 411.2922, 412.2922, 412.30219999999997, 418.2922, 418.30219999999997, 451.62219999999996, 451.6322, 484.9622, 484.9722, 502.36721, 502.37721, 505.07219999999995, 518.2922, 518.3022, 520.2922, 520.2972, 520.3022, 520.3072, 520.3172, 520.36721, 520.37721, 521.2922], [-10.799999999999999, -10.799999999999999, -10.799999999999999, -10.799999999999999, -10.799999999999999, -10.799999999999999, -10.799999999999999, -10.799999999999999, -10.799999999999999, -10.799999999999999, -10.799999999999999, -10.799999999999999, -10.799999999999999, -10.799999999999999, -10.799999999999999, -10.799999999999999, -10.799999999999999, -10.799999999999999, -10.799999999999999, -10.799999999999999, -10.799999999999999, -10.799999999999999, -10.799999999999999, -10.799999999999999, -10.799999999999999, -10.799999999999999, -10.799999999999999, -10.799999999999999, -10.799999999999999, -10.799999999999999, -10.799999999999999, -10.799999999999999, -10.799999999999999, -10.799999999999999, -10.799999999999999, -10.799999999999999, -10.799999999999999, -10.799999999999999, -10.799999999999999, -10.799999999999999, -10.799999999999999, -10.799999999999999, -10.799999999999999, -10.799999999999999, -10.799999999999999, -10.799999999999999, -10.799999999999999, -10.799999999999999, -10.799999999999999, -10.799999999999999, -10.799999999999999, -10.799999999999999, -10.799999999999999, -10.799999999999999, -10.799999999999999, -10.799999999999999]}, {[0.0, 0.17220000000000013, 18.1746, 18.1846, 19.1722, 19.1822, 19.28709999999999, 19.288099999999993, 19.297099999999993, 19.333099999999995, 19.41219999999999, 19.422199999999993, 20.1312, 20.1712, 20.1722, 31.1722, 32.172200000000004, 100.1722, 112.1722, 112.18220000000001, 117.1722, 120.1722, 130.1722, 130.1822, 133.1722, 138.1722, 139.1222, 395.12219999999996, 396.07219999999995, 398.2922, 402.07219999999995, 402.07419999999996, 405.07219999999995, 405.07419999999996, 411.2922, 412.2922, 412.30219999999997, 418.2922, 418.30219999999997, 451.62219999999996, 451.6322, 484.9622, 484.9722, 502.36721, 502.37721, 505.07219999999995, 518.2922, 518.3022, 520.2922, 520.2972, 520.3022, 520.3072, 520.3172, 520.36721, 520.37721, 521.2922], [-11.999999999999998, -10.999999999999998, -10.999999999999998, -10.999999999999998, -10.999999999999998, -10.999999999999998, -10.999999999999998, -10.999999999999998, -10.999999999999998, -10.999999999999998, -10.999999999999998, -10.999999999999998, -10.999999999999998, -10.999999999999998, -10.999999999999998, -10.999999999999998, -10.999999999999998, -11.999999999999998, -11.999999999999998, -11.999999999999998, -11.999999999999998, -11.999999999999998, -11.999999999999998, -11.999999999999998, -11.999999999999998, -11.999999999999998, -11.999999999999998, -11.999999999999998, -11.999999999999998, -11.999999999999998, -11.999999999999998, -11.999999999999998, -11.999999999999998, -11.999999999999998, -11.999999999999998, -11.999999999999998, -11.999999999999998, -11.999999999999998, -11.999999999999998, -11.999999999999998, -11.999999999999998, -11.999999999999998, -11.999999999999998, -11.999999999999998, -11.999999999999998, -11.999999999999998, -11.999999999999998, -11.999999999999998, -11.999999999999998, -11.999999999999998, -11.999999999999998, -11.999999999999998, -11.999999999999998, -11.999999999999998, -11.999999999999998, -11.999999999999998]}, {[0.0, 0.17220000000000013, 18.1746, 18.1846, 19.1722, 19.1822, 19.28709999999999, 19.288099999999993, 19.297099999999993, 19.333099999999995, 19.41219999999999, 19.422199999999993, 20.1312, 20.1712, 20.1722, 31.1722, 32.172200000000004, 100.1722, 112.1722, 112.18220000000001, 117.1722, 120.1722, 130.1722, 130.1822, 133.1722, 138.1722, 139.1222, 395.12219999999996, 396.07219999999995, 398.2922, 402.07219999999995, 402.07419999999996, 405.07219999999995, 405.07419999999996, 411.2922, 412.2922, 412.30219999999997, 418.2922, 418.30219999999997, 451.62219999999996, 451.6322, 484.9622, 484.9722, 502.36721, 502.37721, 505.07219999999995, 518.2922, 518.3022, 520.2922, 520.2972, 520.3022, 520.3072, 520.3172, 520.36721, 520.37721, 521.2922], [-13.199999999999998, -13.199999999999998, -13.199999999999998, -13.199999999999998, -13.199999999999998, -13.199999999999998, -13.199999999999998, -13.199999999999998, -13.199999999999998, -13.199999999999998, -13.199999999999998, -13.199999999999998, -13.199999999999998, -13.199999999999998, -13.199999999999998, -13.199999999999998, -13.199999999999998, -13.199999999999998, -13.199999999999998, -13.199999999999998, -13.199999999999998, -13.199999999999998, -13.199999999999998, -13.199999999999998, -13.199999999999998, -13.199999999999998, -13.199999999999998, -13.199999999999998, -13.199999999999998, -13.199999999999998, -13.199999999999998, -13.199999999999998, -13.199999999999998, -13.199999999999998, -13.199999999999998, -13.199999999999998, -13.199999999999998, -13.199999999999998, -13.199999999999998, -13.199999999999998, -13.199999999999998, -13.199999999999998, -13.199999999999998, -13.199999999999998, -13.199999999999998, -13.199999999999998, -13.199999999999998, -13.199999999999998, -13.199999999999998, -13.199999999999998, -13.199999999999998, -13.199999999999998, -13.199999999999998, -13.199999999999998, -13.199999999999998, -13.199999999999998]}, {[0.0, 0.17220000000000013, 18.1746, 18.1846, 19.1722, 19.1822, 19.28709999999999, 19.288099999999993, 19.297099999999993, 19.333099999999995, 19.41219999999999, 19.422199999999993, 20.1312, 20.1712, 20.1722, 31.1722, 32.172200000000004, 100.1722, 112.1722, 112.18220000000001, 117.1722, 120.1722, 130.1722, 130.1822, 133.1722, 138.1722, 139.1222, 395.12219999999996, 396.07219999999995, 398.2922, 402.07219999999995, 402.07419999999996, 405.07219999999995, 405.07419999999996, 411.2922, 412.2922, 412.30219999999997, 418.2922, 418.30219999999997, 451.62219999999996, 451.6322, 484.9622, 484.9722, 502.36721, 502.37721, 505.07219999999995, 518.2922, 518.3022, 520.2922, 520.2972, 520.3022, 520.3072, 520.3172, 520.36721, 520.37721, 521.2922], [-14.399999999999997, -14.399999999999997, -14.399999999999997, -14.399999999999997, -13.399999999999997, -14.399999999999997, -14.399999999999997, -14.399999999999997, -14.399999999999997, -14.399999999999997, -14.399999999999997, -14.399999999999997, -14.399999999999997, -14.399999999999997, -14.399999999999997, -14.399999999999997, -14.399999999999997, -14.399999999999997, -14.399999999999997, -14.399999999999997, -14.399999999999997, -14.399999999999997, -14.399999999999997, -14.399999999999997, -14.399999999999997, -14.399999999999997, -14.399999999999997, -14.399999999999997, -14.399999999999997, -14.399999999999997, -14.399999999999997, -14.399999999999997, -14.399999999999997, -14.399999999999997, -14.399999999999997, -14.399999999999997, -14.399999999999997, -14.399999999999997, -14.399999999999997, -14.399999999999997, -14.399999999999997, -14.399999999999997, -14.399999999999997, -14.399999999999997, -14.399999999999997, -14.399999999999997, -14.399999999999997, -14.399999999999997, -14.399999999999997, -14.399999999999997, -14.399999999999997, -14.399999999999997, -14.399999999999997, -14.399999999999997, -14.399999999999997, -14.399999999999997]}]
  in  "dio64:override":T6={"DIO64 Line 1"=[FALSE, FALSE, FALSE, FALSE, FALSE, FALSE, FALSE, FALSE, FALSE, FALSE, FALSE, FALSE, FALSE, FALSE, FALSE, FALSE], "DIO64 Line 2"=[FALSE, FALSE, FALSE, FALSE, FALSE, FALSE, TRUE, FALSE, FALSE, FALSE, FALSE, FALSE, FALSE, FALSE, FALSE, FALSE], "DIO64 Line 3"=[FALSE, FALSE, FALSE, FALSE, FALSE, FALSE, FALSE, FALSE, FALSE, FALSE, FALSE, FALSE, FALSE, FALSE, FALSE, FALSE], "DIO64 Line 4"=[FALSE, FALSE, FALSE, FALSE, FALSE, FALSE, FALSE, FALSE, FALSE, FALSE, FALSE, FALSE, FALSE, FALSE, FALSE, FALSE]} caption="DIO64 Override"
  out "dio64:debug2":T7(array[cluster])=[{"Task"="T0", "begin time"=0.0, "end time"=0.0, "Chops"=[FALSE, FALSE, FALSE, FALSE, FALSE, FALSE, FALSE, FALSE, FALSE, FALSE, FALSE]}, {"Task"="Bertha UV Shutter", "begin time"=0.17220000000000013, "end time"=100.1722, "Chops"=[FALSE, FALSE, FALSE, FALSE, FALSE, FALSE, FALSE, FALSE, FALSE, FALSE, FALSE, FALSE]}, {"Task"="Jessica Shutter", "begin time"=0.17220000000000013, "end time"=100.1722, "Chops"=[FALSE, FALSE, FALSE, FALSE, FALSE, FALSE, FALSE, FALSE, FALSE, FALSE, FALSE, FALSE]}, {"Task"="IOUpdate", "begin time"=18.1746, "end time"=18.1846, "Chops"=[FALSE, FALSE, FALSE, FALSE, FALSE, FALSE, FALSE, FALSE, FALSE, FALSE, FALSE, FALSE]}, {"Task"="Chillax", "begin time"=19.1722, "end time"=19.1822, "Chops"=[FALSE, FALSE, FALSE, FALSE, FALSE, FALSE, FALSE, FALSE, FALSE, FALSE, FALSE, FALSE]}, {"Task"="Trigger DAC", "begin time"=19.1722, "end time"=19.1822, "Chops"=[FALSE, FALSE, FALSE, FALSE, FALSE, FALSE, FALSE, FALSE, FALSE, FALSE, FALSE, FALSE]}, {"Task"="Abby Flashlamp", "begin time"=19.28709999999999, "end time"=19.297099999999993, "Chops"=[FALSE, FALSE, FALSE, FALSE, FALSE, FALSE, FALSE, FALSE, FALSE, FALSE, FALSE, FALSE]}, {"Task"="Gas Pulse", "begin time"=19.288099999999993, "end time"=19.333099999999995, "Chops"=[FALSE, FALSE, FALSE, FALSE, FALSE, FALSE, FALSE, FALSE, FALSE, FALSE, FALSE, FALSE]}, {"Task"="Abby Q-switch", "begin time"=19.41219999999999, "end time"=19.422199999999993, "Chops"=[FALSE, FALSE, FALSE, FALSE, FALSE, FALSE, FALSE, FALSE, FALSE, FALSE, FALSE, FALSE]}, {"Task"="Zero DAC", "begin time"=20.1312, "end time"=20.1712, "Chops"=[FALSE, FALSE, FALSE, FALSE, FALSE, FALSE, FALSE, FALSE, FALSE, FALSE, FALSE, FALSE]}, {"Task"="Stop Ions", "begin time"=20.1712, "end time"=20.1722, "Chops"=[FALSE, FALSE, FALSE, FALSE, FALSE, FALSE, FALSE, FALSE, FALSE, FALSE, FALSE, FALSE]}, {"Task"="Trap", "begin time"=20.1722, "end time"=520.2922, "Chops"=[FALSE, FALSE, FALSE, FALSE, FALSE, FALSE, FALSE, FALSE, FALSE, FALSE, FALSE, FALSE]}, {"Task"="DDS Ramp 1", "begin time"=31.1722, "end time"=411.2922, "Chops"=[FALSE, FALSE, FALSE, FALSE, TRUE, TRUE, TRUE, FALSE, FALSE, FALSE, FALSE, FALSE]}, {"Task"="Stella Fiber Switch", "begin time"=32.172200000000004, "end time"=112.1722, "Chops"=[FALSE, FALSE, FALSE, TRUE, TRUE, TRUE, TRUE, FALSE, FALSE, FALSE, FALSE, FALSE]}, {"Task"="Toptica Fiber Switch", "begin time"=32.172200000000004, "end time"=117.1722, "Chops"=[FALSE, FALSE, FALSE, TRUE, TRUE, TRUE, TRUE, FALSE, FALSE, FALSE, FALSE, FALSE]}, {"Task"="Scope trigger 2 transfer", "begin time"=112.1722, "end time"=112.18220000000001, "Chops"=[TRUE, TRUE, FALSE, TRUE, TRUE, TRUE, TRUE, FALSE, FALSE, FALSE, FALSE, FALSE]}, {"Task"="Change Toptica Wavelength", "begin time"=120.1722, "end time"=505.07219999999995, "Chops"=[FALSE, FALSE, FALSE, FALSE, TRUE, TRUE, TRUE, FALSE, FALSE, FALSE, FALSE, FALSE]}, {"Task"="Scope trigger 2 depletion", "begin time"=130.1722, "end time"=130.1822, "Chops"=[FALSE, FALSE, TRUE, TRUE, TRUE, TRUE, TRUE, FALSE, FALSE, FALSE, FALSE, FALSE]}, {"Task"="Trigger Depletion", "begin time"=130.1722, "end time"=133.1722, "Chops"=[FALSE, FALSE, TRUE, TRUE, TRUE, TRUE, TRUE, FALSE, FALSE, FALSE, FALSE, FALSE]}, {"Task"="Pi/2 Pulse", "begin time"=138.1722, "end time"=139.1222, "Chops"=[FALSE, FALSE, FALSE, FALSE, TRUE, TRUE, TRUE, FALSE, FALSE, FALSE, FALSE, FALSE]}, {"Task"="Pi/2 Pulse 2", "begin time"=395.12219999999996, "end time"=396.07219999999995, "Chops"=[FALSE, FALSE, FALSE, FALSE, TRUE, TRUE, TRUE, FALSE, FALSE, FALSE, FALSE, FALSE]}, {"Task"="266nm Shutter", "begin time"=398.2922, "end time"=521.2922, "Chops"=[FALSE, FALSE, FALSE, FALSE, FALSE, TRUE, TRUE, FALSE, FALSE, FALSE, FALSE, FALSE]}, {"Task"="Cora Shutter", "begin time"=398.2922, "end time"=521.2922, "Chops"=[FALSE, FALSE, FALSE, FALSE, TRUE, TRUE, TRUE, FALSE, FALSE, FALSE, FALSE, FALSE]}, {"Task"="Trigger Depletion 2", "begin time"=402.07219999999995, "end time"=405.07219999999995, "Chops"=[TRUE, FALSE, TRUE, TRUE, TRUE, TRUE, TRUE, FALSE, FALSE, FALSE, FALSE, FALSE]}, {"Task"="Trigger Depletion 2-dephase", "begin time"=402.07419999999996, "end time"=405.07419999999996, "Chops"=[FALSE, TRUE, TRUE, TRUE, TRUE, TRUE, TRUE, FALSE, FALSE, FALSE, FALSE, FALSE]}, {"Task"="Unchillax", "begin time"=412.2922, "end time"=412.30219999999997, "Chops"=[FALSE, FALSE, FALSE, FALSE, FALSE, TRUE, TRUE, FALSE, FALSE, FALSE, FALSE, FALSE]}, {"Task"="End Ramp", "begin time"=418.2922, "end time"=418.30219999999997, "Chops"=[FALSE, FALSE, FALSE, FALSE, FALSE, TRUE, TRUE, FALSE, FALSE, FALSE, FALSE, FALSE]}, {"Task"="End Ramp 2", "begin time"=451.62219999999996, "end time"=451.6322, "Chops"=[FALSE, FALSE, FALSE, FALSE, FALSE, TRUE, TRUE, FALSE, FALSE, FALSE, FALSE, FALSE]}, {"Task"="End Ramp 2", "begin time"=484.9622, "end time"=484.9722, "Chops"=[FALSE, FALSE, FALSE, FALSE, FALSE, TRUE, TRUE, FALSE, FALSE, FALSE, FALSE, FALSE]}, {"Task"="Framegrabber Trigger", "begin time"=502.36721, "end time"=502.37721, "Chops"=[TRUE, TRUE, TRUE, TRUE, TRUE, TRUE, FALSE, FALSE, FALSE, FALSE, FALSE, FALSE]}, {"Task"="End Ramp 2", "begin time"=518.2922, "end time"=518.3022, "Chops"=[FALSE, FALSE, FALSE, FALSE, FALSE, TRUE, TRUE, FALSE, FALSE, FALSE, FALSE, FALSE]}, {"Task"="Kick to MCP", "begin time"=520.2922, "end time"=520.2972, "Chops"=[FALSE, FALSE, FALSE, FALSE, FALSE, FALSE, FALSE, FALSE, FALSE, FALSE, FALSE, FALSE]}, {"Task"="Scope trigger 2", "begin time"=520.2922, "end time"=520.3022, "Chops"=[TRUE, TRUE, TRUE, FALSE, FALSE, FALSE, FALSE, FALSE, FALSE, FALSE, FALSE, FALSE]}, {"Task"="Zero DAC", "begin time"=520.2972, "end time"=530.2972, "Chops"=[FALSE, FALSE, FALSE, FALSE, FALSE, FALSE, FALSE, FALSE, FALSE, FALSE, FALSE, FALSE]}, {"Task"="Trigger Scope", "begin time"=520.3072, "end time"=520.3172, "Chops"=[FALSE, FALSE, FALSE, FALSE, FALSE, FALSE, TRUE, FALSE, FALSE, FALSE, FALSE, FALSE]}, {"Task"="Img MCP Trigger", "begin time"=520.36721, "end time"=520.37721, "Chops"=[TRUE, TRUE, TRUE, TRUE, TRUE, TRUE, FALSE, FALSE, FALSE, FALSE, FALSE, FALSE]}] caption="DIO64 Debug" {"end time" format="%#_8g"; "begin time" format="%#_8g"}
  out "dio64:debug1":T8(array[cluster])=[{"Begin (ms)"=0.0, "Duration (ms)"=0.17220000000000013, "DIO64 Line 1"=[FALSE, FALSE, FALSE, FALSE, FALSE, FALSE, FALSE, FALSE, FALSE, FALSE, FALSE, FALSE, FALSE, FALSE, FALSE, FALSE], "DIO64 Line 2"=[FALSE, FALSE, FALSE, FALSE, FALSE, FALSE, FALSE, FALSE, FALSE, FALSE, FALSE, FALSE, FALSE, FALSE, FALSE, FALSE], "DIO64 Line 3"=[FALSE, FALSE, FALSE, FALSE, FALSE, FALSE, FALSE, FALSE, FALSE, FALSE, FALSE, FALSE, FALSE, FALSE, FALSE, FALSE], "DIO64 Line 4"=[FALSE, FALSE, FALSE, FALSE, FALSE, FALSE, FALSE, FALSE, FALSE, FALSE, FALSE, FALSE, FALSE, FALSE, FALSE, FALSE]}, {"Begin (ms)"=0.17220000000000013, "Duration (ms)"=18.0024, "DIO64 Line 1"=[FALSE, FALSE, FALSE, FALSE, FALSE, FALSE, FALSE, FALSE, FALSE, FALSE, FALSE, FALSE, FALSE, TRUE, FALSE, FALSE], "DIO64 Line 2"=[FALSE, FALSE, FALSE, FALSE, FALSE, FALSE, FALSE, FALSE, FALSE, FALSE, FALSE, FALSE, FALSE, FALSE, FALSE, TRUE], "DIO64 Line 3"=[FALSE, FALSE, FALSE, FALSE, FALSE, FALSE, FALSE, FALSE, FALSE, FALSE, FALSE, FALSE, FALSE, FALSE, FALSE, FALSE], "DIO64 Line 4"=[FALSE, FALSE, FALSE, FALSE, FALSE, FALSE, FALSE, FALSE, FALSE, FALSE, FALSE, FALSE, FALSE, FALSE, FALSE, FALSE]}, {"Begin (ms)"=18.1746, "Duration (ms)"=0.00999999999999801, "DIO64 Line 1"=[FALSE, FALSE, FALSE, FALSE, FALSE, FALSE, FALSE, FALSE, FALSE, FALSE, FALSE, FALSE, FALSE, TRUE, FALSE, FALSE], "DIO64 Line 2"=[FALSE, FALSE, FALSE, FALSE, FALSE, FALSE, FALSE, FALSE, FALSE, FALSE, FALSE, FALSE, FALSE, FALSE, FALSE, TRUE], "DIO64 Line 3"=[FALSE, FALSE, FALSE, FALSE, FALSE, FALSE, FALSE, FALSE, FALSE, FALSE, FALSE, FALSE, FALSE, FALSE, FALSE, FALSE], "DIO64 Line 4"=[TRUE, FALSE, FALSE, FALSE, FALSE, FALSE, FALSE, FALSE, FALSE, FALSE, FALSE, FALSE, FALSE, FALSE, FALSE, FALSE]}, {"Begin (ms)"=18.1846, "Duration (ms)"=0.9876000000000005, "DIO64 Line 1"=[FALSE, FALSE, FALSE, FALSE, FALSE, FALSE, FALSE, FALSE, FALSE, FALSE, FALSE, FALSE, FALSE, TRUE, FALSE, FALSE], "DIO64 Line 2"=[FALSE, FALSE, FALSE, FALSE, FALSE, FALSE, FALSE, FALSE, FALSE, FALSE, FALSE, FALSE, FALSE, FALSE, FALSE, TRUE], "DIO64 Line 3"=[FALSE, FALSE, FALSE, FALSE, FALSE, FALSE, FALSE, FALSE, FALSE, FALSE, FALSE, FALSE, FALSE, FALSE, FALSE, FALSE], "DIO64 Line 4"=[FALSE, FALSE, FALSE, FALSE, FALSE, FALSE, FALSE, FALSE, FALSE, FALSE, FALSE, FALSE, FALSE, FALSE, FALSE, FALSE]}, {"Begin (ms)"=19.1722, "Duration (ms)"=0.010000000000001563, "DIO64 Line 1"=[FALSE, FALSE, FALSE, FALSE, FALSE, FALSE, FALSE, FALSE, FALSE, FALSE, FALSE, FALSE, FALSE, TRUE, FALSE, FALSE], "DIO64 Line 2"=[FALSE, FALSE, FALSE, FALSE, FALSE, FALSE, FALSE, FALSE, FALSE, TRUE, FALSE, FALSE, FALSE, FALSE, FALSE, TRUE], "DIO64 Line 3"=[FALSE, TRUE, FALSE, FALSE, FALSE, FALSE, FALSE, FALSE, FALSE, FALSE, FALSE, FALSE, FALSE, FALSE, FALSE, FALSE], "DIO64 Line 4"=[FALSE, FALSE, FALSE, FALSE, FALSE, FALSE, FALSE, FALSE, FALSE, FALSE, FALSE, FALSE, FALSE, FALSE, FALSE, FALSE]}, {"Begin (ms)"=19.1822, "Duration (ms)"=0.10489999999999, "DIO64 Line 1"=[FALSE, FALSE, FALSE, FALSE, FALSE, FALSE, FALSE, FALSE, FALSE, FALSE, FALSE, FALSE, FALSE, TRUE, FALSE, FALSE], "DIO64 Line 2"=[FALSE, FALSE, FALSE, FALSE, FALSE, FALSE, FALSE, FALSE, FALSE, FALSE, FALSE, FALSE, FALSE, FALSE, FALSE, TRUE], "DIO64 Line 3"=[FALSE, FALSE, FALSE, FALSE, FALSE, FALSE, FALSE, FALSE, FALSE, FALSE, FALSE, FALSE, FALSE, FALSE, FALSE, FALSE], "DIO64 Line 4"=[FALSE, FALSE, FALSE, FALSE, FALSE, FALSE, FALSE, FALSE, FALSE, FALSE, FALSE, FALSE, FALSE, FALSE, FALSE, FALSE]}, {"Begin (ms)"=19.28709999999999, "Duration (ms)"=0.0010000000000012221, "DIO64 Line 1"=[FALSE, FALSE, FALSE, TRUE, FALSE, FALSE, FALSE, FALSE, FALSE, FALSE, FALSE, FALSE, FALSE, TRUE, FALSE, FALSE], "DIO64 Line 2"=[FALSE, FALSE, FALSE, FALSE, FALSE, FALSE, FALSE, FALSE, FALSE, FALSE, FALSE, FALSE, FALSE, FALSE, FALSE, TRUE], "DIO64 Line 3"=[FALSE, FALSE, FALSE, FALSE, FALSE, FALSE, FALSE, FALSE, FALSE, FALSE, FALSE, FALSE, FALSE, FALSE, FALSE, FALSE], "DIO64 Line 4"=[FALSE, FALSE, FALSE, FALSE, FALSE, FALSE, FALSE, FALSE, FALSE, FALSE, FALSE, FALSE, FALSE, FALSE, FALSE, FALSE]}, {"Begin (ms)"=19.288099999999993, "Duration (ms)"=0.009000000000000341, "DIO64 Line 1"=[FALSE, FALSE, FALSE, TRUE, FALSE, FALSE, FALSE, FALSE, FALSE, FALSE, FALSE, FALSE, FALSE, TRUE, TRUE, FALSE], "DIO64 Line 2"=[FALSE, FALSE, FALSE, FALSE, FALSE, FALSE, FALSE, FALSE, FALSE, FALSE, FALSE, FALSE, FALSE, FALSE, FALSE, TRUE], "DIO64 Line 3"=[FALSE, FALSE, FALSE, FALSE, FALSE, FALSE, FALSE, FALSE, FALSE, FALSE, FALSE, FALSE, FALSE, FALSE, FALSE, FALSE], "DIO64 Line 4"=[FALSE, FALSE, FALSE, FALSE, FALSE, FALSE, FALSE, FALSE, FALSE, FALSE, FALSE, FALSE, FALSE, FALSE, FALSE, FALSE]}, {"Begin (ms)"=19.297099999999993, "Duration (ms)"=0.036000000000001364, "DIO64 Line 1"=[FALSE, FALSE, FALSE, FALSE, FALSE, FALSE, FALSE, FALSE, FALSE, FALSE, FALSE, FALSE, FALSE, TRUE, TRUE, FALSE], "DIO64 Line 2"=[FALSE, FALSE, FALSE, FALSE, FALSE, FALSE, FALSE, FALSE, FALSE, FALSE, FALSE, FALSE, FALSE, FALSE, FALSE, TRUE], "DIO64 Line 3"=[FALSE, FALSE, FALSE, FALSE, FALSE, FALSE, FALSE, FALSE, FALSE, FALSE, FALSE, FALSE, FALSE, FALSE, FALSE, FALSE], "DIO64 Line 4"=[FALSE, FALSE, FALSE, FALSE, FALSE, FALSE, FALSE, FALSE, FALSE, FALSE, FALSE, FALSE, FALSE, FALSE, FALSE, FALSE]}, {"Begin (ms)"=19.333099999999995, "Duration (ms)"=0.07909999999999684, "DIO64 Line 1"=[FALSE, FALSE, FALSE, FALSE, FALSE, FALSE, FALSE, FALSE, FALSE, FALSE, FALSE, FALSE, FALSE, TRUE, FALSE, FALSE], "DIO64 Line 2"=[FALSE, FALSE, FALSE, FALSE, FALSE, FALSE, FALSE, FALSE, FALSE, FALSE, FALSE, FALSE, FALSE, FALSE, FALSE, TRUE], "DIO64 Line 3"=[FALSE, FALSE, FALSE, FALSE, FALSE, FALSE, FALSE, FALSE, FALSE, FALSE, FALSE, FALSE, FALSE, FALSE, FALSE, FALSE], "DIO64 Line 4"=[FALSE, FALSE, FALSE, FALSE, FALSE, FALSE, FALSE, FALSE, FALSE, FALSE, FALSE, FALSE, FALSE, FALSE, FALSE, FALSE]}, {"Begin (ms)"=19.41219999999999, "Duration (ms)"=0.010000000000001563, "DIO64 Line 1"=[FALSE, FALSE, FALSE, FALSE, TRUE, FALSE, FALSE, FALSE, FALSE, FALSE, FALSE, FALSE, FALSE, TRUE, FALSE, FALSE], "DIO64 Line 2"=[FALSE, FALSE, FALSE, FALSE, FALSE, FALSE, FALSE, FALSE, FALSE, FALSE, FALSE, FALSE, FALSE, FALSE, FALSE, TRUE], "DIO64 Line 3"=[FALSE, FALSE, FALSE, FALSE, FALSE, FALSE, FALSE, FALSE, FALSE, FALSE, FALSE, FALSE, FALSE, FALSE, FALSE, FALSE], "DIO64 Line 4"=[FALSE, FALSE, FALSE, FALSE, FALSE, FALSE, FALSE, FALSE, FALSE, FALSE, FALSE, FALSE, FALSE, FALSE, FALSE, FALSE]}, {"Begin (ms)"=19.422199999999993, "Duration (ms)"=0.7090000000000067, "DIO64 Line 1"=[FALSE, FALSE, FALSE, FALSE, FALSE, FALSE, FALSE, FALSE, FALSE, FALSE, FALSE, FALSE, FALSE, TRUE, FALSE, FALSE], "DIO64 Line 2"=[FALSE, FALSE, FALSE, FALSE, FALSE, FALSE, FALSE, FALSE, FALSE, FALSE, FALSE, FALSE, FALSE, FALSE, FALSE, TRUE], "DIO64 Line 3"=[FALSE, FALSE, FALSE, FALSE, FALSE, FALSE, FALSE, FALSE, FALSE, FALSE, FALSE, FALSE, FALSE, FALSE, FALSE, FALSE], "DIO64 Line 4"=[FALSE, FALSE, FALSE, FALSE, FALSE, FALSE, FALSE, FALSE, FALSE, FALSE, FALSE, FALSE, FALSE, FALSE, FALSE, FALSE]}, {"Begin (ms)"=20.1312, "Duration (ms)"=0.03999999999999915, "DIO64 Line 1"=[FALSE, FALSE, FALSE, FALSE, FALSE, FALSE, FALSE, FALSE, FALSE, TRUE, TRUE, FALSE, FALSE, TRUE, FALSE, FALSE], "DIO64 Line 2"=[FALSE, FALSE, FALSE, FALSE, FALSE, FALSE, FALSE, FALSE, FALSE, FALSE, FALSE, FALSE, FALSE, FALSE, FALSE, TRUE], "DIO64 Line 3"=[FALSE, FALSE, FALSE, FALSE, FALSE, FALSE, FALSE, FALSE, FALSE, FALSE, FALSE, FALSE, FALSE, FALSE, FALSE, FALSE], "DIO64 Line 4"=[FALSE, FALSE, FALSE, FALSE, FALSE, FALSE, FALSE, FALSE, FALSE, FALSE, FALSE, FALSE, FALSE, FALSE, FALSE, FALSE]}, {"Begin (ms)"=20.1712, "Duration (ms)"=0.0010000000000012221, "DIO64 Line 1"=[FALSE, FALSE, FALSE, FALSE, FALSE, FALSE, FALSE, FALSE, FALSE, TRUE, FALSE, FALSE, FALSE, TRUE, FALSE, FALSE], "DIO64 Line 2"=[FALSE, FALSE, FALSE, FALSE, FALSE, FALSE, FALSE, FALSE, FALSE, FALSE, FALSE, FALSE, FALSE, FALSE, FALSE, TRUE], "DIO64 Line 3"=[FALSE, FALSE, FALSE, FALSE, FALSE, FALSE, FALSE, FALSE, FALSE, FALSE, FALSE, FALSE, FALSE, FALSE, FALSE, FALSE], "DIO64 Line 4"=[FALSE, FALSE, FALSE, FALSE, FALSE, FALSE, FALSE, FALSE, FALSE, FALSE, FALSE, FALSE, FALSE, FALSE, FALSE, FALSE]}, {"Begin (ms)"=20.1722, "Duration (ms)"=11.0, "DIO64 Line 1"=[FALSE, FALSE, FALSE, FALSE, FALSE, FALSE, TRUE, FALSE, FALSE, FALSE, FALSE, FALSE, FALSE, TRUE, FALSE, FALSE], "DIO64 Line 2"=[FALSE, FALSE, FALSE, FALSE, TRUE, FALSE, FALSE, FALSE, FALSE, FALSE, FALSE, FALSE, FALSE, TRUE, FALSE, TRUE], "DIO64 Line 3"=[FALSE, FALSE, FALSE, TRUE, FALSE, FALSE, FALSE, FALSE, FALSE, FALSE, FALSE, FALSE, FALSE, FALSE, FALSE, FALSE], "DIO64 Line 4"=[FALSE, FALSE, FALSE, FALSE, FALSE, FALSE, FALSE, FALSE, FALSE, FALSE, FALSE, FALSE, FALSE, FALSE, FALSE, TRUE]}, {"Begin (ms)"=31.1722, "Duration (ms)"=1.0000000000000036, "DIO64 Line 1"=[FALSE, FALSE, FALSE, FALSE, FALSE, FALSE, TRUE, FALSE, FALSE, FALSE, FALSE, FALSE, FALSE, TRUE, FALSE, FALSE], "DIO64 Line 2"=[TRUE, FALSE, FALSE, FALSE, TRUE, FALSE, FALSE, FALSE, FALSE, FALSE, FALSE, FALSE, FALSE, TRUE, FALSE, TRUE], "DIO64 Line 3"=[FALSE, FALSE, FALSE, TRUE, FALSE, FALSE, FALSE, FALSE, FALSE, FALSE, FALSE, FALSE, FALSE, FALSE, FALSE, FALSE], "DIO64 Line 4"=[FALSE, FALSE, FALSE, FALSE, FALSE, FALSE, FALSE, FALSE, FALSE, FALSE, FALSE, FALSE, FALSE, FALSE, FALSE, TRUE]}, {"Begin (ms)"=32.172200000000004, "Duration (ms)"=68.0, "DIO64 Line 1"=[FALSE, FALSE, FALSE, FALSE, FALSE, FALSE, TRUE, FALSE, FALSE, FALSE, FALSE, TRUE, FALSE, TRUE, FALSE, FALSE], "DIO64 Line 2"=[TRUE, FALSE, FALSE, FALSE, TRUE, FALSE, FALSE, FALSE, FALSE, FALSE, FALSE, FALSE, FALSE, TRUE, TRUE, TRUE], "DIO64 Line 3"=[FALSE, FALSE, FALSE, TRUE, FALSE, FALSE, FALSE, FALSE, FALSE, FALSE, FALSE, FALSE, FALSE, FALSE, FALSE, FALSE], "DIO64 Line 4"=[FALSE, FALSE, FALSE, FALSE, FALSE, FALSE, FALSE, FALSE, FALSE, FALSE, FALSE, FALSE, FALSE, FALSE, FALSE, TRUE]}, {"Begin (ms)"=100.1722, "Duration (ms)"=12.0, "DIO64 Line 1"=[FALSE, FALSE, FALSE, FALSE, FALSE, FALSE, TRUE, FALSE, FALSE, FALSE, FALSE, TRUE, FALSE, FALSE, FALSE, FALSE], "DIO64 Line 2"=[TRUE, FALSE, FALSE, FALSE, TRUE, FALSE, FALSE, FALSE, FALSE, FALSE, FALSE, FALSE, FALSE, TRUE, TRUE, FALSE], "DIO64 Line 3"=[FALSE, FALSE, FALSE, TRUE, FALSE, FALSE, FALSE, FALSE, FALSE, FALSE, FALSE, FALSE, FALSE, FALSE, FALSE, FALSE], "DIO64 Line 4"=[FALSE, FALSE, FALSE, FALSE, FALSE, FALSE, FALSE, FALSE, FALSE, FALSE, FALSE, FALSE, FALSE, FALSE, FALSE, TRUE]}, {"Begin (ms)"=112.1722, "Duration (ms)"=0.010000000000005116, "DIO64 Line 1"=[FALSE, FALSE, FALSE, FALSE, FALSE, FALSE, TRUE, FALSE, FALSE, FALSE, FALSE, TRUE, FALSE, FALSE, FALSE, FALSE], "DIO64 Line 2"=[TRUE, FALSE, FALSE, FALSE, TRUE, FALSE, FALSE, FALSE, FALSE, FALSE, FALSE, FALSE, FALSE, TRUE, FALSE, FALSE], "DIO64 Line 3"=[FALSE, FALSE, FALSE, TRUE, FALSE, FALSE, FALSE, FALSE, FALSE, FALSE, FALSE, FALSE, FALSE, FALSE, FALSE, FALSE], "DIO64 Line 4"=[FALSE, FALSE, FALSE, FALSE, FALSE, FALSE, FALSE, FALSE, FALSE, FALSE, FALSE, FALSE, FALSE, FALSE, FALSE, TRUE]}, {"Begin (ms)"=112.18220000000001, "Duration (ms)"=4.989999999999995, "DIO64 Line 1"=[FALSE, FALSE, FALSE, FALSE, FALSE, FALSE, TRUE, FALSE, FALSE, FALSE, FALSE, TRUE, FALSE, FALSE, FALSE, FALSE], "DIO64 Line 2"=[TRUE, FALSE, FALSE, FALSE, TRUE, FALSE, FALSE, FALSE, FALSE, FALSE, FALSE, FALSE, FALSE, TRUE, FALSE, FALSE], "DIO64 Line 3"=[FALSE, FALSE, FALSE, TRUE, FALSE, FALSE, FALSE, FALSE, FALSE, FALSE, FALSE, FALSE, FALSE, FALSE, FALSE, FALSE], "DIO64 Line 4"=[FALSE, FALSE, FALSE, FALSE, FALSE, FALSE, FALSE, FALSE, FALSE, FALSE, FALSE, FALSE, FALSE, FALSE, FALSE, TRUE]}, {"Begin (ms)"=117.1722, "Duration (ms)"=3.0, "DIO64 Line 1"=[FALSE, FALSE, FALSE, FALSE, FALSE, FALSE, TRUE, FALSE, FALSE, FALSE, FALSE, FALSE, FALSE, FALSE, FALSE, FALSE], "DIO64 Line 2"=[TRUE, FALSE, FALSE, FALSE, TRUE, FALSE, FALSE, FALSE, FALSE, FALSE, FALSE, FALSE, FALSE, TRUE, FALSE, FALSE], "DIO64 Line 3"=[FALSE, FALSE, FALSE, TRUE, FALSE, FALSE, FALSE, FALSE, FALSE, FALSE, FALSE, FALSE, FALSE, FALSE, FALSE, FALSE], "DIO64 Line 4"=[FALSE, FALSE, FALSE, FALSE, FALSE, FALSE, FALSE, FALSE, FALSE, FALSE, FALSE, FALSE, FALSE, FALSE, FALSE, TRUE]}, {"Begin (ms)"=120.1722, "Duration (ms)"=10.0, "DIO64 Line 1"=[FALSE, FALSE, FALSE, FALSE, FALSE, FALSE, TRUE, FALSE, FALSE, FALSE, FALSE, FALSE, FALSE, FALSE, FALSE, FALSE], "DIO64 Line 2"=[TRUE, FALSE, FALSE, TRUE, TRUE, FALSE, FALSE, FALSE, FALSE, FALSE, FALSE, FALSE, FALSE, TRUE, FALSE, FALSE], "DIO64 Line 3"=[FALSE, FALSE, FALSE, TRUE, FALSE, FALSE, FALSE, FALSE, FALSE, FALSE, FALSE, FALSE, FALSE, FALSE, FALSE, FALSE], "DIO64 Line 4"=[FALSE, FALSE, FALSE, FALSE, FALSE, FALSE, FALSE, FALSE, FALSE, FALSE, FALSE, FALSE, FALSE, FALSE, FALSE, TRUE]}, {"Begin (ms)"=130.1722, "Duration (ms)"=0.009999999999990905, "DIO64 Line 1"=[FALSE, FALSE, FALSE, FALSE, FALSE, FALSE, TRUE, FALSE, FALSE, FALSE, FALSE, FALSE, FALSE, FALSE, FALSE, FALSE], "DIO64 Line 2"=[TRUE, FALSE, FALSE, TRUE, TRUE, FALSE, FALSE, FALSE, TRUE, FALSE, FALSE, TRUE, FALSE, TRUE, FALSE, FALSE], "DIO64 Line 3"=[FALSE, FALSE, FALSE, TRUE, FALSE, FALSE, FALSE, FALSE, FALSE, FALSE, FALSE, FALSE, FALSE, FALSE, FALSE, FALSE], "DIO64 Line 4"=[FALSE, FALSE, FALSE, FALSE, FALSE, FALSE, FALSE, FALSE, FALSE, FALSE, FALSE, FALSE, FALSE, FALSE, FALSE, TRUE]}, {"Begin (ms)"=130.1822, "Duration (ms)"=2.990000000000009, "DIO64 Line 1"=[FALSE, FALSE, FALSE, FALSE, FALSE, FALSE, TRUE, FALSE, FALSE, FALSE, FALSE, FALSE, FALSE, FALSE, FALSE, FALSE], "DIO64 Line 2"=[TRUE, FALSE, FALSE, TRUE, TRUE, FALSE, FALSE, FALSE, TRUE, FALSE, FALSE, FALSE, FALSE, TRUE, FALSE, FALSE], "DIO64 Line 3"=[FALSE, FALSE, FALSE, TRUE, FALSE, FALSE, FALSE, FALSE, FALSE, FALSE, FALSE, FALSE, FALSE, FALSE, FALSE, FALSE], "DIO64 Line 4"=[FALSE, FALSE, FALSE, FALSE, FALSE, FALSE, FALSE, FALSE, FALSE, FALSE, FALSE, FALSE, FALSE, FALSE, FALSE, TRUE]}, {"Begin (ms)"=133.1722, "Duration (ms)"=5.0, "DIO64 Line 1"=[FALSE, FALSE, FALSE, FALSE, FALSE, FALSE, TRUE, FALSE, FALSE, FALSE, FALSE, FALSE, FALSE, FALSE, FALSE, FALSE], "DIO64 Line 2"=[TRUE, FALSE, FALSE, TRUE, TRUE, FALSE, FALSE, FALSE, FALSE, FALSE, FALSE, FALSE, FALSE, TRUE, FALSE, FALSE], "DIO64 Line 3"=[FALSE, FALSE, FALSE, TRUE, FALSE, FALSE, FALSE, FALSE, FALSE, FALSE, FALSE, FALSE, FALSE, FALSE, FALSE, FALSE], "DIO64 Line 4"=[FALSE, FALSE, FALSE, FALSE, FALSE, FALSE, FALSE, FALSE, FALSE, FALSE, FALSE, FALSE, FALSE, FALSE, FALSE, TRUE]}, {"Begin (ms)"=138.1722, "Duration (ms)"=0.9499999999999886, "DIO64 Line 1"=[FALSE, FALSE, FALSE, FALSE, FALSE, FALSE, TRUE, FALSE, FALSE, FALSE, FALSE, FALSE, FALSE, FALSE, FALSE, FALSE], "DIO64 Line 2"=[TRUE, FALSE, FALSE, TRUE, TRUE, FALSE, FALSE, FALSE, FALSE, FALSE, FALSE, FALSE, TRUE, TRUE, FALSE, FALSE], "DIO64 Line 3"=[FALSE, FALSE, FALSE, TRUE, FALSE, FALSE, FALSE, FALSE, FALSE, FALSE, FALSE, FALSE, FALSE, FALSE, FALSE, FALSE], "DIO64 Line 4"=[FALSE, FALSE, FALSE, FALSE, FALSE, FALSE, FALSE, FALSE, FALSE, FALSE, FALSE, FALSE, FALSE, FALSE, FALSE, TRUE]}, {"Begin (ms)"=139.1222, "Duration (ms)"=255.99999999999997, "DIO64 Line 1"=[FALSE, FALSE, FALSE, FALSE, FALSE, FALSE, TRUE, FALSE, FALSE, FALSE, FALSE, FALSE, FALSE, FALSE, FALSE, FALSE], "DIO64 Line 2"=[TRUE, FALSE, FALSE, TRUE, TRUE, FALSE, FALSE, FALSE, FALSE, FALSE, FALSE, FALSE, FALSE, TRUE, FALSE, FALSE], "DIO64 Line 3"=[FALSE, FALSE, FALSE, TRUE, FALSE, FALSE, FALSE, FALSE, FALSE, FALSE, FALSE, FALSE, FALSE, FALSE, FALSE, FALSE], "DIO64 Line 4"=[FALSE, FALSE, FALSE, FALSE, FALSE, FALSE, FALSE, FALSE, FALSE, FALSE, FALSE, FALSE, FALSE, FALSE, FALSE, TRUE]}, {"Begin (ms)"=395.12219999999996, "Duration (ms)"=0.9499999999999886, "DIO64 Line 1"=[FALSE, FALSE, FALSE, FALSE, FALSE, FALSE, TRUE, FALSE, FALSE, FALSE, FALSE, FALSE, FALSE, FALSE, FALSE, FALSE], "DIO64 Line 2"=[TRUE, FALSE, FALSE, TRUE, TRUE, FALSE, FALSE, FALSE, FALSE, FALSE, FALSE, FALSE, TRUE, TRUE, FALSE, FALSE], "DIO64 Line 3"=[FALSE, FALSE, FALSE, TRUE, FALSE, FALSE, FALSE, FALSE, FALSE, FALSE, FALSE, FALSE, FALSE, FALSE, FALSE, FALSE], "DIO64 Line 4"=[FALSE, FALSE, FALSE, FALSE, FALSE, FALSE, FALSE, FALSE, FALSE, FALSE, FALSE, FALSE, FALSE, FALSE, FALSE, TRUE]}, {"Begin (ms)"=396.07219999999995, "Duration (ms)"=2.2200000000000273, "DIO64 Line 1"=[FALSE, FALSE, FALSE, FALSE, FALSE, FALSE, TRUE, FALSE, FALSE, FALSE, FALSE, FALSE, FALSE, FALSE, FALSE, FALSE], "DIO64 Line 2"=[TRUE, FALSE, FALSE, TRUE, TRUE, FALSE, FALSE, FALSE, FALSE, FALSE, FALSE, FALSE, FALSE, TRUE, FALSE, FALSE], "DIO64 Line 3"=[FALSE, FALSE, FALSE, TRUE, FALSE, FALSE, FALSE, FALSE, FALSE, FALSE, FALSE, FALSE, FALSE, FALSE, FALSE, FALSE], "DIO64 Line 4"=[FALSE, FALSE, FALSE, FALSE, FALSE, FALSE, FALSE, FALSE, FALSE, FALSE, FALSE, FALSE, FALSE, FALSE, FALSE, TRUE]}, {"Begin (ms)"=398.2922, "Duration (ms)"=3.7799999999999727, "DIO64 Line 1"=[FALSE, FALSE, FALSE, FALSE, FALSE, FALSE, TRUE, FALSE, FALSE, FALSE, FALSE, FALSE, FALSE, FALSE, FALSE, FALSE], "DIO64 Line 2"=[TRUE, TRUE, FALSE, TRUE, TRUE, TRUE, FALSE, FALSE, FALSE, FALSE, FALSE, FALSE, FALSE, TRUE, FALSE, FALSE], "DIO64 Line 3"=[FALSE, FALSE, FALSE, TRUE, FALSE, FALSE, FALSE, FALSE, FALSE, FALSE, FALSE, FALSE, FALSE, FALSE, FALSE, FALSE], "DIO64 Line 4"=[FALSE, FALSE, FALSE, FALSE, FALSE, FALSE, FALSE, FALSE, FALSE, FALSE, FALSE, FALSE, FALSE, FALSE, FALSE, TRUE]}, {"Begin (ms)"=402.07219999999995, "Duration (ms)"=0.0020000000000095497, "DIO64 Line 1"=[FALSE, FALSE, FALSE, FALSE, FALSE, FALSE, TRUE, FALSE, FALSE, FALSE, FALSE, FALSE, FALSE, FALSE, FALSE, FALSE], "DIO64 Line 2"=[TRUE, TRUE, FALSE, TRUE, TRUE, TRUE, FALSE, FALSE, TRUE, FALSE, FALSE, FALSE, FALSE, TRUE, FALSE, FALSE], "DIO64 Line 3"=[FALSE, FALSE, FALSE, TRUE, FALSE, FALSE, FALSE, FALSE, FALSE, FALSE, FALSE, FALSE, FALSE, FALSE, FALSE, FALSE], "DIO64 Line 4"=[FALSE, FALSE, FALSE, FALSE, FALSE, FALSE, FALSE, FALSE, FALSE, FALSE, FALSE, FALSE, FALSE, FALSE, FALSE, TRUE]}, {"Begin (ms)"=402.07419999999996, "Duration (ms)"=2.9979999999999905, "DIO64 Line 1"=[FALSE, FALSE, FALSE, FALSE, FALSE, FALSE, TRUE, FALSE, FALSE, FALSE, FALSE, FALSE, FALSE, FALSE, FALSE, FALSE], "DIO64 Line 2"=[TRUE, TRUE, FALSE, TRUE, TRUE, TRUE, FALSE, FALSE, TRUE, FALSE, FALSE, FALSE, FALSE, TRUE, FALSE, FALSE], "DIO64 Line 3"=[FALSE, FALSE, FALSE, TRUE, FALSE, FALSE, FALSE, FALSE, FALSE, FALSE, FALSE, FALSE, FALSE, FALSE, FALSE, FALSE], "DIO64 Line 4"=[FALSE, FALSE, FALSE, FALSE, FALSE, FALSE, FALSE, FALSE, FALSE, FALSE, FALSE, FALSE, FALSE, FALSE, FALSE, TRUE]}, {"Begin (ms)"=405.07219999999995, "Duration (ms)"=0.0020000000000095497, "DIO64 Line 1"=[FALSE, FALSE, FALSE, FALSE, FALSE, FALSE, TRUE, FALSE, FALSE, FALSE, FALSE, FALSE, FALSE, FALSE, FALSE, FALSE], "DIO64 Line 2"=[TRUE, TRUE, FALSE, TRUE, TRUE, TRUE, FALSE, FALSE, FALSE, FALSE, FALSE, FALSE, FALSE, TRUE, FALSE, FALSE], "DIO64 Line 3"=[FALSE, FALSE, FALSE, TRUE, FALSE, FALSE, FALSE, FALSE, FALSE, FALSE, FALSE, FALSE, FALSE, FALSE, FALSE, FALSE], "DIO64 Line 4"=[FALSE, FALSE, FALSE, FALSE, FALSE, FALSE, FALSE, FALSE, FALSE, FALSE, FALSE, FALSE, FALSE, FALSE, FALSE, TRUE]}, {"Begin (ms)"=405.07419999999996, "Duration (ms)"=6.218000000000018, "DIO64 Line 1"=[FALSE, FALSE, FALSE, FALSE, FALSE, FALSE, TRUE, FALSE, FALSE, FALSE, FALSE, FALSE, FALSE, FALSE, FALSE, FALSE], "DIO64 Line 2"=[TRUE, TRUE, FALSE, TRUE, TRUE, TRUE, FALSE, FALSE, FALSE, FALSE, FALSE, FALSE, FALSE, TRUE, FALSE, FALSE], "DIO64 Line 3"=[FALSE, FALSE, FALSE, TRUE, FALSE, FALSE, FALSE, FALSE, FALSE, FALSE, FALSE, FALSE, FALSE, FALSE, FALSE, FALSE], "DIO64 Line 4"=[FALSE, FALSE, FALSE, FALSE, FALSE, FALSE, FALSE, FALSE, FALSE, FALSE, FALSE, FALSE, FALSE, FALSE, FALSE, TRUE]}, {"Begin (ms)"=411.2922, "Duration (ms)"=1.0, "DIO64 Line 1"=[FALSE, FALSE, FALSE, FALSE, FALSE, FALSE, TRUE, FALSE, FALSE, FALSE, FALSE, FALSE, FALSE, FALSE, FALSE, FALSE], "DIO64 Line 2"=[FALSE, TRUE, FALSE, TRUE, TRUE, TRUE, FALSE, FALSE, FALSE, FALSE, FALSE, FALSE, FALSE, TRUE, FALSE, FALSE], "DIO64 Line 3"=[FALSE, FALSE, FALSE, TRUE, FALSE, FALSE, FALSE, FALSE, FALSE, FALSE, FALSE, FALSE, FALSE, FALSE, FALSE, FALSE], "DIO64 Line 4"=[FALSE, FALSE, FALSE, FALSE, FALSE, FALSE, FALSE, FALSE, FALSE, FALSE, FALSE, FALSE, FALSE, FALSE, FALSE, TRUE]}, {"Begin (ms)"=412.2922, "Duration (ms)"=0.009999999999990905, "DIO64 Line 1"=[FALSE, FALSE, FALSE, FALSE, FALSE, FALSE, TRUE, FALSE, FALSE, FALSE, FALSE, FALSE, FALSE, FALSE, FALSE, FALSE], "DIO64 Line 2"=[FALSE, TRUE, FALSE, TRUE, TRUE, TRUE, FALSE, FALSE, FALSE, FALSE, FALSE, FALSE, FALSE, TRUE, FALSE, FALSE], "DIO64 Line 3"=[TRUE, FALSE, FALSE, TRUE, FALSE, FALSE, FALSE, FALSE, FALSE, FALSE, FALSE, FALSE, FALSE, FALSE, FALSE, FALSE], "DIO64 Line 4"=[FALSE, FALSE, FALSE, FALSE, FALSE, FALSE, FALSE, FALSE, FALSE, FALSE, FALSE, FALSE, FALSE, FALSE, FALSE, TRUE]}, {"Begin (ms)"=412.30219999999997, "Duration (ms)"=5.990000000000009, "DIO64 Line 1"=[FALSE, FALSE, FALSE, FALSE, FALSE, FALSE, TRUE, FALSE, FALSE, FALSE, FALSE, FALSE, FALSE, FALSE, FALSE, FALSE], "DIO64 Line 2"=[FALSE, TRUE, FALSE, TRUE, TRUE, TRUE, FALSE, FALSE, FALSE, FALSE, FALSE, FALSE, FALSE, TRUE, FALSE, FALSE], "DIO64 Line 3"=[FALSE, FALSE, FALSE, TRUE, FALSE, FALSE, FALSE, FALSE, FALSE, FALSE, FALSE, FALSE, FALSE, FALSE, FALSE, FALSE], "DIO64 Line 4"=[FALSE, FALSE, FALSE, FALSE, FALSE, FALSE, FALSE, FALSE, FALSE, FALSE, FALSE, FALSE, FALSE, FALSE, FALSE, TRUE]}, {"Begin (ms)"=418.2922, "Duration (ms)"=0.009999999999990905, "DIO64 Line 1"=[FALSE, FALSE, FALSE, FALSE, FALSE, FALSE, TRUE, FALSE, FALSE, FALSE, FALSE, FALSE, TRUE, FALSE, FALSE, FALSE], "DIO64 Line 2"=[FALSE, TRUE, FALSE, TRUE, TRUE, TRUE, FALSE, FALSE, FALSE, FALSE, FALSE, FALSE, FALSE, TRUE, FALSE, FALSE], "DIO64 Line 3"=[FALSE, FALSE, FALSE, TRUE, FALSE, FALSE, FALSE, FALSE, FALSE, FALSE, FALSE, FALSE, FALSE, FALSE, FALSE, FALSE], "DIO64 Line 4"=[FALSE, FALSE, FALSE, FALSE, FALSE, FALSE, FALSE, FALSE, FALSE, FALSE, FALSE, FALSE, FALSE, FALSE, FALSE, TRUE]}, {"Begin (ms)"=418.30219999999997, "Duration (ms)"=33.31999999999999, "DIO64 Line 1"=[FALSE, FALSE, FALSE, FALSE, FALSE, FALSE, TRUE, FALSE, FALSE, FALSE, FALSE, FALSE, FALSE, FALSE, FALSE, FALSE], "DIO64 Line 2"=[FALSE, TRUE, FALSE, TRUE, TRUE, TRUE, FALSE, FALSE, FALSE, FALSE, FALSE, FALSE, FALSE, TRUE, FALSE, FALSE], "DIO64 Line 3"=[FALSE, FALSE, FALSE, TRUE, FALSE, FALSE, FALSE, FALSE, FALSE, FALSE, FALSE, FALSE, FALSE, FALSE, FALSE, FALSE], "DIO64 Line 4"=[FALSE, FALSE, FALSE, FALSE, FALSE, FALSE, FALSE, FALSE, FALSE, FALSE, FALSE, FALSE, FALSE, FALSE, FALSE, TRUE]}, {"Begin (ms)"=451.62219999999996, "Duration (ms)"=0.010000000000047748, "DIO64 Line 1"=[FALSE, FALSE, FALSE, FALSE, FALSE, FALSE, TRUE, FALSE, FALSE, FALSE, FALSE, FALSE, TRUE, FALSE, FALSE, FALSE], "DIO64 Line 2"=[FALSE, TRUE, FALSE, TRUE, TRUE, TRUE, FALSE, FALSE, FALSE, FALSE, FALSE, FALSE, FALSE, TRUE, FALSE, FALSE], "DIO64 Line 3"=[FALSE, FALSE, FALSE, TRUE, FALSE, FALSE, FALSE, FALSE, FALSE, FALSE, FALSE, FALSE, FALSE, FALSE, FALSE, FALSE], "DIO64 Line 4"=[FALSE, FALSE, FALSE, FALSE, FALSE, FALSE, FALSE, FALSE, FALSE, FALSE, FALSE, FALSE, FALSE, FALSE, FALSE, TRUE]}, {"Begin (ms)"=451.6322, "Duration (ms)"=33.329999999999984, "DIO64 Line 1"=[FALSE, FALSE, FALSE, FALSE, FALSE, FALSE, TRUE, FALSE, FALSE, FALSE, FALSE, FALSE, FALSE, FALSE, FALSE, FALSE], "DIO64 Line 2"=[FALSE, TRUE, FALSE, TRUE, TRUE, TRUE, FALSE, FALSE, FALSE, FALSE, FALSE, FALSE, FALSE, TRUE, FALSE, FALSE], "DIO64 Line 3"=[FALSE, FALSE, FALSE, TRUE, FALSE, FALSE, FALSE, FALSE, FALSE, FALSE, FALSE, FALSE, FALSE, FALSE, FALSE, FALSE], "DIO64 Line 4"=[FALSE, FALSE, FALSE, FALSE, FALSE, FALSE, FALSE, FALSE, FALSE, FALSE, FALSE, FALSE, FALSE, FALSE, FALSE, TRUE]}, {"Begin (ms)"=484.9622, "Duration (ms)"=0.009999999999990905, "DIO64 Line 1"=[FALSE, FALSE, FALSE, FALSE, FALSE, FALSE, TRUE, FALSE, FALSE, FALSE, FALSE, FALSE, TRUE, FALSE, FALSE, FALSE], "DIO64 Line 2"=[FALSE, TRUE, FALSE, TRUE, TRUE, TRUE, FALSE, FALSE, FALSE, FALSE, FALSE, FALSE, FALSE, TRUE, FALSE, FALSE], "DIO64 Line 3"=[FALSE, FALSE, FALSE, TRUE, FALSE, FALSE, FALSE, FALSE, FALSE, FALSE, FALSE, FALSE, FALSE, FALSE, FALSE, FALSE], "DIO64 Line 4"=[FALSE, FALSE, FALSE, FALSE, FALSE, FALSE, FALSE, FALSE, FALSE, FALSE, FALSE, FALSE, FALSE, FALSE, FALSE, TRUE]}, {"Begin (ms)"=484.9722, "Duration (ms)"=17.395010000000013, "DIO64 Line 1"=[FALSE, FALSE, FALSE, FALSE, FALSE, FALSE, TRUE, FALSE, FALSE, FALSE, FALSE, FALSE, FALSE, FALSE, FALSE, FALSE], "DIO64 Line 2"=[FALSE, TRUE, FALSE, TRUE, TRUE, TRUE, FALSE, FALSE, FALSE, FALSE, FALSE, FALSE, FALSE, TRUE, FALSE, FALSE], "DIO64 Line 3"=[FALSE, FALSE, FALSE, TRUE, FALSE, FALSE, FALSE, FALSE, FALSE, FALSE, FALSE, FALSE, FALSE, FALSE, FALSE, FALSE], "DIO64 Line 4"=[FALSE, FALSE, FALSE, FALSE, FALSE, FALSE, FALSE, FALSE, FALSE, FALSE, FALSE, FALSE, FALSE, FALSE, FALSE, TRUE]}, {"Begin (ms)"=502.36721, "Duration (ms)"=0.009999999999990905, "DIO64 Line 1"=[FALSE, FALSE, FALSE, FALSE, FALSE, FALSE, TRUE, FALSE, FALSE, FALSE, FALSE, FALSE, FALSE, FALSE, FALSE, FALSE], "DIO64 Line 2"=[FALSE, TRUE, FALSE, TRUE, TRUE, TRUE, FALSE, FALSE, FALSE, FALSE, FALSE, FALSE, FALSE, TRUE, FALSE, FALSE], "DIO64 Line 3"=[FALSE, FALSE, FALSE, TRUE, FALSE, FALSE, FALSE, FALSE, FALSE, FALSE, FALSE, FALSE, FALSE, FALSE, FALSE, FALSE], "DIO64 Line 4"=[FALSE, FALSE, FALSE, FALSE, FALSE, FALSE, FALSE, FALSE, FALSE, FALSE, FALSE, FALSE, FALSE, FALSE, FALSE, TRUE]}, {"Begin (ms)"=502.37721, "Duration (ms)"=2.6949899999999616, "DIO64 Line 1"=[FALSE, FALSE, FALSE, FALSE, FALSE, FALSE, TRUE, FALSE, FALSE, FALSE, FALSE, FALSE, FALSE, FALSE, FALSE, FALSE], "DIO64 Line 2"=[FALSE, TRUE, FALSE, TRUE, TRUE, TRUE, FALSE, FALSE, FALSE, FALSE, FALSE, FALSE, FALSE, TRUE, FALSE, FALSE], "DIO64 Line 3"=[FALSE, FALSE, FALSE, TRUE, FALSE, FALSE, FALSE, FALSE, FALSE, FALSE, FALSE, FALSE, FALSE, FALSE, FALSE, FALSE], "DIO64 Line 4"=[FALSE, FALSE, FALSE, FALSE, FALSE, FALSE, FALSE, FALSE, FALSE, FALSE, FALSE, FALSE, FALSE, FALSE, FALSE, TRUE]}, {"Begin (ms)"=505.07219999999995, "Duration (ms)"=13.220000000000027, "DIO64 Line 1"=[FALSE, FALSE, FALSE, FALSE, FALSE, FALSE, TRUE, FALSE, FALSE, FALSE, FALSE, FALSE, FALSE, FALSE, FALSE, FALSE], "DIO64 Line 2"=[FALSE, TRUE, FALSE, FALSE, TRUE, TRUE, FALSE, FALSE, FALSE, FALSE, FALSE, FALSE, FALSE, TRUE, FALSE, FALSE], "DIO64 Line 3"=[FALSE, FALSE, FALSE, TRUE, FALSE, FALSE, FALSE, FALSE, FALSE, FALSE, FALSE, FALSE, FALSE, FALSE, FALSE, FALSE], "DIO64 Line 4"=[FALSE, FALSE, FALSE, FALSE, FALSE, FALSE, FALSE, FALSE, FALSE, FALSE, FALSE, FALSE, FALSE, FALSE, FALSE, TRUE]}, {"Begin (ms)"=518.2922, "Duration (ms)"=0.009999999999990905, "DIO64 Line 1"=[FALSE, FALSE, FALSE, FALSE, FALSE, FALSE, TRUE, FALSE, FALSE, FALSE, FALSE, FALSE, TRUE, FALSE, FALSE, FALSE], "DIO64 Line 2"=[FALSE, TRUE, FALSE, FALSE, TRUE, TRUE, FALSE, FALSE, FALSE, FALSE, FALSE, FALSE, FALSE, TRUE, FALSE, FALSE], "DIO64 Line 3"=[FALSE, FALSE, FALSE, TRUE, FALSE, FALSE, FALSE, FALSE, FALSE, FALSE, FALSE, FALSE, FALSE, FALSE, FALSE, FALSE], "DIO64 Line 4"=[FALSE, FALSE, FALSE, FALSE, FALSE, FALSE, FALSE, FALSE, FALSE, FALSE, FALSE, FALSE, FALSE, FALSE, FALSE, TRUE]}, {"Begin (ms)"=518.3022, "Duration (ms)"=1.990000000000009, "DIO64 Line 1"=[FALSE, FALSE, FALSE, FALSE, FALSE, FALSE, TRUE, FALSE, FALSE, FALSE, FALSE, FALSE, FALSE, FALSE, FALSE, FALSE], "DIO64 Line 2"=[FALSE, TRUE, FALSE, FALSE, TRUE, TRUE, FALSE, FALSE, FALSE, FALSE, FALSE, FALSE, FALSE, TRUE, FALSE, FALSE], "DIO64 Line 3"=[FALSE, FALSE, FALSE, TRUE, FALSE, FALSE, FALSE, FALSE, FALSE, FALSE, FALSE, FALSE, FALSE, FALSE, FALSE, FALSE], "DIO64 Line 4"=[FALSE, FALSE, FALSE, FALSE, FALSE, FALSE, FALSE, FALSE, FALSE, FALSE, FALSE, FALSE, FALSE, FALSE, FALSE, TRUE]}, {"Begin (ms)"=520.2922, "Duration (ms)"=0.0049999999999954525, "DIO64 Line 1"=[FALSE, FALSE, FALSE, FALSE, FALSE, FALSE, FALSE, FALSE, FALSE, TRUE, FALSE, FALSE, FALSE, FALSE, FALSE, FALSE], "DIO64 Line 2"=[FALSE, TRUE, FALSE, FALSE, FALSE, TRUE, FALSE, FALSE, FALSE, FALSE, FALSE, FALSE, FALSE, FALSE, FALSE, FALSE], "DIO64 Line 3"=[FALSE, FALSE, FALSE, FALSE, FALSE, FALSE, FALSE, FALSE, FALSE, FALSE, FALSE, FALSE, FALSE, FALSE, FALSE, FALSE], "DIO64 Line 4"=[FALSE, FALSE, FALSE, FALSE, FALSE, FALSE, FALSE, FALSE, FALSE, FALSE, FALSE, FALSE, FALSE, FALSE, FALSE, FALSE]}, {"Begin (ms)"=520.2972, "Duration (ms)"=0.0049999999999954525, "DIO64 Line 1"=[FALSE, FALSE, FALSE, FALSE, FALSE, FALSE, FALSE, FALSE, FALSE, TRUE, TRUE, FALSE, FALSE, FALSE, FALSE, FALSE], "DIO64 Line 2"=[FALSE, TRUE, FALSE, FALSE, FALSE, TRUE, FALSE, FALSE, FALSE, FALSE, FALSE, FALSE, FALSE, FALSE, FALSE, FALSE], "DIO64 Line 3"=[FALSE, FALSE, FALSE, FALSE, FALSE, FALSE, FALSE, FALSE, FALSE, FALSE, FALSE, FALSE, FALSE, FALSE, FALSE, FALSE], "DIO64 Line 4"=[FALSE, FALSE, FALSE, FALSE, FALSE, FALSE, FALSE, FALSE, FALSE, FALSE, FALSE, FALSE, FALSE, FALSE, FALSE, FALSE]}, {"Begin (ms)"=520.3022, "Duration (ms)"=0.0049999999999954525, "DIO64 Line 1"=[FALSE, FALSE, FALSE, FALSE, FALSE, FALSE, FALSE, FALSE, FALSE, TRUE, TRUE, FALSE, FALSE, FALSE, FALSE, FALSE], "DIO64 Line 2"=[FALSE, TRUE, FALSE, FALSE, FALSE, TRUE, FALSE, FALSE, FALSE, FALSE, FALSE, FALSE, FALSE, FALSE, FALSE, FALSE], "DIO64 Line 3"=[FALSE, FALSE, FALSE, FALSE, FALSE, FALSE, FALSE, FALSE, FALSE, FALSE, FALSE, FALSE, FALSE, FALSE, FALSE, FALSE], "DIO64 Line 4"=[FALSE, FALSE, FALSE, FALSE, FALSE, FALSE, FALSE, FALSE, FALSE, FALSE, FALSE, FALSE, FALSE, FALSE, FALSE, FALSE]}, {"Begin (ms)"=520.3072, "Duration (ms)"=0.009999999999990905, "DIO64 Line 1"=[FALSE, FALSE, FALSE, FALSE, FALSE, FALSE, FALSE, TRUE, FALSE, TRUE, TRUE, FALSE, FALSE, FALSE, FALSE, FALSE], "DIO64 Line 2"=[FALSE, TRUE, FALSE, FALSE, FALSE, TRUE, FALSE, FALSE, FALSE, FALSE, FALSE, FALSE, FALSE, FALSE, FALSE, FALSE], "DIO64 Line 3"=[FALSE, FALSE, FALSE, FALSE, FALSE, FALSE, FALSE, FALSE, FALSE, FALSE, FALSE, FALSE, FALSE, FALSE, FALSE, FALSE], "DIO64 Line 4"=[FALSE, TRUE, FALSE, FALSE, FALSE, FALSE, FALSE, FALSE, FALSE, FALSE, FALSE, FALSE, FALSE, FALSE, FALSE, FALSE]}, {"Begin (ms)"=520.3172, "Duration (ms)"=0.050010000000042965, "DIO64 Line 1"=[FALSE, FALSE, FALSE, FALSE, FALSE, FALSE, FALSE, FALSE, FALSE, TRUE, TRUE, FALSE, FALSE, FALSE, FALSE, FALSE], "DIO64 Line 2"=[FALSE, TRUE, FALSE, FALSE, FALSE, TRUE, FALSE, FALSE, FALSE, FALSE, FALSE, FALSE, FALSE, FALSE, FALSE, FALSE], "DIO64 Line 3"=[FALSE, FALSE, FALSE, FALSE, FALSE, FALSE, FALSE, FALSE, FALSE, FALSE, FALSE, FALSE, FALSE, FALSE, FALSE, FALSE], "DIO64 Line 4"=[FALSE, FALSE, FALSE, FALSE, FALSE, FALSE, FALSE, FALSE, FALSE, FALSE, FALSE, FALSE, FALSE, FALSE, FALSE, FALSE]}, {"Begin (ms)"=520.36721, "Duration (ms)"=0.009999999999990905, "DIO64 Line 1"=[FALSE, FALSE, FALSE, FALSE, FALSE, FALSE, FALSE, FALSE, FALSE, TRUE, TRUE, FALSE, FALSE, FALSE, FALSE, FALSE], "DIO64 Line 2"=[FALSE, TRUE, FALSE, FALSE, FALSE, TRUE, FALSE, FALSE, FALSE, FALSE, FALSE, FALSE, FALSE, FALSE, FALSE, FALSE], "DIO64 Line 3"=[FALSE, FALSE, FALSE, FALSE, FALSE, FALSE, FALSE, FALSE, FALSE, FALSE, FALSE, FALSE, FALSE, FALSE, FALSE, FALSE], "DIO64 Line 4"=[FALSE, FALSE, FALSE, FALSE, FALSE, FALSE, FALSE, FALSE, FALSE, FALSE, FALSE, FALSE, FALSE, FALSE, FALSE, FALSE]}, {"Begin (ms)"=520.37721, "Duration (ms)"=0.9149899999999889, "DIO64 Line 1"=[FALSE, FALSE, FALSE, FALSE, FALSE, FALSE, FALSE, FALSE, FALSE, TRUE, TRUE, FALSE, FALSE, FALSE, FALSE, FALSE], "DIO64 Line 2"=[FALSE, TRUE, FALSE, FALSE, FALSE, TRUE, FALSE, FALSE, FALSE, FALSE, FALSE, FALSE, FALSE, FALSE, FALSE, FALSE], "DIO64 Line 3"=[FALSE, FALSE, FALSE, FALSE, FALSE, FALSE, FALSE, FALSE, FALSE, FALSE, FALSE, FALSE, FALSE, FALSE, FALSE, FALSE], "DIO64 Line 4"=[FALSE, FALSE, FALSE, FALSE, FALSE, FALSE, FALSE, FALSE, FALSE, FALSE, FALSE, FALSE, FALSE, FALSE, FALSE, FALSE]}, {"Begin (ms)"=521.2922, "Duration (ms)"=9.004999999999995, "DIO64 Line 1"=[FALSE, FALSE, FALSE, FALSE, FALSE, FALSE, FALSE, FALSE, FALSE, TRUE, TRUE, FALSE, FALSE, FALSE, FALSE, FALSE], "DIO64 Line 2"=[FALSE, FALSE, FALSE, FALSE, FALSE, FALSE, FALSE, FALSE, FALSE, FALSE, FALSE, FALSE, FALSE, FALSE, FALSE, FALSE], "DIO64 Line 3"=[FALSE, FALSE, FALSE, FALSE, FALSE, FALSE, FALSE, FALSE, FALSE, FALSE, FALSE, FALSE, FALSE, FALSE, FALSE, FALSE], "DIO64 Line 4"=[FALSE, FALSE, FALSE, FALSE, FALSE, FALSE, FALSE, FALSE, FALSE, FALSE, FALSE, FALSE, FALSE, FALSE, FALSE, FALSE]}, {"Begin (ms)"=530.2972, "Duration (ms)"=inf, "DIO64 Line 1"=[FALSE, FALSE, FALSE, FALSE, FALSE, FALSE, FALSE, FALSE, FALSE, FALSE, FALSE, FALSE, FALSE, FALSE, FALSE, FALSE], "DIO64 Line 2"=[FALSE, FALSE, FALSE, FALSE, FALSE, FALSE, FALSE, FALSE, FALSE, FALSE, FALSE, FALSE, FALSE, FALSE, FALSE, FALSE], "DIO64 Line 3"=[FALSE, FALSE, FALSE, FALSE, FALSE, FALSE, FALSE, FALSE, FALSE, FALSE, FALSE, FALSE, FALSE, FALSE, FALSE, FALSE], "DIO64 Line 4"=[FALSE, FALSE, FALSE, FALSE, FALSE, FALSE, FALSE, FALSE, FALSE, FALSE, FALSE, FALSE, FALSE, FALSE, FALSE, FALSE]}] caption="DIO64 Debug"
  in  "dac:kick":T9(array[cluster])=[{"Name"="Fast", "DAC"=[{"Time"=0.0, "Voltage"=[-2.17, -0.11, 2.69, 2.17, 0.11, -2.689999999999999]}, {"Time"=1.19, "Voltage"=[-2.17, -0.11, 2.69, 2.17, 0.11, -2.689999999999999]}, {"Time"=1.2, "Voltage"=[0.0, -6.0, -6.0, 0.0, 6.0, 6.0]}]}, {"Name"="IMG", "DAC"=[{"Time"=0.0, "Voltage"=[-2.17, -0.11, 2.69, 2.17, 0.11, -2.689999999999999, 0.0]}, {"Time"=1.19, "Voltage"=[-2.17, -0.11, 2.689999999999999, 2.17, 0.11, -2.689999999999999, 0.0]}, {"Time"=1.2, "Voltage"=[6.0, 0.0, -6.0, -6.0, 0.0, 6.0, 0.0]}]}, {"Name"="Zero", "DAC"=[{"Time"=0.0, "Voltage"=[0.0, 0.0, 0.0, 0.0, 0.0, 0.0, 0.0, 0.25]}]}, {"Name"="Shim IMG Simple", "DAC"=[{"Time"=0.0, "Voltage"=[-0.002, 0.022, 0.022, 0.002, -0.022, -0.022, -0.47, 0.25]}, {"Time"=1.0, "Voltage"=[-0.002, 0.022, 0.022, 0.002, -0.022, -0.022, -0.47, 0.25]}, {"Time"=2.0, "Voltage"=[-0.1, 0.013000000000000001, 0.013000000000000001, -0.1, -0.013000000000000001, -0.013000000000000001, -0.481, 0.25]}]}, {"Name"="Zero", "DAC"=[{"Time"=0.0, "Voltage"=[0.0, 0.0, 0.0, 0.0, 0.0, 0.0, 0.0, 0.25]}]}, {"Name"="Relax Trap", "DAC"=[{"Time"=0.0, "Voltage"=[0.006, 0.018, 0.018, -0.006, -0.018, -0.018, -0.49, 0.25]}, {"Time"=1.0, "Voltage"=[0.006, 0.018, 0.018, -0.006, -0.018, -0.018, -0.49, 0.25]}, {"Time"=2.0, "Voltage"=[-0.1, 0.01, 0.01, -0.1, -0.018, -0.018, -0.5, 0.25]}, {"Time"=178.0, "Voltage"=[-0.1, 0.01, 0.01, -0.1, -0.018, -0.018, -0.5, 0.25]}, {"Time"=181.0, "Voltage"=[0.0, -0.04, -0.04, 0.0, -0.068, -0.068, -0.08, 0.25]}, {"Time"=184.0, "Voltage"=[0.0, -0.04, -0.04, 0.0, -0.068, -0.068, -0.08, 0.25]}, {"Time"=187.0, "Voltage"=[-0.1, 0.01, 0.01, -0.1, -0.018, -0.018, -0.5, 0.25]}, {"Time"=5.0, "Voltage"=[-0.1, 0.01, 0.01, -0.1, -0.018, -0.018, -0.5, 0.25]}, {"Time"=175.0, "Voltage"=[-0.1, 0.01, 0.01, -0.1, -0.018, -0.018, -0.5, 0.25]}, {"Time"=177.99, "Voltage"=[-0.1, 0.01, 0.01, -0.1, -0.018, -0.018, -0.5, 0.25]}, {"Time"=220.70000000000005, "Voltage"=[-0.1, 0.01, 0.01, -0.1, -0.018, -0.018, -0.5, 0.25]}, {"Time"=221.0, "Voltage"=[-0.1, 0.07, 0.07, -0.1, 0.042, 0.042, -6.0, 0.25]}]}, {"Name"="Relax Trap IMG", "DAC"=[{"Time"=0.0, "Voltage"=[-0.105, 0.02, 0.02, -0.1, -0.02, -0.02, -0.5, 0.25]}, {"Time"=1.0, "Voltage"=[-0.105, 0.02, 0.02, -0.1, -0.02, -0.02, -0.5, 0.25]}, {"Time"=2.0, "Voltage"=[-0.1, 0.01, 0.01, -0.1, -0.018, -0.018, -0.5, 0.25]}, {"Time"=5.0, "Voltage"=[-0.1055, 0.01, 0.01, -0.1, -0.018, -0.018, -0.10000000000000003, 0.25]}, {"Time"=67.0, "Voltage"=[-0.1055, 0.01, 0.01, -0.1, -0.018, -0.018, -0.10000000000000003, 0.25]}, {"Time"=70.0, "Voltage"=[-0.1, 0.01, 0.01, -0.1, -0.018, -0.018, -0.5, 0.25]}, {"Time"=70.7, "Voltage"=[-0.1, 0.01, 0.01, -0.1, -0.018, -0.018, -0.5, 0.25]}, {"Time"=71.0, "Voltage"=[-0.1, 0.07, 0.07, -0.1, 0.042, 0.042, -6.0, 0.25]}]}] caption="DAC Kick"
  in  "dac:tasks":T9(array[cluster])=[{"Name"="Zero", "DAC"=[{"Time"=0.0, "Voltage"=[0.0, 0.0, 0.0, 0.0, 0.0, 0.0, 0.0, 0.0]}]}, {"Name"="Initial", "DAC"=[{"Time"=0.0, "Voltage"=[0.044099999999999986, 0.005300000000000008, 0.0053, -0.044099999999999986, -0.005299999999999994, -0.005299999999999994, -0.11000999999999994, -0.12900999999999993]}, {"Time"=2.0, "Voltage"=[0.044099999999999986, 0.005300000000000008, 0.005300000000000008, -0.044099999999999986, -0.005299999999999994, -0.005299999999999994, -0.11000999999999994, -0.12900999999999993]}, {"Time"=10.0, "Voltage"=[0.034099999999999984, 0.0012100000000000025, 0.0012100000000000051, -0.034099999999999984, -0.0012100000000000051, -0.0012100000000000051, -0.06390999999999997, -0.07711000000000007]}]}, {"Name"="Dissociation 2", "DAC"=[{"Time"=2.0, "Voltage"=[0.0, 0.0, 0.0, 0.0, 0.0, 0.0, -3.5999999999999996, -3.5999999999999996]}, {"Time"=2.1, "Voltage"=[0.0, 0.0, 0.0, 0.0, 0.0, 0.0, -3.5999999999999996, -3.5999999999999996]}, {"Time"=4.1, "Voltage"=[0.034099999999999984, 0.0012100000000000025, 0.0012100000000000051, -0.034099999999999984, -0.0012100000000000051, -0.0012100000000000051, -0.09390999999999995, -0.10711000000000005]}]}, {"Name"="Dissociation", "DAC"=[{"Time"=2.0, "Voltage"=[0.0, 0.0, 0.0, 0.0, 0.0, 0.0, -3.5999999999999996, -3.5999999999999996]}, {"Time"=2.0999999999999996, "Voltage"=[0.0, 0.0, 0.0, 0.0, 0.0, 0.0, -3.5999999999999996, -3.5999999999999996]}, {"Time"=4.1, "Voltage"=[0.034099999999999984, 0.0012100000000000025, 0.0012100000000000051, -0.034099999999999984, -0.0012100000000000051, -0.0012100000000000051, -0.09390999999999995, -0.10711000000000005]}]}, {"Name"="Kick X", "DAC"=[{"Time"=0.002, "Voltage"=[0.0321, 0.20531000000000002, 0.20531000000000002, -0.0321, -0.20531000000000002, -0.20531000000000002, -0.06810999999999996, -0.09291000000000006]}, {"Time"=0.004, "Voltage"=[0.0321, 0.005310000000000003, 0.005310000000000003, -0.0321, -0.005310000000000003, -0.005310000000000003, -0.06810999999999996, -0.09291000000000006]}]}, {"Name"="Kick Y", "DAC"=[{"Time"=0.01, "Voltage"=[-0.09999999999999999, 0.0117, 0.0117, 0.09999999999999999, -0.0117, -0.0117, -0.0777, -0.1313]}, {"Time"=0.02, "Voltage"=[-0.0189, 0.011699999999999995, 0.011699999999999995, 0.0191, -0.011699999999999995, -0.011699999999999995, -0.07769999999999994, -0.13130000000000003]}]}, {"Name"="Kick Z", "DAC"=[{"Time"=0.0, "Voltage"=[0.027000000000000003, 0.005399999999999997, 0.005399999999999997, 0.013000000000000001, -0.0254, -0.0254, -0.045000000000000005, -0.084]}, {"Time"=0.002, "Voltage"=[0.027000000000000003, 0.005399999999999997, 0.005399999999999997, 0.013000000000000001, -0.0254, -0.0254, 0.355, -0.484]}, {"Time"=0.004, "Voltage"=[0.027000000000000003, 0.005399999999999997, 0.005399999999999997, 0.013000000000000001, -0.0254, -0.0254, -0.045000000000000005, -0.084]}]}, {"Name"="Unrelax", "DAC"=[{"Time"=0.0, "Voltage"=[0.034099999999999984, 0.0012100000000000025, 0.0012100000000000051, -0.034099999999999984, -0.0012100000000000051, -0.0012100000000000051, -0.06390999999999997, -0.07711000000000007]}, {"Time"=5.0, "Voltage"=[0.034099999999999984, 0.0012100000000000025, 0.0012100000000000051, -0.034099999999999984, -0.0012100000000000051, -0.0012100000000000051, -0.09390999999999995, -0.10711000000000005]}]}, {"Name"="Kick XYZ", "DAC"=[{"Time"=0.002, "Voltage"=[0.1321, 0.10531000000000001, 0.10531000000000001, -0.1321, -0.10531000000000001, -0.10531000000000001, 0.03189000000000004, -0.19291000000000008]}, {"Time"=0.004, "Voltage"=[0.0321, 0.005310000000000003, 0.005310000000000003, -0.0321, -0.005310000000000003, -0.005310000000000003, -0.06810999999999996, -0.09291000000000006]}]}, {"Name"="Move z", "DAC"=[{"Time"=0.0, "Voltage"=[0.034099999999999984, 0.0012100000000000025, 0.0012100000000000051, -0.034099999999999984, -0.0012100000000000051, -0.0012100000000000051, -0.06390999999999997, -0.07711000000000007]}, {"Time"=5.0, "Voltage"=[0.034099999999999984, 0.0012100000000000025, 0.0012100000000000051, -0.034099999999999984, -0.0012100000000000051, -0.0012100000000000051, -0.05890999999999996, -0.08211000000000007]}]}, {"Name"="Return z", "DAC"=[{"Time"=0.0, "Voltage"=[0.034099999999999984, 0.0012100000000000025, 0.0012100000000000051, -0.034099999999999984, -0.0012100000000000051, -0.0012100000000000051, -0.05890999999999996, -0.08211000000000007]}, {"Time"=5.0, "Voltage"=[0.034099999999999984, 0.0012100000000000025, 0.0012100000000000051, -0.034099999999999984, -0.0012100000000000051, -0.0012100000000000051, -0.06390999999999997, -0.07711000000000007]}]}, {"Name"="Move x", "DAC"=[{"Time"=0.0, "Voltage"=[0.027000000000000003, 0.005399999999999997, 0.005399999999999997, 0.013000000000000001, -0.0254, -0.0254, -0.045000000000000005, -0.084]}, {"Time"=5.0, "Voltage"=[0.026999999999999996, 0.0104, 0.0104, 0.013, -0.030400000000000003, -0.030400000000000003, -0.045000000000000005, -0.084]}]}, {"Name"="Return x", "DAC"=[{"Time"=0.0, "Voltage"=[0.026999999999999996, 0.010399999999999998, 0.010399999999999998, 0.013, -0.030399999999999996, -0.030399999999999996, -0.045000000000000005, -0.084]}, {"Time"=5.0, "Voltage"=[0.027000000000000003, 0.005399999999999997, 0.005399999999999997, 0.013000000000000001, -0.0254, -0.0254, -0.045000000000000005, -0.084]}]}, {"Name"="Move y", "DAC"=[{"Time"=0.0, "Voltage"=[0.0321, 0.005310000000000003, 0.005310000000000003, -0.0321, -0.005310000000000003, -0.005310000000000003, -0.06810999999999996, -0.09291000000000006]}, {"Time"=5.0, "Voltage"=[0.0421, 0.005310000000000003, 0.005310000000000003, -0.0421, -0.005310000000000003, -0.005310000000000003, -0.06810999999999996, -0.09291000000000006]}]}, {"Name"="Return y", "DAC"=[{"Time"=0.0, "Voltage"=[0.042100000000000005, 0.005310000000000003, 0.005310000000000003, -0.0421, -0.005310000000000003, -0.005310000000000003, -0.06810999999999996, -0.09291000000000006]}, {"Time"=5.0, "Voltage"=[0.0321, 0.005310000000000003, 0.005310000000000003, -0.0321, -0.005310000000000003, -0.005310000000000003, -0.06810999999999996, -0.09291000000000006]}]}] caption="DAC Tasks"
  in  "dac":T10(array[cluster])=[{"Task"="Initial", "Reference"="T0", "Begin"=0.0, "Chops"=[FALSE, FALSE, FALSE, FALSE, FALSE, FALSE, FALSE, FALSE, FALSE, FALSE, FALSE, FALSE]}, {"Task"="Dissociation", "Reference"="T0", "Begin"=399.0, "Chops"=[FALSE, FALSE, FALSE, FALSE, FALSE, FALSE, FALSE, FALSE, FALSE, FALSE, FALSE, FALSE]}, {"Task"="Dissociation 2", "Reference"="Dissociation", "Begin"=33.33, "Chops"=[FALSE, FALSE, FALSE, FALSE, FALSE, FALSE, FALSE, FALSE, FALSE, FALSE, FALSE, FALSE]}, {"Task"="Dissociation 2", "Reference"="Dissociation", "Begin"=66.67, "Chops"=[FALSE, FALSE, FALSE, FALSE, FALSE, FALSE, FALSE, FALSE, FALSE, FALSE, FALSE, FALSE]}, {"Task"="Dissociation 2", "Reference"="Dissociation", "Begin"=100.0, "Chops"=[FALSE, FALSE, FALSE, FALSE, FALSE, FALSE, FALSE, FALSE, FALSE, FALSE, FALSE, FALSE]}, {"Task"="Unrelax", "Reference"="Dissociation", "Begin"=-6.0, "Chops"=[FALSE, FALSE, FALSE, FALSE, FALSE, FALSE, FALSE, FALSE, FALSE, FALSE, FALSE, FALSE]}, {"Task"="Move z", "Reference"="T0", "Begin"=114.0, "Chops"=[FALSE, FALSE, FALSE, FALSE, FALSE, FALSE, FALSE, FALSE, FALSE, FALSE, FALSE, FALSE]}, {"Task"="Return z", "Reference"="T0", "Begin"=377.42, "Chops"=[FALSE, FALSE, FALSE, FALSE, FALSE, FALSE, FALSE, FALSE, FALSE, FALSE, FALSE, FALSE]}] caption="DAC Schedule" {"Begin" format="%#_8g"}
  in  "switches":T11={"Brot"={"in"=-0.235, "out"=0.2, "channel"="DAC_KICK/ao7", "delay"=200}, "Doublet"={"upper"=168.18, "lower"=189.79, "DurationUpper"=1.16, "DurationLower"=0.95, "Upper T"=256.0, "Lower T"=256.0}, "Rotation"={"Down"=[{"Frequency"=250.0, "Phase"=420.0, "Amplitude"=0.993}, {"Frequency"=250.0, "Phase"=358.58, "Amplitude"=0.991}, {"Frequency"=250.0, "Phase"=300.54, "Amplitude"=0.984}, {"Frequency"=250.0, "Phase"=239.9, "Amplitude"=1.0}, {"Frequency"=250.0, "Phase"=180.05, "Amplitude"=0.988}, {"Frequency"=250.0, "Phase"=120.63, "Amplitude"=0.987}, {"Frequency"=250.0, "Phase"=0.0, "Amplitude"=0.0}, {"Frequency"=250.0, "Phase"=70.0, "Amplitude"=0.0}], "Up"=[{"Frequency"=250.0, "Phase"=0.0, "Amplitude"=0.996}, {"Frequency"=250.0, "Phase"=58.64, "Amplitude"=0.991}, {"Frequency"=250.0, "Phase"=120.56, "Amplitude"=0.984}, {"Frequency"=250.0, "Phase"=179.79, "Amplitude"=1.0}, {"Frequency"=250.0, "Phase"=239.66, "Amplitude"=0.992}, {"Frequency"=250.0, "Phase"=300.48, "Amplitude"=0.985}, {"Frequency"=250.0, "Phase"=0.0, "Amplitude"=0.0}, {"Frequency"=250.0, "Phase"=70.0, "Amplitude"=0.0}]}, "Depletion phase"={"0 phase"=0.0, "pi phase"=180.0}} caption="Switch Settings" {"Depletion phase"."pi phase" format="%#_8g"; "Depletion phase"."0 phase" format="%#_8g"; "Rotation"."Up"."Amplitude" min=0.0 max=1.0 step=0.0001 format="%#_10g"; "Rotation"."Up"."Phase" format="%.2f"; "Rotation"."Up"."Frequency" format="%#_10g"; "Rotation"."Down"."Amplitude" min=0.0 max=1.0 step=0.0001 format="%#_10g"; "Rotation"."Down"."Phase" format="%.2f"; "Rotation"."Down"."Frequency" format="%#_10g"; "Doublet"."Lower T" format="%#_8g"; "Doublet"."Upper T" format="%#_8g"; "Doublet"."DurationLower" format="%#_8g"; "Doublet"."DurationUpper" format="%#_8g"; "Doublet"."lower" format="%.9g"; "Doublet"."upper" format="%.9g"}
  in  "scope:channels":T12(array[ring])
  out "scope":waveform(dbl)[](graph)
  in  "scope:resource":refnum<visa-resource-name>="USB0::0x0699::0x0408::C012037::INSTR"
  in  "test commands":string="Frames >> 1,1\nScope: Settings >> TDS5034B\nScope: Trigger Settings >> TDS5034B\n\nMacro: Clear Wavelengths\nMacro: Read Wavelengths\nMagnetometer: Measure\n\nTrap DDS: Upload\nTrap DDS: Upload Ramp\n\nDAC: Upload2 >> 0,Fast\n#MV500: Trigger\n#DAC: Upload2 >> 0,IMG\n\n#Scan: Reset\nScope: Start >> TDS5034B\n\nDIO64: Prepare >> 1\nDIO64: Run\nScope: Read >> TDS5034B\nScope: Stop >> TDS5034B\nScope: Display Traces >> TDS5034B\n\nCount Ions\n\n#DIO64: Override\n" caption="Test Commands"
  out "queue":string[](array[string])
  out "current state":string="Exit"
  out "debug timing":cluster{"command":string, "time":dbl}[](array[cluster])=[{"command"="Data: Initialize", "time"=0.0}, {"command"="Data: Cleanup", "time"=0.0}, {"command"="UI: Initialize", "time"=0.0}, {"command"="UI: Cursor Set", "time"=0.0}, {"command"="UI: Front Panel State", "time"=13.0}, {"command"="UI: Get Case Strings", "time"=0.0}, {"command"="UI: Get Case Documentation", "time"=0.0}, {"command"="UI: DIO64 Update Control", "time"=0.0}, {"command"="UI: DIO64 Labels", "time"=0.0}, {"command"="UI: Chop Labels", "time"=0.0}, {"command"="Macro: Initialize", "time"=0.0}, {"command"="Macro: Exit", "time"=3.0}, {"command"="delay", "time"=0.0}, {"command"="stdout", "time"=0.0}, {"command"="Abort", "time"=0.0}, {"command"="Test", "time"=0.0}, {"command"="Pause", "time"=0.0}, {"command"="Sync", "time"=0.0}, {"command"="uBinary: Load", "time"=79126.0}, {"command"="uBinary", "time"=0.0}, {"command"="DIO64: Initialize", "time"=0.0}, {"command"="DIO64: Prepare", "time"=0.0}, {"command"="DIO64: Update Graph", "time"=0.0}, {"command"="DIO64: Run", "time"=0.0}, {"command"="DIO64: Override", "time"=0.0}, {"command"="DIO64: Close", "time"=0.0}, {"command"="Scope: Initialize", "time"=0.0}, {"command"="Scope: Settings", "time"=0.0}, {"command"="Scope: Read", "time"=0.0}, {"command"="Scope: Close", "time"=0.0}] caption="Debug Timing"
  out "stdout":string
  out "documentation:display":string caption="Documentation"
  in  "states":i32(listbox) caption="States"
  out "documentation":string[](array[string])=["Initialize the shift-register data, here.\n(data names are defined by what you wire into the bundle function)", "Cleanup any data and references, here.\n(this is called automatically, by the Macro: Exit)", "Initialize the User Interface, here.\n(this is called automatically, by the Macro: Init)", "Set and Unset Cursor Busy.\n(Usage: \"UI: Cursor Set >> Busy|Idle\")", "Argument", "Gets the program states from the main loop case selector\n(Usage: \"UI: Get Case Strings\")", "Gets program documentation from main loop case selector\n(Usage: \"UI: Get Case Documentation\")", "Updates DIO64 control with string from DIO64 Tasks\n(Usage: \"call after any modification to DIO64 Tasks\")", "Updates DIO64 control with string from DIO64 Tasks\n(Usage: \"call after any modification to DIO64 Tasks\")", "Updates DIO64 control with string from DIO64 Tasks\n(Usage: \"call after any modification to DIO64 Tasks\")", "Initialization Macro\n(This is called once, when the VI starts. It calls a number of other program states.)", "Exit Macro\n(This is called once, when the VI exits)", "Delays for some number of milliseconds\n(Usage: delay >>  TIME)", "Prints a message to the labview stdout control\n(Usage: stdout >> TEXT)", "Clears the queue\n(Usage: abort)", "Runs the test sequence\n(Usage: Test)", "Pauses the state machine\n(swaps out the queue to memory)", "Pauses the state machine\n(swaps out the queue to memory)", "Pauses the state machine\n(swaps out the queue to memory)", "Pauses the state machine\n(swaps out the queue to memory)", "Initialize the DIO64", "Parses the DIO64\n(Usage: DIO64: Prepare >> CHOP)", "Updates the DIO64 Timing Graph\n(Usage: call whenever the DIO64 changes)", "Runs the DIO64\n(Usage: DIO64: Run )\n(Usage: DIO64: Run >> Chop,CHOP to run CHOP a number of times in the frame control)\n(Usage: DIO64: Run >> Repeat,N, to run the prepared sequence N times)", "DIO64: Override\n(Usage: DIO64: Override >> CHANNEL, to run a channel like A0 or C6)", "Closes the DIO64\n(Usage: DIO64: Close)", "Initalize the Scope\n(Usage: Scope: Initialize >> SCOPE, where SCOPE can be DPO)", "Updates Scope Settings\n(Usage: Scope: Settings >> SCOPE, where SCOPE can be DPO)", "Reads a frame from the Scope\n(Usage: Scope: Read >> SCOPE, where SCOPE can be DPO)", "Close the Scope\n(Usage: Scope: Close >> SCOPE, where SCOPE can be DPO)"] caption="Documentation"
  # "Task Name"
  # "Start (ms)"
  # "Edge"
  # "Reference"
  # "End (ms)"
  # "Edge"
  # "Reference"
  # "0"
  # "1"
  # "2"
  # "3"
  # "4"
  # "5"
  # "6"
  # "7"
  # "8"
  # "9"
  # "10"
  # "11"
  # "A00"
  # "A01"
  # "A02"
  # "A03"
  # "A04"
  # "A05"
  # "A06"
  # "A07"
  # "A08"
  # "A09"
  # "A10"
  # "A11"
  # "A12"
  # "A13"
  # "A14"
  # "A15"
  # "B00"
  # "B01"
  # "B02"
  # "B03"
  # "B04"
  # "B05"
  # "B06"
  # "B07"
  # "B08"
  # "B09"
  # "B10"
  # "B11"
  # "B12"
  # "B13"
  # "B14"
  # "B15"
  # "C00"
  # "C01"
  # "C02"
  # "C03"
  # "C04"
  # "C05"
  # "C06"
  # "C07"
  # "C08"
  # "C09"
  # "C10"
  # "C11"
  # "C12"
  # "C13"
  # "C14"
  # "C15"
  # "D00"
  # "D01"
  # "D02"
  # "D03"
  # "D04"
  # "D05"
  # "D06"
  # "D07"
  # "D08"
  # "D09"
  # "D10"
  # "D11"
  # "D12"
  # "D13"
  # "D14"
  # "D15"
  # "Time (ms)"
  # "A0"
  # "A1"
  # "A2"
  # "A3"
  # "A4"
  # "A5"
  # "A6"
  # "Time (ms)"
  # "A0"
  # "A1"
  # "A2"
  # "A3"
  # "A4"
  # "A5"
  # "A6"
  # "A7"
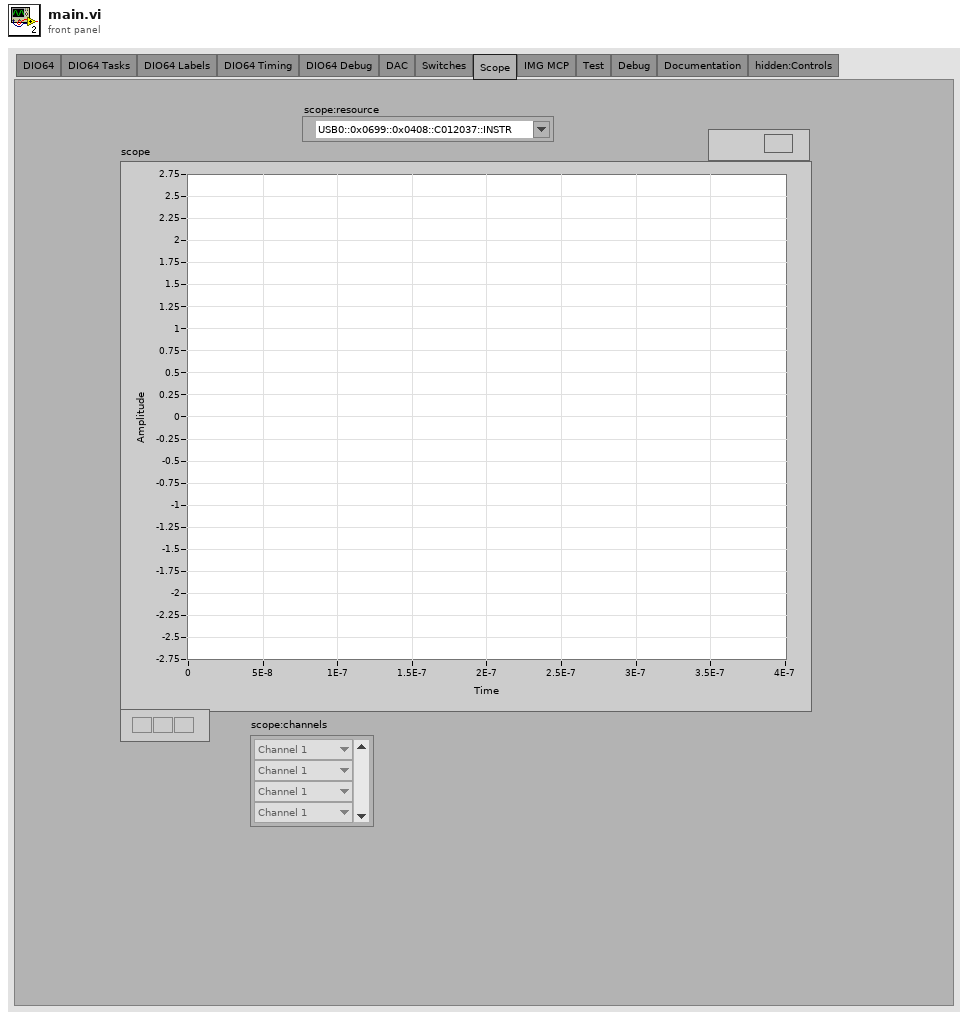
[diagram p1: front panel]
types:
  T1 = enum32{"DIO64", "DIO64 Tasks", "DIO64 Labels", "DIO64 Timing", "DIO64 Debug", "DAC", "Switches", "Scope", "IMG MCP", "Test", "Debug", "Documentation", "hidden:Controls"}
  T2 = cluster{"Task":string, "begin time":dbl, "begin edge":bool, "begin reference":string, "end time":dbl, "end edge":bool, "end reference":string, "Chops":bool[]}[]
  T3 = cluster{"Name":string, "DIO64 Line 1":bool[], "DIO64 Line 2":bool[], "DIO64 Line 3":bool[], "DIO64 Line 4":bool[]}[]
  T4 = cluster{"Channel 1":picture[], "Channel 2":picture[], "Channel 3":picture[], "Channel 4":picture[]}
  T5 = cluster{"Channel":string, "Name":string, "plot":bool}[][]
  T6 = cluster{"DIO64 Line 1":bool[], "DIO64 Line 2":bool[], "DIO64 Line 3":bool[], "DIO64 Line 4":bool[]}
  T7 = cluster{"Task":string, "begin time":dbl, "end time":dbl, "Chops":bool[]}[]
  T8 = cluster{"Begin (ms)":dbl, "Duration (ms)":dbl, "DIO64 Line 1":bool[], "DIO64 Line 2":bool[], "DIO64 Line 3":bool[], "DIO64 Line 4":bool[]}[]
  T9 = cluster{"Name":string, "DAC":cluster{"Time":dbl, "Voltage":dbl[]}[]}[]
  T10 = cluster{"Task":string, "Reference":string, "Begin":sgl, "Chops":bool[]}[]
  T11 = cluster{"Brot":cluster{"in":dbl, "out":dbl, "channel":tag, "delay":u32}, "Doublet":cluster{"upper":dbl, "lower":dbl, "DurationUpper":dbl, "DurationLower":dbl, "Upper T":dbl, "Lower T":dbl}, "Rotation":cluster{"Down":cluster{"Frequency":dbl, "Phase":dbl, "Amplitude":dbl}[], "Up":cluster{"Frequency":dbl, "Phase":dbl, "Amplitude":dbl}[]}, "Depletion phase":cluster{"0 phase":dbl, "pi phase":dbl}}
  T12 = enum16{"Channel 1", "Channel 2", "Channel 3", "Channel 4", "Math", "Reference 1", "Reference 2", "Reference 3", "Reference 4", "D0", "D1", "D2", "D3", "D4", "D5", "D6", "D7", "D8", "D9", "D10", "D11", "D12", "D13", "D14", "D15", "Amplitude", "Frequency", "Phase", "Normal", "Average", "Maximum Peak Hold", "Minimum Peak Hold"}[]
  T13 = cluster{"32bit integer":i32, "32bit integer":u16}
  T14 = cluster{"Task":string, "begin time":dbl, "begin edge":bool, "begin reference":string, "end time":dbl, "end edge":bool, "end reference":string, "Chops":bool[]}
  T15 = cluster{"Name":string, "DIO64 Line 1":bool[], "DIO64 Line 2":bool[], "DIO64 Line 3":bool[], "DIO64 Line 4":bool[]}
  T16 = typedef "Rendezvous RefNum" = refnum<k1>
  T17 = enum32{"invalid app kind", "Development System", "Run Time System", "Student Edition", "Embedded LabVIEW", "Evaluation", "Custom"}
  T18 = enum32{"Invalid", "Standard", "Closed", "Hidden", "Minimized", "Maximized"}
  T19 = cluster{"Font Name:":string, "Size":i16, "Strikeout?":bool, "Italic?":bool, "Underline?":bool, "Outline?":bool, "Shadow?":bool, "Bold?":bool}
  T20 = enum16{"User-specified Font", "Application Font", "System Font", "Dialog Font"}
  T21 = enum16{"None", "Stacked", "Clockwise", "Counterclockwise"}
  T22 = cluster{"horizontal":enum16{"left", "center", "right"}, "vertical":enum16{"top", "center", "bottom"}}
  T23 = enum32{"invalid OS target", "Mac OS", "Windows 3.1", "Windows 95/NT", "Solaris 1", "Solaris 2", "HP-UX", "PowerMAX", "Linux", "Irix", "Rhapsody", "BeOS", "AIX", "OSF1", "VxWorks", "PharLap", "Carbon", "RTX", "Windows x64", "Linux x64"}
  T24 = cluster{"Core":cluster{"Current VI Reference":refnum<vi>, "Close Panel on Exit?":bool}, "case labels":string[], "scope:resource":refnum<visa-resource-name>, "pause queue":string[]}
  T25 = typedef "DialogType.ctl" = u16
  T26 = cluster{"Current VI Reference":refnum<vi>, "Close Panel on Exit?":bool}
  T27 = cluster{"Channel":string, "Name":string, "plot":bool}[]
  T28 = cluster{"Begin (ms)":dbl, "Begin (ms)":dbl, "DIO64 Line 4":bool[], "DIO64 Line 4":bool[], "DIO64 Line 4":bool[], "DIO64 Line 4":bool[]}
  T29 = cluster{"Begin (ms)":dbl, "Begin (ms)":dbl, "DIO64 Line 4":bool[], "DIO64 Line 4":bool[], "DIO64 Line 4":bool[], "DIO64 Line 4":bool[]}[]
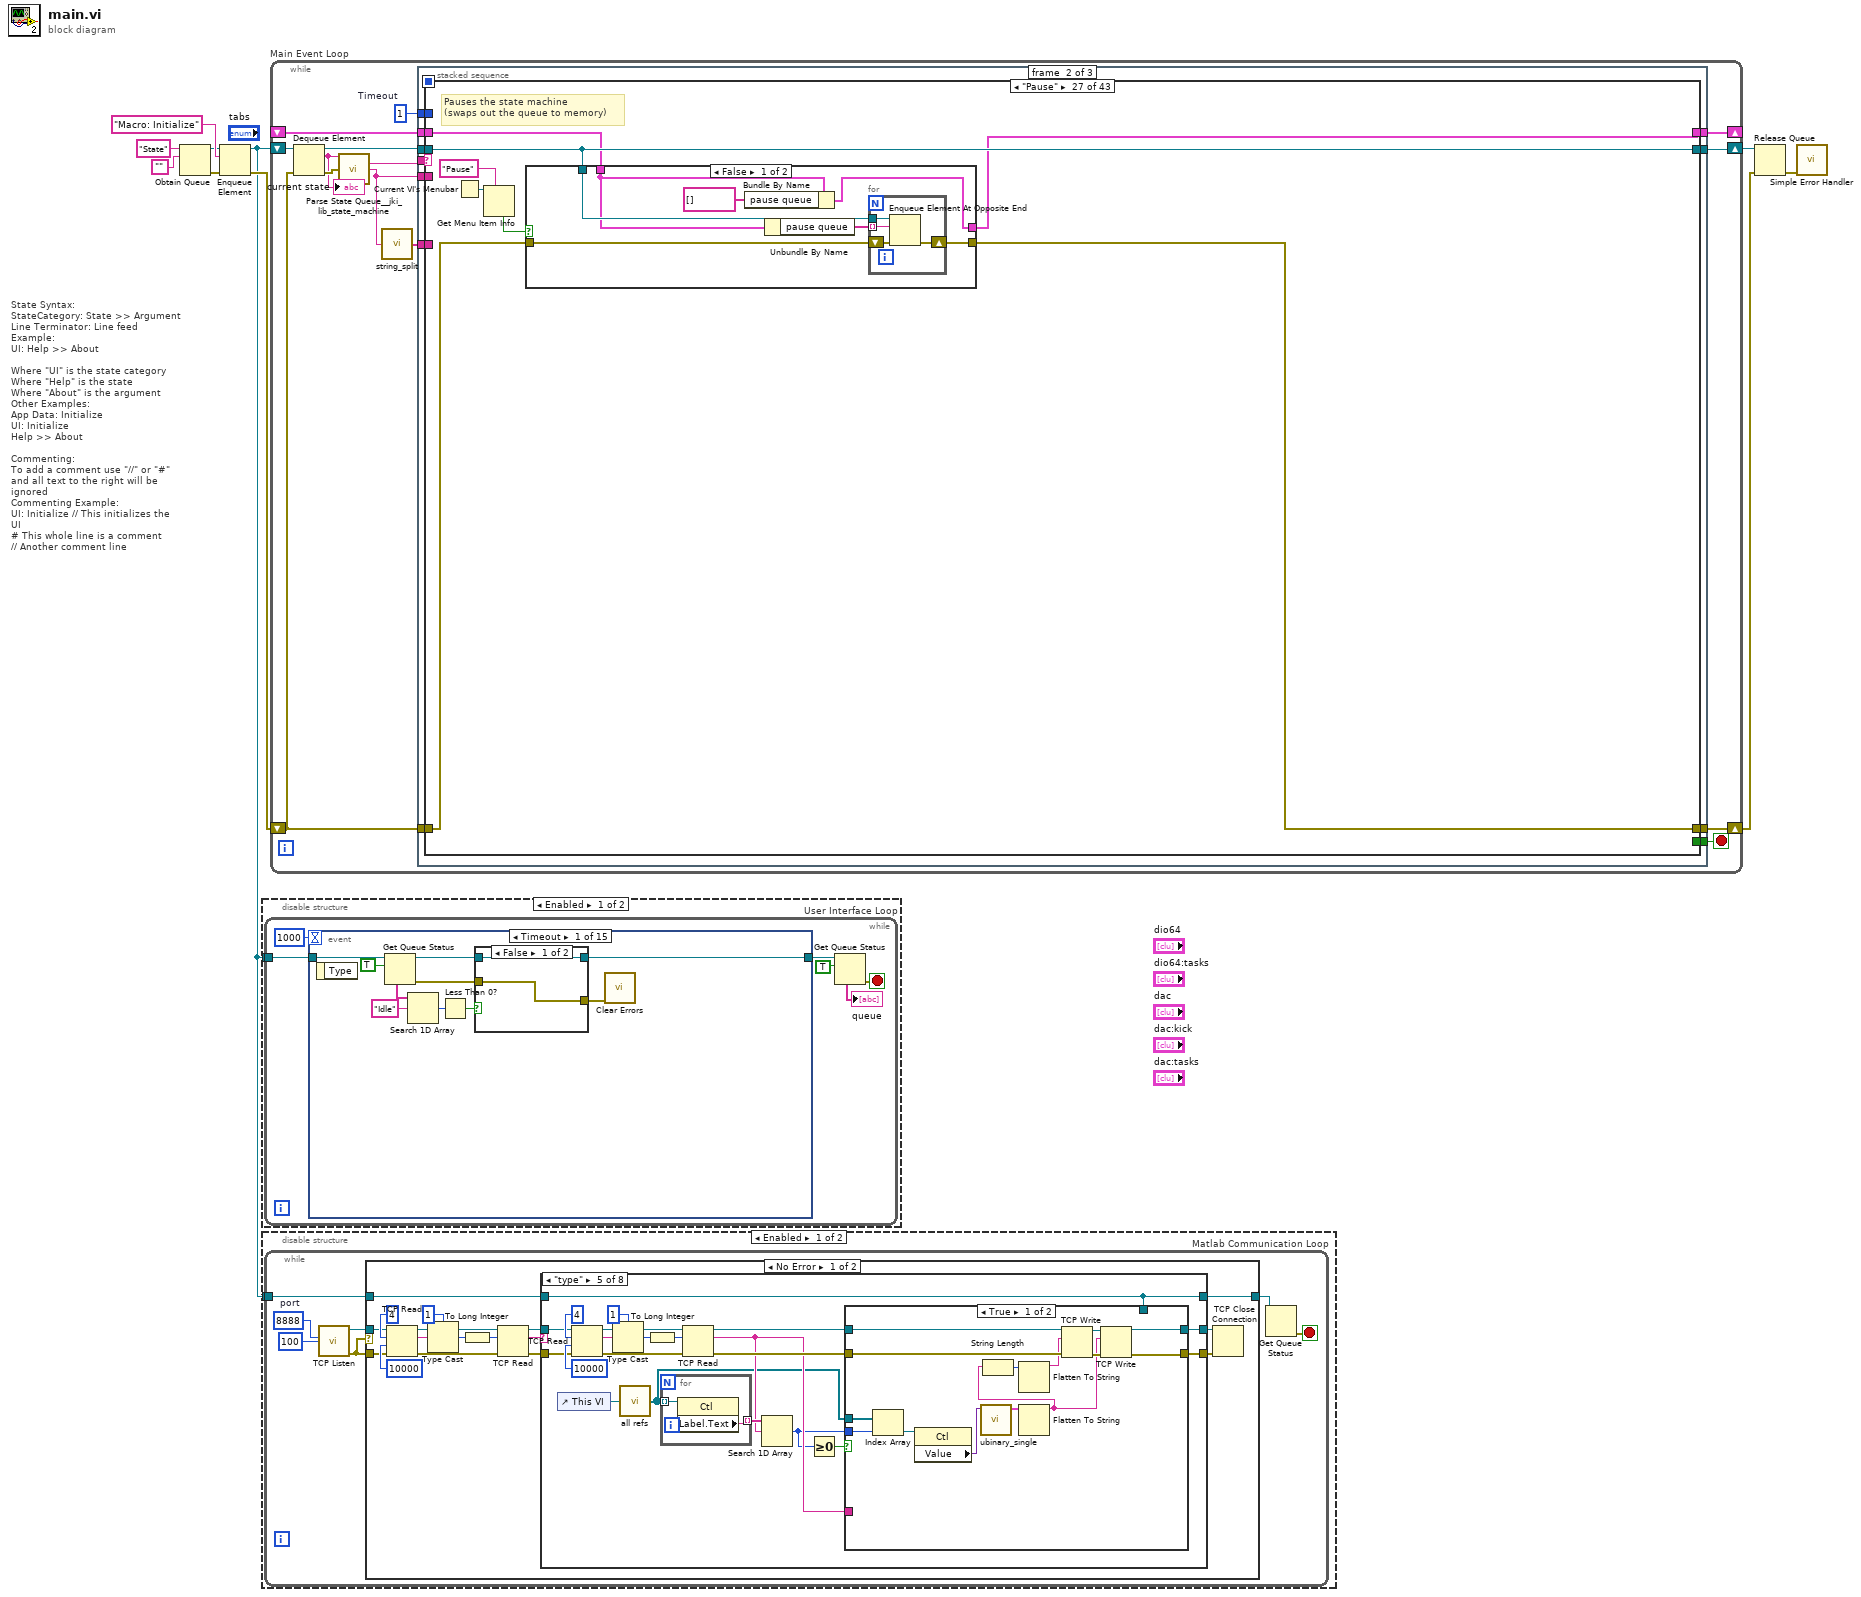
[diagram p0: block diagram]
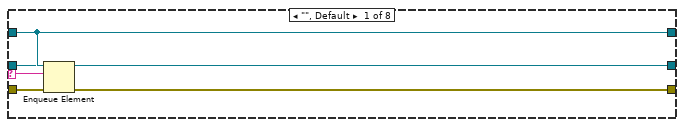
[diagram p2: hidden frame]
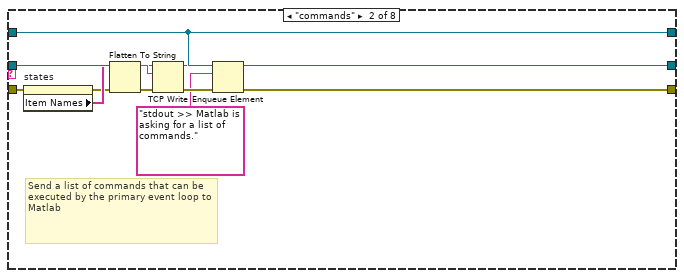
[diagram p3: hidden frame]
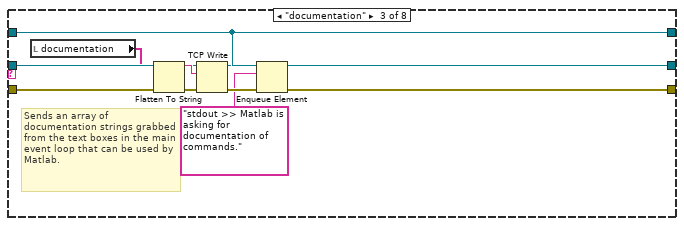
[diagram p4: hidden frame]
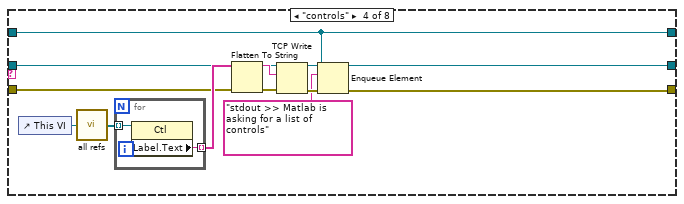
[diagram p5: hidden frame]
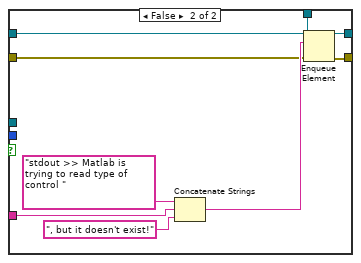
[diagram p6: hidden frame]
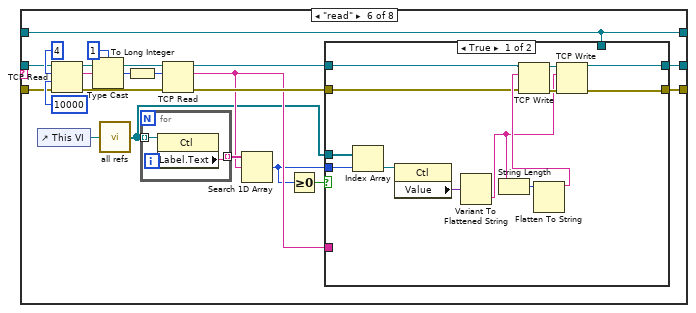
[diagram p7: hidden frame]
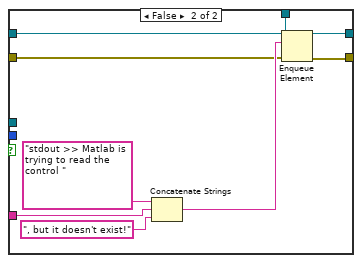
[diagram p8: hidden frame]
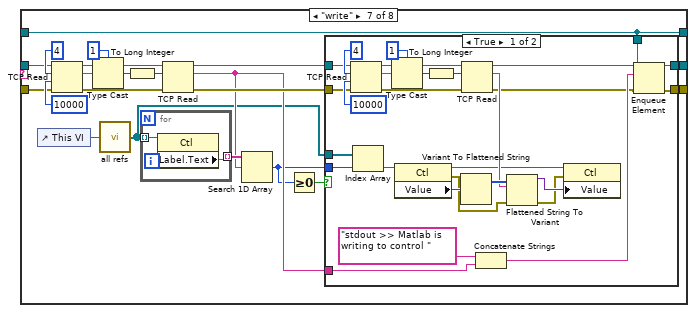
[diagram p9: hidden frame]
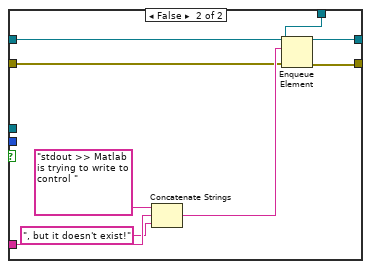
[diagram p10: hidden frame]
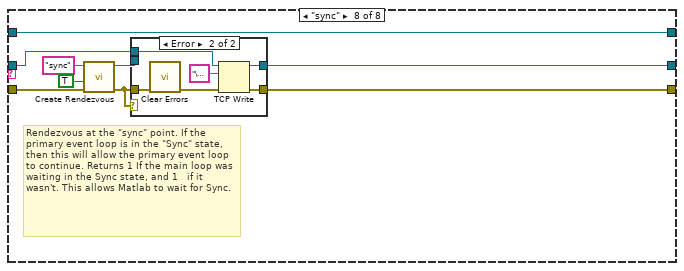
[diagram p11: hidden frame]
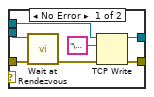
[diagram p12: hidden frame]
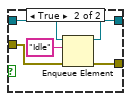
[diagram p15: hidden frame]
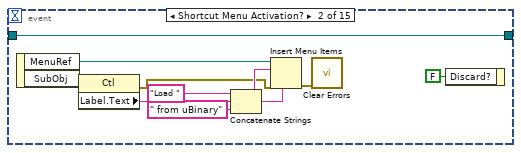
[diagram p16: hidden frame]
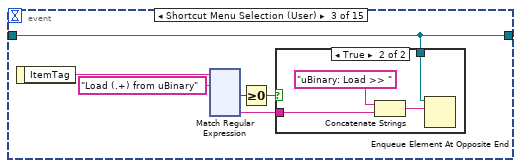
[diagram p17: hidden frame]
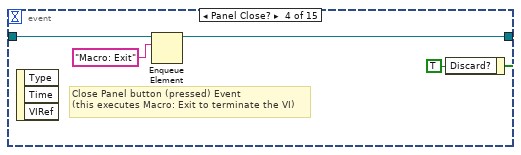
[diagram p19: hidden frame]
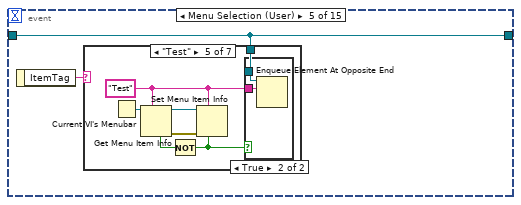
[diagram p20: hidden frame]
diagram:
  # "State Syntax:\nStateCategory: State >> Argument\nLine Terminator: Line feed\nExample:\nUI: Help >> About\n\nWhere \"UI\" is the state category\nWhere \"Help\" is the state\nWhere \"About\" is the argument\nOther Examples:\nApp Data: Initialize\nUI: Initialize\nHelp >> About\n\nCommenting:\nTo add a comment use \"//\" or \"#\" and all text to the right will be ignored\nCommenting Example:\nUI: Initialize // This initializes the UI\n# This whole line is a comment\n// Another comment line"
  n1 = Obtain Queue(name (unnamed)="State", element data type="") -> (queue out=w2:refnum<queue>, error out=w7:errorcluster)  [unwired: 3 in, 1 out]
  n2 = Enqueue Element(queue=w2, element="Macro: Initialize", error in (no error)=w7) -> (queue out=w1:refnum<queue>, error out=w6:errorcluster)  [unwired: 1 in, 1 out]
  n3 = disable-structure shown="Enabled" {
    disable-tunnel: w1 -> [w11 _]
    frame Enabled {
      n4 = while "User Interface Loop" {
        tunnel: w11 -> [w17]
        stop <- w13 stop-if-true
        n5 = event shown="[0] Timeout" {
          selector: _ -> [_ _ _ _ _ _ _ _ _ _ _ _ _ _ _]
          dyn-events: _ -> [_ _ _ _ _ _ _ _ _ _ _ _ _ _ _]
          timeout: 1000 -> [_ _ _ _ _ _ _ _ _ _ _ _ _ _ _]
          tunnel: w17 -> [w27 w43 w46 w169 w172 w201 w204 w220 w252 w261 w262 w309 w318 w323 w326]
          tunnel: [w21 w43 w46 w168 w172 w201 w203 w220 w252 w260 w262 w309 w317 w319 w325] -> w16
          event Timeout {
            n6 = event-data() -> ()  [unwired: 1 in, 1 out]
            n7 = Get Queue Status(queue=w27, return elements? (F)=TRUE) -> (queue out=w22:refnum<queue>, error out=w20:errorcluster, elements=w25:string[])  [unwired: 1 in, 5 out]
            n8 = Search 1D Array(1D array=w25, element="Idle") -> (index of element=w23:i32)  [unwired: 1 in]
            n9 = Less Than 0?(x=w23) -> (x < 0?=w18:bool)
            n10 = case shown="False" w18 {
              tunnel: w22 -> [w29 w34]
              tunnel: [w29 w33] -> w21
              tunnel: w20 -> [w28 w31]
              tunnel: [w28 w30] -> w19
              frame False {
              }
              frame True {
                n11 = Enqueue Element(queue=w34, element="Idle", error in (no error)=w31) -> (queue out=w33:refnum<queue>, error out=w30:errorcluster)  [unwired: 1 in, 1 out]
              }
            }
            n12 = call <vilib>:"Clear Errors.vi"("error in (no error)"=w19) -> ()  [unwired: 6 in, 1 out]
          }
          event Shortcut Menu Activation? {
            n13 = event-data() -> ("MenuRef"=w42:refnum<k9>, "SubObj"=w40:refnum<vi>)  [unwired: 1 in]
            n14 = property class="Ctl"(reference=w40) -> (error out=w36:errorcluster, "Label.Text"=w39:string)  [unwired: 1 in, 1 out]
            n15 = Concatenate Strings("Load ", w39, " from uBinary" ("string")) -> (w37:string)
            n16 = Insert Menu Items(4:w37, 6:w36, 8:w37, 9:w42) -> (0:w35:errorcluster)  [unwired: 2 in, 2 out]
            n17 = call <vilib>:"Clear Errors.vi"("error in (no error)"=w35) -> ()  [unwired: 6 in, 1 out]
            n18 = event-data("Discard?"=FALSE) -> ()  [unwired: 1 in, 1 out]
          }
          event Shortcut Menu Selection (User) {
            n19 = event-data() -> ("ItemTag"=w50:string)  [unwired: 1 in]
            n20 = xnode "Match Regular Expression"("input string"=w50, "regular expression"="Load (.+) from uBinary") -> ("offset past match"=w48:i32, "submatch 1"=w45:string)  [unwired: 4 in, 4 out]
            n21 = Greater Or Equal To 0?(x=w48) -> (x >= 0?=w47:bool)
            n22 = case shown="True" w47 {
              tunnel: w46 -> [_ w54]
              tunnel: w45 -> [_ w52]
              frame False {
              }
              frame True {
                n23 = Concatenate Strings("uBinary: Load >> " ("string"), w52) -> (w53:string)
                n24 = Enqueue Element At Opposite End(queue=w54, element=w53) -> ()  [unwired: 2 in, 3 out]
              }
            }
          }
          event Panel Close? {
            # "Close Panel button (pressed) Event\n(this executes Macro: Exit to terminate the VI)"
            n25 = event-data() -> ()  [unwired: 1 in, 3 out]
            n26 = Enqueue Element(queue=w169, element="Macro: Exit") -> (queue out=w168:refnum<queue>)  [unwired: 2 in, 2 out]
            n27 = event-data("Discard?"=TRUE) -> ()  [unwired: 1 in, 1 out]
          }
          event Menu Selection (User) {
            n28 = event-data() -> ("ItemTag"=w173:string)  [unwired: 1 in]
            n29 = case shown="\"Test\"" w173 {
              tunnel: w172 -> [_ w175 w177 w179 w186 w195 w197]
              frame "", Default {
              }
              frame "Save" {
                n30 = Enqueue Element At Opposite End(queue=w175, element="uBinary: Save") -> ()  [unwired: 2 in, 3 out]
              }
              frame "Load" {
                n31 = Enqueue Element At Opposite End(queue=w177, element="uBinary: Load") -> ()  [unwired: 2 in, 3 out]
              }
              frame "Abort" {
                n32 = Enqueue Element At Opposite End(queue=w179, element="Abort") -> ()  [unwired: 2 in, 3 out]
              }
              frame "Test" {
                w181 = "Test" ("item tag")
                n33 = Current VI's Menubar() -> (w182:refnum<k9>)
                n34 = Get Menu Item Info(7:w181, 11:w182) -> (0:w183:errorcluster, 3:w185:refnum<k9>, 4:w184:bool)  [unwired: 1 in, 4 out]
                n35 = Not(x=w184) -> (.not. x?=w180:bool)
                n36 = Set Menu Item Info(6:w180, 7:w181, 8:w183, 11:w185) -> ()  [unwired: 3 in, 2 out]
                n37 = case shown="True" w180 {
                  tunnel: w186 -> [_ w188]
                  tunnel: w181 -> [_ w187]
                  frame False {
                  }
                  frame True {
                    n38 = Enqueue Element At Opposite End(queue=w188, element=w187) -> ()  [unwired: 2 in, 3 out]
                  }
                }
              }
              frame "Pause" {
                w190 = "Pause" ("item tag")
                n39 = Current VI's Menubar() -> (w191:refnum<k9>)
                n40 = Get Menu Item Info(7:w190, 11:w191) -> (0:w192:errorcluster, 3:w194:refnum<k9>, 4:w193:bool)  [unwired: 1 in, 4 out]
                n41 = Not(x=w193) -> (.not. x?=w189:bool)
                n42 = Set Menu Item Info(6:w189, 7:w190, 8:w192, 11:w194) -> ()  [unwired: 3 in, 2 out]
                n43 = Enqueue Element At Opposite End(queue=w195, element=w190) -> ()  [unwired: 2 in, 3 out]
              }
              frame "Quit" {
                n44 = Enqueue Element At Opposite End(queue=w197, element="Macro: Exit") -> ()  [unwired: 2 in, 3 out]
              }
            }
          }
          event "states": Value Change {
            n45 = event-data() -> ("NewVal"=w198:i32)  [unwired: 1 in]
            n46 = local read "documentation"() -> (w199:string[])
            n47 = Index Array(array=w199, index=w198) -> (element=→"documentation:display":string)
          }
          event "dio64": Value Change {
            n48 = event-data() -> ()  [unwired: 1 in, 1 out]
            n49 = Enqueue Element(queue=w204, element="DIO64: Update Graoh") -> (queue out=w203:refnum<queue>)  [unwired: 2 in, 2 out]
          }
          event "dio64": Mouse Down {
            n50 = event-data() -> ("Button"=w206:u16, "Coords.Vertical"=w205:i32)  [unwired: 1 in]
            n51 = property on="dio64" class="Arr (strict)"() -> ("Number of Rows"=w209:u32, "Index Values"=w216:u32[])  [unwired: 2 in, 2 out]
            n52 = property on="dio64" class="Arr (strict)"() -> ("Top"=w208:i32, "Height"=w207:u32)  [unwired: 2 in, 2 out]
            n53 = Index Array(array=w216) -> (element=w217:u32)  [unwired: 1 in]
            n54 = formula code="Y = (X-T-23)/(H-27);"("H"=w207, "T"=w208, "X"=w205) -> ("Y"=w212:dbl)
            n55 = In Range and Coerce(upper limit=1.0, x=w212, lower limit=0.0) -> (coerced(x)=w213:dbl)  [unwired: 1 out]
            n56 = Multiply(x=w213, y=w209) -> (x*y=w214:dbl)
            n57 = Round Toward -Infinity(1:w214) -> (0:w215:dbl)
            n58 = Add(x=w215, y=w217) -> (x+y=w218:dbl)
            n59 = To Long Integer(number=w218) -> (32bit integer=w219:i32)
            n60 = case shown="12" w206 {
              selector: w206 -> [_ _ w228]
              tunnel: w219 -> [_ w221 w226]
              frame 0, Default {
              }
              frame 3 {
                n61 = local read "dio64"() -> (w223:T2)
                n62 = Delete From Array(array=w223, index=w221) -> (array with subset deleted=w222:T2)  [unwired: 1 in, 1 out]
                n63 = local write "dio64"(w222) -> ()
              }
              frame 12 {
                n64 = Bundle(w226, "Button"=w228) -> (w227:cluster{i32, "Button":u16})  [unwired: 1 in]
                n65 = Bundle("dio64_row_drag", w227) -> (w229:cluster{string, cluster{i32, "Button":u16}})  [unwired: 1 in]
                n66 = Build Array(w229) -> (w224:cluster{string, cluster{i32, "Button":u16}}[])
                n67 = invoke on="dio64" class="Arr (strict)" method="Start Drag"("Data"=w224, "AllowsMove"=enum32{"copy or move", "copy only", "move only"}."move only" ("Drag Mode")) -> ()  [unwired: 3 in, 5 out]
              }
            }
          }
          event "dio64": Drop {
            n68 = event-data() -> ("Coords.Vertical"=w239:i32)  [unwired: 1 in]
            n69 = property on="dio64" class="Arr (strict)"() -> ("Number of Rows"=w242:u32, "Index Values"=w249:u32[])  [unwired: 2 in, 2 out]
            n70 = Bundle("32bit integer"=0, "32bit integer"=u16 0) -> (w235:T13)  [unwired: 1 in]
            n71 = property on="dio64" class="Arr (strict)"() -> ("Top"=w241:i32, "Height"=w240:u32)  [unwired: 2 in, 2 out]
            n72 = Index Array(array=w249) -> (element=w250:u32)  [unwired: 1 in]
            n73 = Get Drag Drop Data(8:w235, 9:"dio64_row_drag" ("data name")) -> (3:w238:T13)  [unwired: 1 in, 1 out]
            n74 = Unbundle(w238) -> ("32bit integer"=w232:i32, "32bit integer"=w233:u16)
            n75 = formula code="Y = (X-T-23)/(H-27);"("H"=w240, "T"=w241, "X"=w239) -> ("Y"=w245:dbl)
            n76 = In Range and Coerce(upper limit=1.0, x=w245, lower limit=0.0) -> (coerced(x)=w246:dbl)  [unwired: 1 out]
            n77 = Multiply(x=w246, y=w242) -> (x*y=w247:dbl)
            n78 = Round Toward -Infinity(1:w247) -> (0:w248:dbl)
            n79 = Add(x=w248, y=w250) -> (x+y=w251:dbl)
            n80 = To Long Integer(number=w251) -> (32bit integer=w231:i32)
            n81 = case shown="2" w233 {
              tunnel: w231 -> [_ w254]
              tunnel: w232 -> [_ w253]
              frame 0, Default {
              }
              frame 2 {
                n82 = local read "dio64"() -> (w256:T2)
                n83 = Delete From Array(array=w256, index=w253) -> (deleted portion=w257:T14, array with subset deleted=w258:T2)  [unwired: 1 in]
                n84 = Insert Into Array(array=w258, index=w254, new element=w257) -> (w255:T2)
                n85 = local write "dio64"(w255) -> ()
              }
            }
            n86 = event-data() -> ()  [unwired: 2 in, 1 out]
          }
          event "dio64:tasks": Value Change {
            n87 = event-data() -> ()  [unwired: 1 in, 5 out]
            n88 = Enqueue Element(queue=w261, element="UI: DIO64 Update Control") -> (queue out=w260:refnum<queue>)  [unwired: 2 in, 2 out]
          }
          event "dio64:tasks": Mouse Down {
            n89 = event-data() -> ("Button"=w264:u16, "Coords.Vertical"=w263:i32)  [unwired: 1 in]
            n90 = property on="dio64:tasks" class="Arr (strict)"() -> ("Top"=w276:i32, "Height"=w277:u32)  [unwired: 2 in, 2 out]
            n91 = property on="dio64:tasks" class="Arr (strict)"() -> ("Number of Rows"=w275:u32, "Index Values"=w268:u32[])  [unwired: 2 in, 2 out]
            n92 = Index Array(array=w268) -> (element=w267:u32)  [unwired: 1 in]
            n93 = formula code="Y = (X-T-23)/(H-27);"("H"=w277, "T"=w276, "X"=w263) -> ("Y"=w272:dbl)
            n94 = In Range and Coerce(upper limit=1.0, x=w272, lower limit=0.0) -> (coerced(x)=w271:dbl)  [unwired: 1 out]
            n95 = Multiply(x=w271, y=w275) -> (x*y=w270:dbl)
            n96 = Round Toward -Infinity(1:w270) -> (0:w269:dbl)
            n97 = Add(x=w269, y=w267) -> (x+y=w266:dbl)
            n98 = To Long Integer(number=w266) -> (32bit integer=w265:i32)
            n99 = case shown="12" w264 {
              selector: w264 -> [_ _ w283]
              tunnel: w265 -> [_ w278 w281]
              frame 0, Default {
              }
              frame 3 {
                n100 = local read "dio64:tasks"() -> (w280:T3)
                n101 = Delete From Array(array=w280, index=w278) -> (array with subset deleted=w279:T3)  [unwired: 1 in, 1 out]
                n102 = local write "dio64:tasks"(w279) -> ()
              }
              frame 12 {
                n103 = Bundle(w281, "Button"=w283) -> (w282:cluster{i32, "Button":u16})  [unwired: 1 in]
                n104 = Bundle("dio64_task_drag", w282) -> (w285:cluster{string, cluster{i32, "Button":u16}})  [unwired: 1 in]
                n105 = Build Array(w285) -> (w284:cluster{string, cluster{i32, "Button":u16}}[])
                n106 = invoke on="dio64:tasks" class="Arr (strict)" method="Start Drag"("Data"=w284, "AllowsMove"=enum32{"copy or move", "copy only", "move only"}."move only" ("Drag Mode")) -> ()  [unwired: 3 in, 5 out]
              }
            }
          }
          event "dio64:tasks": Drop {
            n107 = event-data() -> ("Coords.Vertical"=w288:i32)  [unwired: 1 in]
            n108 = property on="dio64:tasks" class="Arr (strict)"() -> ("Number of Rows"=w306:u32, "Index Values"=w299:u32[])  [unwired: 2 in, 2 out]
            n109 = Bundle("32bit integer"=0, "32bit integer"=u16 0) -> (w294:T13)  [unwired: 1 in]
            n110 = Index Array(array=w299) -> (element=w298:u32)  [unwired: 1 in]
            n111 = Get Drag Drop Data(8:w294, 9:"dio64_task_drag" ("data name")) -> (3:w291:T13)  [unwired: 1 in, 1 out]
            n112 = property on="dio64:tasks" class="Arr (strict)"() -> ("Top"=w307:i32, "Height"=w308:u32)  [unwired: 2 in, 2 out]
            n113 = Unbundle(w291) -> ("32bit integer"=w289:i32, "32bit integer"=w290:u16)
            n114 = formula code="Y = (X-T-23)/(H-27);"("H"=w308, "T"=w307, "X"=w288) -> ("Y"=w303:dbl)
            n115 = In Range and Coerce(upper limit=1.0, x=w303, lower limit=0.0) -> (coerced(x)=w302:dbl)  [unwired: 1 out]
            n116 = Multiply(x=w302, y=w306) -> (x*y=w301:dbl)
            n117 = Round Toward -Infinity(1:w301) -> (0:w300:dbl)
            n118 = Add(x=w300, y=w298) -> (x+y=w297:dbl)
            n119 = To Long Integer(number=w297) -> (32bit integer=w296:i32)
            n120 = case shown="2" w290 {
              tunnel: w296 -> [_ w311]
              tunnel: w289 -> [_ w310]
              frame 0, Default {
              }
              frame 2 {
                n121 = local read "dio64:tasks"() -> (w313:T3)
                n122 = Delete From Array(array=w313, index=w310) -> (deleted portion=w314:T15, array with subset deleted=w315:T3)  [unwired: 1 in]
                n123 = Insert Into Array(array=w315, index=w311, new element=w314) -> (w312:T3)
                n124 = local write "dio64:tasks"(w312) -> ()
              }
            }
            n125 = event-data() -> ()  [unwired: 2 in, 1 out]
          }
          event "dio64:override": Value Change {
            n126 = event-data() -> ()  [unwired: 1 in, 5 out]
            n127 = Enqueue Element(queue=w318, element="DIO64: Override") -> (queue out=w317:refnum<queue>)  [unwired: 2 in, 2 out]
          }
          event "dio64:channel labels": Value Change {
            n128 = event-data() -> ()  [unwired: 1 in, 5 out]
            n129 = Enqueue Element(queue=w323, element="UI: DIO64 Labels") -> (queue out=w320:refnum<queue>)  [unwired: 2 in, 2 out]
            n130 = Enqueue Element(queue=w320, element=" \"DIO64: Update Graph\" ") -> (queue out=w319:refnum<queue>)  [unwired: 2 in, 2 out]
          }
          event "dio64:chop labels": Value Change {
            n131 = event-data() -> ()  [unwired: 1 in, 5 out]
            n132 = Enqueue Element(queue=w326, element="UI: Chop Labels") -> (queue out=w325:refnum<queue>)  [unwired: 2 in, 2 out]
          }
        }
        n133 = Get Queue Status(queue=w16, return elements? (F)=TRUE) -> (error out=w13:errorcluster, elements=→"queue":string[])  [unwired: 1 in, 6 out]
      }
    }
    frame Disabled {
    }
  }
  n134 = disable-structure shown="Enabled" {
    disable-tunnel: w1 -> [w327 _]
    frame Enabled {
      n135 = while "Matlab Communication Loop" {
        tunnel: w327 -> [w329]
        stop <- w334 stop-if-true
        w333 = u16 8888  # port
        n136 = call <vilib>:"TCP Listen.vi"("timeout ms (wait forever: -1)"=100, "port"=w333) -> ("error out"=w330:errorcluster, "connection ID"=w331:refnum<k5>)  [unwired: 5 in, 3 out]
        n137 = case shown="No Error" w330 {
          tunnel: w331 -> [w343 _]
          tunnel: w330 -> [w342 _]
          tunnel: w329 -> [w340 w561]
          tunnel: [w339 w561] -> w328
          frame No Error {
            n138 = TCP Read(connection ID=w343, bytes to read=4, error in (no error)=w342, 9:10000 ("timeout ms (25000)")) -> (connection ID out=w349:refnum<k5>, data out=w347:string, error out=w348:errorcluster)  [unwired: 1 in]
            n139 = Type Cast(type=u32 1 ("bytes to read"), x=w347) -> (*(type *) &x=w345:u32)
            n140 = To Long Integer(number=w345) -> (32bit integer=w344:i32)
            n141 = TCP Read(connection ID=w349, bytes to read=w344, error in (no error)=w348) -> (connection ID out=w337:refnum<k5>, data out=w341:string, error out=w338:errorcluster)  [unwired: 2 in]
            n142 = case shown="\"type\"" w341 {
              selector: w341 -> [w352 _ _ _ _ _ _ _]
              tunnel: w340 -> [w356 w367 w377 w387 w402 w447 w491 w541]
              tunnel: [w356 w367 w377 w387 w402 w447 w491 w541] -> w339
              tunnel: w338 -> [w355 w358 w373 w382 w400 w445 w489 w544]
              tunnel: [w354 w366 w376 w389 w412 w457 w501 w543] -> w336
              tunnel: w337 -> [w353 w362 w371 w383 w401 w446 w490 w540]
              tunnel: [w353 w361 w370 w388 w411 w456 w500 w539] -> w335
              frame "", Default {
                n143 = Enqueue Element(queue=w356, element=w352, error in (no error)=w355) -> (error out=w354:errorcluster)  [unwired: 1 in, 2 out]
              }
              frame "commands" {
                # "Send a list of commands that can be executed by the primary event loop to Matlab"
                n144 = property on="states" class="LstBox (strict)"(error in=w358) -> (error out=w357:errorcluster, "Item Names"=w359:string[])  [unwired: 1 in, 1 out]
                n145 = Flatten To String(anything=w359, error in (no error)=w357) -> (data string=w364:string, error out=w363:errorcluster)  [unwired: 2 in, 1 out]
                n146 = TCP Write(connection ID=w362, data in=w364, error in (no error)=w363) -> (connection ID out=w361:refnum<k5>, error out=w365:errorcluster)  [unwired: 1 in, 1 out]
                n147 = Enqueue Element(queue=w367, element="stdout >> Matlab is asking for a list of commands." ("string"), error in (no error)=w365) -> (error out=w366:errorcluster)  [unwired: 1 in, 2 out]
              }
              frame "documentation" {
                # "Sends an array of documentation strings grabbed from the text boxes in the main event loop that can be used by Matlab."
                n148 = local read "documentation"() -> (w368:string[])
                n149 = Flatten To String(anything=w368, error in (no error)=w373) -> (data string=w374:string, error out=w372:errorcluster)  [unwired: 2 in, 1 out]
                n150 = TCP Write(connection ID=w371, data in=w374, error in (no error)=w372) -> (connection ID out=w370:refnum<k5>, error out=w375:errorcluster)  [unwired: 1 in, 1 out]
                n151 = Enqueue Element(queue=w377, element="stdout >> Matlab is asking for documentation of commands." ("string"), error in (no error)=w375) -> (error out=w376:errorcluster)  [unwired: 1 in, 2 out]
              }
              frame "controls" {
                n152 = control-ref of="This VI"() -> (w378:refnum<vi>)
                n153 = call "all refs.vi"("VI"=w378) -> ("all controls"=w379:refnum<vi>[])
                n154 = for {
                  tunnel: w379 -> [w391] mode=indexing
                  tunnel: [w390] -> w385 mode=indexing
                  n155 = property class="Ctl"(reference=w391) -> ("Label.Text"=w390:string)  [unwired: 1 in, 2 out]
                }
                n156 = Flatten To String(anything=w385, error in (no error)=w382) -> (data string=w384:string, error out=w381:errorcluster)  [unwired: 2 in, 1 out]
                n157 = TCP Write(connection ID=w383, data in=w384, error in (no error)=w381) -> (connection ID out=w388:refnum<k5>, error out=w386:errorcluster)  [unwired: 1 in, 1 out]
                n158 = Enqueue Element(queue=w387, element="stdout >> Matlab is asking for a list of controls" ("string"), error in (no error)=w386) -> (error out=w389:errorcluster)  [unwired: 1 in, 2 out]
              }
              frame "type" {
                n159 = control-ref of="This VI"() -> (w393:refnum<vi>)
                n160 = TCP Read(connection ID=w401, bytes to read=4, error in (no error)=w400, 9:10000 ("timeout ms (25000)")) -> (connection ID out=w405:refnum<k5>, data out=w407:string, error out=w406:errorcluster)  [unwired: 1 in]
                n161 = Type Cast(type=u32 1 ("bytes to read"), x=w407) -> (*(type *) &x=w409:u32)
                n162 = call "all refs.vi"("VI"=w393) -> ("all controls"=w392:refnum<vi>[])
                n163 = To Long Integer(number=w409) -> (32bit integer=w410:i32)
                n164 = for {
                  tunnel: w392 -> [w436] mode=indexing
                  tunnel: [w435] -> w399 mode=indexing
                  n165 = property class="Ctl"(reference=w436) -> ("Label.Text"=w435:string)  [unwired: 1 in, 2 out]
                }
                n166 = TCP Read(connection ID=w405, bytes to read=w410, error in (no error)=w406) -> (connection ID out=w398:refnum<k5>, data out=w396:string, error out=w397:errorcluster)  [unwired: 2 in]
                n167 = Search 1D Array(1D array=w399, element=w396) -> (index of element=w394:i32)  [unwired: 1 in]
                n168 = Greater Or Equal To 0?(x=w394) -> (x >= 0?=w395:bool)
                n169 = case shown="True" w395 {
                  tunnel: [w414 w434] -> w412
                  tunnel: [w415 w427] -> w411
                  tunnel: w402 -> [_ w433]
                  tunnel: w392 -> [w426 _]
                  tunnel: w394 -> [w425 _]
                  tunnel: w398 -> [w421 w427]
                  tunnel: w397 -> [w420 w428]
                  tunnel: w396 -> [_ w430]
                  frame True {
                    n170 = Index Array(array=w426, index=w425) -> (element=w424:refnum<vi>)
                    n171 = property class="Ctl"(reference=w424) -> ("Value"=w413:variant)  [unwired: 1 in, 2 out]
                    n172 = call "ubinary_single.vi"("Cluster"=w413) -> ("Header"=w416:cluster{"Element Names":string[], u8[]})  [unwired: 9 in, 1 out]
                    n173 = Flatten To String(anything=w416) -> (data string=w418:string)  [unwired: 3 in, 2 out]
                    n174 = String Length(string=w418) -> (length=w417:i32)
                    n175 = Flatten To String(anything=w417) -> (data string=w419:string)  [unwired: 3 in, 2 out]
                    n176 = TCP Write(connection ID=w421, data in=w419, error in (no error)=w420) -> (connection ID out=w422:refnum<k5>, error out=w423:errorcluster)  [unwired: 1 in, 1 out]
                    n177 = TCP Write(connection ID=w422, data in=w418, error in (no error)=w423) -> (connection ID out=w415:refnum<k5>, error out=w414:errorcluster)  [unwired: 1 in, 1 out]
                  }
                  frame False {
                    n178 = Concatenate Strings("stdout >> Matlab is trying to read type of control " ("string"), w430, ", but it doesn't exist!" ("string")) -> (w431:string)
                    n179 = Enqueue Element(queue=w433, element=w431, error in (no error)=w428) -> (error out=w434:errorcluster)  [unwired: 1 in, 2 out]
                  }
                }
              }
              frame "read" {
                n180 = control-ref of="This VI"() -> (w438:refnum<vi>)
                n181 = TCP Read(connection ID=w446, bytes to read=4, error in (no error)=w445, 9:10000 ("timeout ms (25000)")) -> (connection ID out=w450:refnum<k5>, data out=w452:string, error out=w451:errorcluster)  [unwired: 1 in]
                n182 = Type Cast(type=u32 1 ("bytes to read"), x=w452) -> (*(type *) &x=w454:u32)
                n183 = call "all refs.vi"("VI"=w438) -> ("all controls"=w437:refnum<vi>[])
                n184 = To Long Integer(number=w454) -> (32bit integer=w455:i32)
                n185 = for {
                  tunnel: w437 -> [w480] mode=indexing
                  tunnel: [w479] -> w444 mode=indexing
                  n186 = property class="Ctl"(reference=w480) -> ("Label.Text"=w479:string)  [unwired: 1 in, 2 out]
                }
                n187 = TCP Read(connection ID=w450, bytes to read=w455, error in (no error)=w451) -> (connection ID out=w443:refnum<k5>, data out=w441:string, error out=w442:errorcluster)  [unwired: 2 in]
                n188 = Search 1D Array(1D array=w444, element=w441) -> (index of element=w439:i32)  [unwired: 1 in]
                n189 = Greater Or Equal To 0?(x=w439) -> (x >= 0?=w440:bool)
                n190 = case shown="True" w440 {
                  tunnel: [w458 w478] -> w457
                  tunnel: [w470 w471] -> w456
                  tunnel: w447 -> [_ w477]
                  tunnel: w437 -> [w467 _]
                  tunnel: w439 -> [w466 _]
                  tunnel: w443 -> [w459 w471]
                  tunnel: w442 -> [w460 w472]
                  tunnel: w441 -> [_ w474]
                  frame True {
                    n191 = Index Array(array=w467, index=w466) -> (element=w465:refnum<vi>)
                    n192 = property class="Ctl"(reference=w465) -> ("Value"=w461:variant)  [unwired: 1 in, 2 out]
                    n193 = Variant To Flattened String(Variant=w461) -> (data string=w462:string)  [unwired: 1 out]
                    n194 = String Length(string=w462) -> (length=w464:i32)
                    n195 = Flatten To String(anything=w464) -> (data string=w463:string)  [unwired: 3 in, 2 out]
                    n196 = TCP Write(connection ID=w459, data in=w463, error in (no error)=w460) -> (connection ID out=w469:refnum<k5>, error out=w468:errorcluster)  [unwired: 1 in, 1 out]
                    n197 = TCP Write(connection ID=w469, data in=w462, error in (no error)=w468) -> (connection ID out=w470:refnum<k5>, error out=w458:errorcluster)  [unwired: 1 in, 1 out]
                  }
                  frame False {
                    n198 = Concatenate Strings("stdout >> Matlab is trying to read the control " ("string"), w474, ", but it doesn't exist!" ("string")) -> (w475:string)
                    n199 = Enqueue Element(queue=w477, element=w475, error in (no error)=w472) -> (error out=w478:errorcluster)  [unwired: 1 in, 2 out]
                  }
                }
              }
              frame "write" {
                n200 = control-ref of="This VI"() -> (w482:refnum<vi>)
                n201 = TCP Read(connection ID=w490, bytes to read=4, error in (no error)=w489, 9:10000 ("timeout ms (25000)")) -> (connection ID out=w494:refnum<k5>, data out=w496:string, error out=w495:errorcluster)  [unwired: 1 in]
                n202 = Type Cast(type=u32 1 ("bytes to read"), x=w496) -> (*(type *) &x=w498:u32)
                n203 = call "all refs.vi"("VI"=w482) -> ("all controls"=w481:refnum<vi>[])
                n204 = To Long Integer(number=w498) -> (32bit integer=w499:i32)
                n205 = for {
                  tunnel: w481 -> [w538] mode=indexing
                  tunnel: [w537] -> w488 mode=indexing
                  n206 = property class="Ctl"(reference=w538) -> ("Label.Text"=w537:string)  [unwired: 1 in, 2 out]
                }
                n207 = TCP Read(connection ID=w494, bytes to read=w499, error in (no error)=w495) -> (connection ID out=w487:refnum<k5>, data out=w485:string, error out=w486:errorcluster)  [unwired: 2 in]
                n208 = Search 1D Array(1D array=w488, element=w485) -> (index of element=w483:i32)  [unwired: 1 in]
                n209 = Greater Or Equal To 0?(x=w483) -> (x >= 0?=w484:bool)
                n210 = case shown="True" w484 {
                  tunnel: [w528 w536] -> w501
                  tunnel: [w506 w529] -> w500
                  tunnel: w491 -> [w527 w535]
                  tunnel: w481 -> [w526 _]
                  tunnel: w483 -> [w525 _]
                  tunnel: w487 -> [w509 w529]
                  tunnel: w486 -> [w510 w530]
                  tunnel: w485 -> [w520 w532]
                  frame True {
                    n211 = TCP Read(connection ID=w509, bytes to read=4, error in (no error)=w510, 9:10000 ("timeout ms (25000)")) -> (connection ID out=w516:refnum<k5>, data out=w514:string, error out=w515:errorcluster)  [unwired: 1 in]
                    n212 = Index Array(array=w526, index=w525) -> (element=w524:refnum<vi>)
                    n213 = Type Cast(type=u32 1 ("bytes to read"), x=w514) -> (*(type *) &x=w512:u32)
                    n214 = property class="Ctl"(reference=w524) -> (reference out=w503:refnum<vi>, error out=w502:errorcluster, "Value"=w523:variant)  [unwired: 1 in]
                    n215 = To Long Integer(number=w512) -> (32bit integer=w511:i32)
                    n216 = Variant To Flattened String(Variant=w523) -> (1:w519:i16[])  [unwired: 1 out]
                    n217 = TCP Read(connection ID=w516, bytes to read=w511, error in (no error)=w515) -> (connection ID out=w506:refnum<k5>, data out=w508:string, error out=w507:errorcluster)  [unwired: 2 in]
                    n218 = Concatenate Strings("stdout >> Matlab is writing to control " ("string"), w520) -> (w521:string)
                    n219 = Flattened String To Variant(4:w502, 6:w508, 7:w519) -> (0:w504:errorcluster, 3:w505:variant)
                    n220 = property class="Ctl"(reference=w503, error in=w504, "Value"=w505) -> ()  [unwired: 2 out]
                    n221 = Enqueue Element(queue=w527, element=w521, error in (no error)=w507) -> (error out=w528:errorcluster)  [unwired: 1 in, 2 out]
                  }
                  frame False {
                    n222 = Concatenate Strings("stdout >> Matlab is trying to write to control " ("string"), w532, ", but it doesn't exist!" ("string")) -> (w533:string)
                    n223 = Enqueue Element(queue=w535, element=w533, error in (no error)=w530) -> (error out=w536:errorcluster)  [unwired: 1 in, 2 out]
                  }
                }
              }
              frame "sync" {
                # "Rendezvous at the \"sync\" point. If the primary event loop is in the \"Sync\" state, then this will allow the primary event loop to continue. Returns 1 If the main loop was waiting in the Sync state, and 1   if it wasn't. This allows Matlab to wait for Sync."
                n224 = call <vilib>:"Create Rendezvous.vi"("error in (no error)"=w544, "return existing (F)"=TRUE, "name (unnamed)"="sync") -> ("error out"=w542:errorcluster, "rendezvous"=w546:T16)  [unwired: 2 in, 1 out]
                n225 = case shown="Error" w542 {
                  tunnel: w546 -> [w554 _]
                  tunnel: w542 -> [w553 w555]
                  tunnel: [w551 w559] -> w543
                  tunnel: [w549 w558] -> w539
                  tunnel: w540 -> [w548 w557]
                  frame No Error {
                    n226 = call <vilib>:"Wait at Rendezvous.vi"("error in (no error)"=w553, "rendezvous"=w554) -> ("error out"=w550:errorcluster)  [unwired: 3 in, 2 out]
                    n227 = TCP Write(connection ID=w548, data in="\u0001", error in (no error)=w550) -> (connection ID out=w549:refnum<k5>, error out=w551:errorcluster)  [unwired: 1 in, 1 out]
                  }
                  frame Error {
                    n228 = call <vilib>:"Clear Errors.vi"("error in (no error)"=w555) -> ("error out"=w560:errorcluster)  [unwired: 6 in]
                    n229 = TCP Write(connection ID=w557, data in="\u0000", error in (no error)=w560) -> (connection ID out=w558:refnum<k5>, error out=w559:errorcluster)  [unwired: 1 in, 1 out]
                  }
                }
              }
            }
            n230 = TCP Close Connection(connection ID=w335, error in (no error)=w336) -> ()  [unwired: 1 in, 2 out]
          }
          frame Error {
          }
        }
        n231 = Get Queue Status(queue=w328) -> (error out=w334:errorcluster)  [unwired: 2 in, 7 out]
      }
    }
    frame Disabled {
    }
  }
  n232 = while "Main Event Loop" {
    shift-right: [w574] -> _
    shift-left: _ -> [w573]
    shift-right: [w562] -> w4
    shift-left: w6 -> [w569]
    shift-right: [w566] -> w5
    shift-left: w1 -> [w570]
    stop <- w575 stop-if-true
    w572 = 1  # Timeout
    n233 = Dequeue Element(queue=w570, error in (no error)=w569) -> (queue out=w567:refnum<queue>, element=w565:string, error out=w568:errorcluster)  [unwired: 1 in, 1 out]
    "current state" <- w565
    n234 = call <vilib>:"Parse State Queue__jki_lib_state_machine.vi"("State Queue"=w565, "Error In (no error)"=w568) -> ("Current State"=w571:string, "Arguments"=w564:string)  [unwired: 11 in, 1 out]
    n235 = call "string_split.vi"("input"=w564) -> ("output"=w563:string[])
    n236 = stacked-sequence {
      seq-local: [w576 _ _] -> [_ _ w1379]
      tunnel: w571 -> [_ w587 w1374]
      tunnel: w567 -> [_ w586 _]
      tunnel: w564 -> [_ w585 _]
      tunnel: [_ w584 _] -> w562
      tunnel: [_ w583 _] -> w566
      tunnel: [_ w582 _] -> w575
      tunnel: [_ w581 _] -> w574
      tunnel: w573 -> [_ w580 w1378]
      tunnel: w572 -> [_ w579 _]
      tunnel: w569 -> [_ w578 _]
      tunnel: w563 -> [_ w577 _]
      frame #0 {
        n237 = Tick Count (ms)() -> (millisecond timer value=w576:u32)
      }
      frame #1 {
        n238 = case shown="\"Pause\"" w587 {
          selector: w587 -> [_ _ w595 _ _ _ _ _ _ _ _ _ _ _ _ _ _ _ _ _ _ _ _ _ _ _ _ _ _ _ _ _ _ _ _ _ _ _ _ _ _ _ _]
          tunnel: w586 -> [w590 w591 w594 w605 w622 w634 w638 w644 w648 w656 w714 w759 w762 w782 w791 w833 w852 w871 w881 w885 w896 w917 w922 w928 w952 w961 w980 w1006 w1016 w1028 w1029 w1036 w1076 w1110 w1183 w1284 w1305 w1307 w1310 w1318 w1330 w1348 w1366]
          tunnel: w585 -> [_ _ _ _ _ _ _ _ _ _ _ _ _ w783 w792 _ _ _ _ _ _ _ _ _ _ _ _ _ _ _ _ _ _ _ _ _ _ _ _ _ _ _ _]
          tunnel: w580 -> [w588 w592 w597 w604 w624 w637 w639 _ w649 w659 w708 w760 w772 w786 w794 w832 w851 w870 w882 w889 w899 w918 w925 w929 w953 w962 w979 w1005 w1015 w1027 w1030 w1041 w1077 w1111 w1184 w1285 w1306 w1308 w1311 w1315 w1327 w1345 w1363]
          tunnel: [w589 w593 w599 w613 w620 w636 w640 w647 w650 w654 w705 w761 w764 w784 w795 w819 w839 w869 w883 w887 w890 w919 w926 w930 w947 w959 w976 w998 w1014 w1024 w1031 w1032 w1074 w1108 w1176 w1280 w1302 w1309 w1312 w1313 w1325 w1343 w1361] -> w584
          tunnel: w578 -> [w589 w593 w598 w613 w617 w636 w640 w647 w651 w655 w713 w761 w763 w785 w796 w820 w839 w869 w883 w886 w893 w919 w926 w930 w951 w956 w977 w1001 w1011 w1022 w1031 w1037 w1075 w1109 w1177 w1281 w1303 w1309 w1312 w1314 w1326 w1344 w1362]
          tunnel: [w590 w591 w594 w605 w621 w634 w638 w644 w648 w656 w714 w759 w769 w782 w791 w833 w852 w871 w881 w888 w897 w917 w922 w928 w949 w960 w980 w1006 w1016 w1028 w1029 w1035 w1076 w1110 w1183 w1284 w1305 w1307 w1310 w1318 w1330 w1348 w1366] -> w583
          tunnel: [_ _ _ _ _ TRUE _ _ _ _ _ _ _ _ _ _ _ _ _ _ _ _ _ _ _ _ _ _ _ _ _ _ _ _ _ _ _ _ _ _ _ _ _] -> w582
          tunnel: [w588 w592 w597 w614 w624 w637 w639 w641 w649 w658 w708 w760 w772 w786 w794 w832 w851 w870 w882 w889 w899 w918 w925 w929 w953 w962 w978 w1005 w1015 w1027 w1030 w1041 w1077 w1111 w1184 w1285 w1306 w1308 w1311 w1315 w1327 w1345 w1363] -> w581
          tunnel: w579 -> [_ _ _ _ _ _ _ _ _ _ _ _ _ _ _ _ _ _ _ _ _ _ _ _ _ _ _ _ _ _ _ _ _ _ _ _ _ _ _ _ _ _ _]
          tunnel: w577 -> [_ _ _ _ _ _ _ _ _ _ _ _ _ _ _ _ _ _ _ _ _ _ w921 w927 _ _ _ _ _ w1018 _ _ w1073 _ w1179 w1282 _ _ _ w1317 w1329 w1347 w1365]
          frame "", "Idle" {
            # "executes when the state queue is empty"
          }
          frame "---------- Core ----------" {
            # "Do not put any code in this frame.\n(it is a separator no-op)"
          }
          frame Default {
            w602 = 42 items=["No error", "Argument error", "Memory is full", "Out of zone", "End of file", "File already open", "Generic file I/O error", "File not found", "File permission error", "Disk is full", "Duplicate path", "Too many files open", "System feature not enabled", "Resource file not found", "Cannot add resource", "Resource not found", "Image not found", "Image memory error", "Pen does not exist", "Config type invalid", "Config token not found", "Config parse error", "Config memory error", "Bad external code format", "Bad external code offset", "External code not present", "Null window", "Destroy window error", "Null menu", "Print aborted", "Bad print record", "Print driver error", "Windows error during printing", "Memory error during printing", "Print dialog error", "Generic print error", "Invalid device refnum", "Device not found", "Device parameter error", "Device unit error", "Cannot open device", "Device call aborted", "Generic error", "Cancelled by user", "Object ID too low", "Object ID too high", "Object not in heap", "Unknown heap", "Unknown object (invalid DefProc)", "Unknown object (DefProc not in table)", "Message out of range", "Invalid (null) method", "Unknown message", "Manager call not supported", "Bad address", "Network operation in progress", "Network operation timed out", "Connection is busy", "Network attribute not supported", "Network error", "Address in use", "System out of memory", "Connection aborted", "Connection refused", "Not connected", "Already connected", "Connection closed", "Initialization error (interapplication manager)", "Bad occurrence", "Wait on unbound occurrence handler", "Occurrence queue overflow", "Datalog type conflict", "Unused", "Unrecognized type (interapplication manager)", "Memory corrupt", "Failed to make temporary DLL", "Old CIN version", "Drag socket not found", "Failed to load drop-object", "Failed to register OLE object", "Failed to release OLE object", "Format specifier type mismatch", "Unknown format specifier", "Too few format specifiers", "Too many format specifiers", "Scan failed", "Newer CIN version", "Error converting to variant", "Runtime menu error", "Password tampered", "Variant attribute not found", "Incompatible variant data type", "Event data is not available", "Event Store is not present", "Occurrence is not found", "Event Queue is not created", "Event info is not available", "Refnum passed is NULL", "Error retrieving Class GUID", "Error retrieving CoClass GUID", "Error retrieving TypeLib GUID.", "Bad built application magic bytes.", "Specific driver is different from the specific driver associated with the Logical Name.", "There is no session opened to the class driver.", "Max Error", "MAX - Error with config objects", "MAX - Error loading configuration", "MAX - Group not supported"]
            # "Do not delete, rename, or modify this frame.\n(this is used to capture unhandled states and typos)"
            # "Handle mistyped state name (developer tool)"
            n239 = Format Into String(format string="Software Exception: Unhandled State \"%s\"." ("message"), error in=w598, w595) -> (resulting string=w601:string, error out=w600:errorcluster)  [unwired: 1 in]
            n240 = call <vilib>:"Error Cluster From Error Code.vi"("show call chain? (False)"=FALSE, "error in (no error)"=w600, "error message (\"\")"=w601, "error code (0)"=w602) -> ("error out"=w599:errorcluster)  [unwired: 5 in]
          }
          frame "Initialize Core Data" {
            # "Do not delete, rename, or modify this frame.\n(this is used to determine panel behavior on exit)"
            # "originally closed?"
            # "exe?"
            # "If panel starts closed or is an EXE, then close it when we exit"
            n241 = control-ref of="Current VI Reference"() -> (w606:refnum<vi>)
            n242 = property class="VI"() -> ("Front Panel.Open"=w612:bool)  [unwired: 2 in, 2 out]
            n243 = property class="App"() -> ("App.Kind"=w611:T17)  [unwired: 2 in, 2 out]
            n244 = Not(x=w612) -> (.not. x?=w609:bool)
            n245 = Equal?(x=w611, y=T17."Run Time System" ("Application:Kind")) -> (x = y?=w608:bool)
            n246 = Or(x=w609, y=w608) -> (x .or. y?=w607:bool)
            n247 = Bundle By Name(cluster=w604, "Core.Current VI Reference"=w606, "Core.Close Panel on Exit?"=w607) -> (w614:T24)
          }
          frame "Error Handler" {
            w618 = T25 0 items=["no dialog", "OK message", "continue or stop message", "OK message + warnings", "continue/stop + warnings"] ("type of dialog (OK msg:1)")
            # "Handle any errors here.\nYou can also output any states to clean-up after errors occur"
            n248 = call <vilib>:"Simple Error Handler.vi"("type of dialog (OK msg:1)"=w618, "error in (no error)"=w617) -> ("source out"=w615:string, "error out"=w616:errorcluster)  [unwired: 3 in, 3 out]
            n249 = flat-sequence {
              tunnel: w615 -> [w625]
              frame #0 {
                n250 = local read "stdout"() -> (w632:string)
                n251 = Get Date/Time String() -> (date string=w628:string, time string=w629:string)  [unwired: 3 in]
                n252 = Concatenate Strings(w632, "\r\n", w628, " " ("string"), w629, ": " ("string"), w625) -> (w626:string)
                n253 = local write "stdout"(w626) -> ()
              }
              frame #1 {
                n254 = property on="stdout" class="Str"("Text.Scroll Position"=u32 4294967295) -> ()  [unwired: 2 in, 2 out]
              }
            }
            n255 = call <vilib>:"Clear Errors.vi"("error in (no error)"=w616) -> ("error out"=w619:errorcluster)  [unwired: 6 in]
            n256 = Enqueue Element At Opposite End(queue=w622, element="/*Post Error States", error in (no error)=w619) -> (queue out=w621:refnum<queue>, error out=w620:errorcluster)  [unwired: 1 in, 1 out]
          }
          frame "Exit" {
            # "Do not put any code in this frame.\n(No errors that occur here will be handled.)"
          }
          frame "---------- Data ----------" {
            # "Do not put any code in this frame.\n(It is a separator no-op. You can make a copy of this frame to create a new Data frame)"
          }
          frame "Data: Initialize" {
            w642 = string[] []  # pause queue
            w645 = string[] []  # case labels
            w646 = T26 {"Current VI Reference"=refnum, "Close Panel on Exit?"=FALSE}  # Core
            # "Initialize the shift-register data, here.\n(data names are defined by what you wire into the bundle function)"
            n257 = Bundle("Core"=w646, "case labels"=w645, "scope:resource"="scope:resource", "pause queue"=w642) -> (w641:T24)  [unwired: 1 in]
          }
          frame "Data: Cleanup" {
            # "Cleanup any data and references, here.\n(this is called automatically, by the Macro: Exit)"
            n258 = Unbundle By Name(w649) -> ("Core.Current VI Reference"=w652:refnum<vi>)
            n259 = Close Reference(reference=w652, error in (no error)=w651) -> (error out=w650:errorcluster)
          }
          frame "Data: Get Case Strings" {
            # "Gets the program states from the main loop case selector\n(Usage: \"Data: Get Case Strings\")"
            n260 = control-ref of="This VI"() -> (w661:refnum<vi>)
            n261 = property class="VI"(reference=w661, error in=w655) -> (error out=w663:errorcluster, "Diagram"=w664:refnum<vi>)  [unwired: 1 out]
            n262 = property class="TopLvlDiag"(reference=w664, error in=w663) -> (error out=w665:errorcluster, "AllObjs[]"=w662:refnum<vi>[])  [unwired: 1 out]
            n263 = while {
              tunnel: w662 -> [w702] mode=indexing
              tunnel: [w700] -> w660
              stop <- w699 continue-if-true
              w701 = refnum<vi> refnum  # WhileLoop
              n264 = To More Specific Class(target class=w701, reference=w702) -> (specific class reference=w700:refnum<vi>, error out=w699:errorcluster)  [unwired: 1 in]
            }
            n265 = property class="WLoop"(reference=w660, error in=w665) -> (error out=w668:errorcluster, "Diagram.AllObjs[]"=w670:refnum<vi>[])  [unwired: 1 out]
            n266 = while {
              tunnel: w670 -> [w692] mode=indexing
              tunnel: [w690] -> w667
              stop <- w689 continue-if-true
              w691 = refnum<vi> refnum  # Sequence
              n267 = To More Specific Class(target class=w691, reference=w692) -> (specific class reference=w690:refnum<vi>, error out=w689:errorcluster)  [unwired: 1 in]
            }
            n268 = property class="Seq"(reference=w667, error in=w668) -> (error out=w669:errorcluster, "Frames[]"=w674:refnum<vi>[])  [unwired: 1 out]
            n269 = for {
              tunnel: [w682] -> w671
              tunnel: w674 -> [w680] mode=indexing
              shift-right: [w681] -> w672
              shift-left: w669 -> [w684]
              stop <- w679 continue-if-true
              n270 = property class="Diag"(reference=w680, error in=w684) -> (error out=w681:errorcluster, "AllObjs[]"=w683:refnum<vi>[])  [unwired: 1 out]
              n271 = for {
                tunnel: w683 -> [w688] mode=indexing
                tunnel: [w686] -> w682
                tunnel: [w685] -> w679
                stop <- w685 continue-if-true
                w687 = refnum<vi> refnum  # CaseStructure
                n272 = To More Specific Class(target class=w687, reference=w688) -> (specific class reference=w686:refnum<vi>, error out=w685:errorcluster)  [unwired: 1 in]
              }
            }
            n273 = property class="CaseSel"(reference=w671, error in=w672) -> (error out=w654:errorcluster, "FrameNames"=w673:string[])  [unwired: 1 out]
            n274 = for {
              tunnel: w673 -> [w696] mode=indexing
              tunnel: [w693] -> w666 mode=indexing
              workers-P: _ -> [_]
              n275 = String Length(string=w696) -> (length=w695:i32)
              n276 = Subtract(x=w695, y=4) -> (x-y=w697:i32)
              n277 = String Subset(string=w696, offset (0)=2, length (rest)=w697) -> (substring=w693:string)
            }
            n278 = Array Subset(array=w666, index=6) -> (w653:string[])  [unwired: 1 in]
            n279 = for {
              tunnel: w653 -> [w678] mode=indexing
              tunnel: [w676] -> w657 mode=indexing
              workers-P: _ -> [_]
              n280 = Bundle(w678, 0) -> (w676:cluster{string, i32})  [unwired: 1 in]
            }
            n281 = Bundle By Name(cluster=w659, "case labels"=w653) -> (w658:T24)
            n282 = property on="states" class="LstBox (strict)"("Item Names"=w653) -> ()  [unwired: 2 in, 2 out]
            n283 = local write "debug timing"(w657) -> ()
          }
          frame "Data: Get Case Documentation" {
            # "Gets program documentation from main loop case selector\n(Usage: \"UI: Get Case Documentation\")"
            n284 = control-ref of="This VI"() -> (w716:refnum<vi>)
            n285 = property class="VI"(reference=w716, error in=w713) -> (error out=w718:errorcluster, "Diagram"=w719:refnum<vi>)  [unwired: 1 out]
            n286 = property class="TopLvlDiag"(reference=w719, error in=w718) -> (error out=w720:errorcluster, "AllObjs[]"=w717:refnum<vi>[])  [unwired: 1 out]
            n287 = while {
              tunnel: w717 -> [w758] mode=indexing
              tunnel: [w756] -> w715
              stop <- w755 continue-if-true
              w757 = refnum<vi> refnum  # WhileLoop
              n288 = To More Specific Class(target class=w757, reference=w758) -> (specific class reference=w756:refnum<vi>, error out=w755:errorcluster)  [unwired: 1 in]
            }
            n289 = property class="WLoop"(reference=w715, error in=w720) -> (error out=w722:errorcluster, "Diagram.AllObjs[]"=w724:refnum<vi>[])  [unwired: 1 out]
            n290 = while {
              tunnel: w724 -> [w754] mode=indexing
              tunnel: [w752] -> w721
              stop <- w751 continue-if-true
              w753 = refnum<vi> refnum  # Sequence
              n291 = To More Specific Class(target class=w753, reference=w754) -> (specific class reference=w752:refnum<vi>, error out=w751:errorcluster)  [unwired: 1 in]
            }
            n292 = property class="Seq"(reference=w721, error in=w722) -> (error out=w723:errorcluster, "Frames[]"=w725:refnum<vi>[])  [unwired: 1 out]
            n293 = for {
              tunnel: [w744] -> w712
              tunnel: w725 -> [w742] mode=indexing
              shift-right: [w743] -> w703
              shift-left: w723 -> [w746]
              stop <- w741 continue-if-true
              n294 = property class="Diag"(reference=w742, error in=w746) -> (error out=w743:errorcluster, "AllObjs[]"=w745:refnum<vi>[])  [unwired: 1 out]
              n295 = for {
                tunnel: w745 -> [w750] mode=indexing
                tunnel: [w748] -> w744
                tunnel: [w747] -> w741
                stop <- w747 continue-if-true
                w749 = refnum<vi> refnum  # CaseStructure
                n296 = To More Specific Class(target class=w749, reference=w750) -> (specific class reference=w748:refnum<vi>, error out=w747:errorcluster)  [unwired: 1 in]
              }
            }
            n297 = property class="CaseSel"(reference=w712, error in=w703) -> (error out=w707:errorcluster, "Frames[]"=w711:refnum<vi>[])  [unwired: 1 out]
            n298 = for {
              tunnel: w711 -> [w734] mode=indexing
              tunnel: [w727] -> w709 mode=indexing
              tunnel: w707 -> [w729]
              tunnel: [w729] -> w706 mode=indexing
              n299 = property class="Diag"(reference=w734, error in=w729) -> (error out=w731:errorcluster, "AllObjs[]"=w733:refnum<vi>[])  [unwired: 1 out]
              n300 = for {
                tunnel: w733 -> [w740] mode=indexing
                tunnel: [w738] -> w732
                tunnel: [w737] -> w730
                tunnel: w731 -> [w736]
                stop <- w737 continue-if-true
                w739 = refnum<vi> refnum  # Text
                n301 = To More Specific Class(target class=w739, reference=w740, error in=w736) -> (specific class reference=w738:refnum<vi>, error out=w737:errorcluster)
              }
              n302 = property class="Txt"(reference=w732, error in=w730) -> (error out=w728:errorcluster, "Text"=w726:string)  [unwired: 1 out]
              n303 = case shown="Error" w728 {
                tunnel: [w735 _] -> w727
                tunnel: w726 -> [w735 _]
                frame No Error {
                }
                frame Error {
                }
              }
            }
            n304 = Merge Errors(w706) -> (w705:errorcluster)
            n305 = Array Subset(array=w709, index=6) -> (→"documentation":string[])  [unwired: 1 in]
          }
          frame "---------- UI ----------" {
            # "Do not put any code in this frame.\n(It is a separator no-op. You can make a copy of this frame to create a new UI frame)"
          }
          frame "UI: Initialize" {
            # "Initialize the User Interface, here.\n(this is called automatically, by the Macro: Init)"
            n306 = local write "stdout"("") -> ()
            n307 = property on="tabs" class="TabCtl (strict)"(error in=w763) -> (error out=w767:errorcluster, "Pages"=w768:refnum<vi>[])  [unwired: 1 in, 1 out]
            n308 = for {
              tunnel: w768 -> [w781] mode=indexing
              shift-right: [w773] -> w766
              shift-left: w767 -> [w774]
              n309 = property class="Page"(reference=w781, error in=w774) -> (reference out=w780:refnum<vi>, error out=w775:errorcluster, "PageLabel"=w779:string)
              n310 = Match Pattern(string=w779, regular expression="^hidden") -> (offset past match=w777:i32)  [unwired: 1 in, 3 out]
              n311 = Less Than 0?(x=w777) -> (x < 0?=w776:bool)
              n312 = property class="Page"(reference=w780, error in=w775, "PageVis"=w776) -> (error out=w773:errorcluster)  [unwired: 1 out]
            }
            n313 = Enqueue Element At Opposite End(queue=w762, element="UI: Get Case Documentation" ("State(s) in Front (\"\")"), error in (no error)=w763) -> (queue out=w769:refnum<queue>, error out=w765:errorcluster)  [unwired: 1 in, 1 out]
            n314 = Merge Errors(w765, w766) -> (w764:errorcluster)
          }
          frame "UI: Cursor Set" {
            # "Set and Unset Cursor Busy.\n(Usage: \"UI: Cursor Set >> Busy|Idle\")"
            n315 = case shown="\"Idle\", Default" w783 {
              tunnel: w785 -> [w788 w790]
              tunnel: [w787 w789] -> w784
              frame "Idle", Default {
                n316 = call <vilib>:"Unset Busy.vi"("error in (no error)"=w788) -> ("error out"=w787:errorcluster)  [unwired: 10 in]
              }
              frame "Busy" {
                n317 = call <vilib>:"Set Busy.vi"("error in (no error)"=w790) -> ("error out"=w789:errorcluster)  [unwired: 9 in, 1 out]
              }
            }
          }
          frame "UI: Front Panel State" {
            # "Argument"
            # "Set Front Panel Open or Closed\n(Usage: \"UI: Front Panel State >> Open|Close\")"
            n318 = Unbundle By Name(w794) -> ("Core.Current VI Reference"=w793:refnum<vi>)
            n319 = case shown="\"Open\", Default" w792 {
              tunnel: w796 -> [w800 w813]
              tunnel: [w802 w814] -> w795
              tunnel: w793 -> [w801 w811]
              frame "Open", Default {
                n320 = property class="VI"(reference=w801, error in=w800) -> (reference out=w798:refnum<vi>, error out=w799:errorcluster, "Front Panel.Open"=w797:bool)
                n321 = case shown="True" w797 {
                  tunnel: [w805 w808] -> w802
                  tunnel: w799 -> [w804 w808]
                  tunnel: w798 -> [w803 _]
                  frame False {
                    n322 = invoke class="VI" method="FP.Open"(reference=w803, error in=w804, "Activate"=TRUE, "State"=T18."Standard") -> (error out=w805:errorcluster)  [unwired: 1 in, 4 out]
                  }
                  frame True {
                  }
                }
              }
              frame "Close" {
                n323 = property class="VI"(reference=w811, error in=w813) -> (reference out=w810:refnum<vi>, error out=w812:errorcluster, "Front Panel.Open"=w809:bool)
                n324 = case shown="True" w809 {
                  tunnel: [w815 w818] -> w814
                  tunnel: w812 -> [w815 w817]
                  tunnel: w810 -> [_ w816]
                  frame False {
                  }
                  frame True {
                    n325 = invoke class="VI" method="FP.Close"(reference=w816, error in=w817) -> (error out=w818:errorcluster)  [unwired: 1 in, 2 out]
                  }
                }
              }
            }
          }
          frame "UI: DIO64 Update Control" {
            w828 = "<SELF>"
            w830 = "T0"
            # "Updates DIO64 control with string from DIO64 Tasks\n(Usage: \"call after any modification to DIO64 Tasks\")"
            n326 = local read "dio64:tasks"() -> (w831:T3)
            n327 = for {
              tunnel: w831 -> [w836] mode=indexing
              tunnel: [w835] -> w826 mode=indexing
              workers-P: _ -> [_]
              n328 = Unbundle By Name(w836) -> ("Name"=w834:string)
              n329 = Bundle("Name"=w834, "Name"=w834) -> (w835:cluster{"Name":string, "Name":string})  [unwired: 1 in]
            }
            n330 = Bundle(w830, w830) -> (w829:cluster{string, string})  [unwired: 1 in]
            n331 = Bundle(w828, w828) -> (w827:cluster{string, string})  [unwired: 1 in]
            n332 = Build Array (concatenate)(w829, w826) -> (w825:cluster{"Name":string, "Name":string}[])
            n333 = Build Array (concatenate)(w827, w825) -> (w824:cluster{"Name":string, "Name":string}[])
            n334 = property on="Task" class="CmbBox"(error in=w820, "Strings And Values[]"=w826) -> (error out=w823:errorcluster)  [unwired: 1 in, 1 out]
            n335 = property on="begin reference" class="CmbBox"(error in=w820, "Strings And Values[]"=w825) -> (error out=w822:errorcluster)  [unwired: 1 in, 1 out]
            n336 = property on="end reference" class="CmbBox"(error in=w820, "Strings And Values[]"=w824) -> (error out=w821:errorcluster)  [unwired: 1 in, 1 out]
            n337 = Merge Errors(w823, w822, w821) -> (w819:errorcluster)
          }
          frame "UI: DIO64 Labels" {
            # "Updates DIO64 control with string from DIO64 Tasks\n(Usage: \"call after any modification to DIO64 Tasks\")"
            n338 = Transpose 2D Array(2D array="dio64:channel labels") -> (transposed array=w850:T5)
            n339 = for {
              tunnel: w850 -> [w854] mode=indexing
              tunnel: [w853] -> w849 mode=indexing
              n340 = for {
                tunnel: w854 -> [w865] mode=indexing
                tunnel: [w858] -> w853 mode=indexing
                n341 = Unbundle By Name(w865) -> ("Channel"=w864:string, "Name"=w863:string)
                n342 = Concatenate Strings(w864, "  " ("string"), w863) -> (w861:string)
                n343 = call <vilib>:"Draw Text at Point.vi"("text orientation"=T21."Counterclockwise", "[user-specified font]"=T19 {"Font Name:"="Application", "Size"=10, "Strikeout?"=FALSE, "Italic?"=FALSE, "Underline?"=FALSE, "Outline?"=FALSE, "Shadow?"=FALSE, "Bold?"=TRUE}, "desired font(Application)"=T20."User-specified Font", "text"=w861, "alignment(left, top)"=T22 {"horizontal"=enum."left", "vertical"=enum."bottom"}, "origin"=cluster{"x":i16, "y":i16} {"x"=0, "y"=90}) -> ("new picture"=w858:picture)  [unwired: 4 in, 1 out]
              }
            }
            n344 = Index Array(array=w849, index (row)=0) -> (element=w844:picture[])  [unwired: 1 in]
            n345 = Index Array(array=w849, index (row)=1) -> (element=w843:picture[])  [unwired: 1 in]
            n346 = Index Array(array=w849, index (row)=2) -> (element=w842:picture[])  [unwired: 1 in]
            n347 = Index Array(array=w849, index (row)=3) -> (element=w841:picture[])  [unwired: 1 in]
            n348 = local read "dio64:channel display"() -> (w840:T4)
            n349 = Bundle By Name(cluster=w840, "Channel 1"=w844, "Channel 2"=w843, "Channel 3"=w842, "Channel 4"=w841) -> (→"dio64:channel display":T4)
          }
          frame "UI: Chop Labels" {
            # "Updates DIO64 control with string from DIO64 Tasks\n(Usage: \"call after any modification to DIO64 Tasks\")"
            n350 = for {
              tunnel: "dio64:chop labels" -> [w874] mode=indexing
              tunnel: [w878] -> w868 mode=indexing
              tunnel: [w872] -> w866 mode=indexing
              i -> [w873]
              n351 = call <vilib>:"Draw Text at Point.vi"("text orientation"=T21."Counterclockwise", "[user-specified font]"=T19 {"Font Name:"="Application", "Size"=14, "Strikeout?"=FALSE, "Italic?"=FALSE, "Underline?"=FALSE, "Outline?"=FALSE, "Shadow?"=FALSE, "Bold?"=TRUE}, "desired font(Application)"=T20."User-specified Font", "text"=w874, "alignment(left, top)"=T22 {"horizontal"=enum."left", "vertical"=enum."bottom"}, "origin"=cluster{"x":i16, "y":i16} {"x"=0, "y"=150}) -> ("new picture"=w878:picture)  [unwired: 4 in, 1 out]
              n352 = Bundle("String"=w874, w873) -> (w872:cluster{"String":string, i32})  [unwired: 1 in]
            }
            "chop display" <- w868
            n353 = property on="Ring" class="Ring (strict)"("StringsAndValues[]"=w866) -> ()  [unwired: 2 in, 2 out]
            n354 = property on="dio64:display chop" class="Ring (strict)"("StringsAndValues[]"=w866) -> ()  [unwired: 2 in, 2 out]
          }
          frame "---------- Macro ----------" {
            # "Do not put any code in this frame.\n(It is a separator no-op. You can make a copy of this frame to create a new Macro frame)"
          }
          frame "Macro: Initialize" {
            # "Initialization Macro\n(This is called once, when the VI starts. It calls a number of other program states.)"
            n355 = call "queue_array_front.vi"("error in"=w886, "array"=string[] ["Data: Initialize", "Initialize Core Data", "Data: Get Case Strings", "Data: Get Case Documentation", "UI: Initialize", "UI: Front Panel State >> Open", "Delay >> 1000"], "queue in"=w885) -> ("error out"=w887:errorcluster, "queue out"=w888:refnum<queue>)  [unwired: 7 in]
          }
          frame "Macro: Exit" {
            # "Exit Macro\n(This is called once, when the VI exits)"
            n356 = Unbundle By Name(w899) -> ("Core.Close Panel on Exit?"=w898:bool)
            n357 = property on="tabs" class="TabCtl (strict)"(error in=w893) -> (error out=w894:errorcluster, "Pages"=w895:refnum<vi>[])  [unwired: 1 in, 1 out]
            n358 = for {
              tunnel: w895 -> [w901] mode=indexing
              shift-right: [w903] -> w892
              shift-left: w894 -> [w902]
              n359 = property class="Page"(reference=w901, error in=w902, "PageVis"=TRUE ("Page Visible")) -> (error out=w903:errorcluster)  [unwired: 1 out]
            }
            n360 = case shown="False" w898 {
              tunnel: w896 -> [w908 w916]
              tunnel: [w907 w912] -> w897
              tunnel: w893 -> [w905 w914]
              tunnel: [w904 w911] -> w891
              frame True {
                n361 = Enqueue Element At Opposite End(queue=w908, element="UI: Front Panel State >> Close", error in (no error)=w905) -> (queue out=w907:refnum<queue>, error out=w904:errorcluster)  [unwired: 1 in, 1 out]
              }
              frame False {
                n362 = Enqueue Element At Opposite End(queue=w916, element="Data: Cleanup", error in (no error)=w914) -> (queue out=w913:refnum<queue>, error out=w910:errorcluster)  [unwired: 1 in, 1 out]
                n363 = Enqueue Element At Opposite End(queue=w913, element="Exit", error in (no error)=w910) -> (queue out=w912:refnum<queue>, error out=w911:errorcluster)  [unwired: 1 in, 1 out]
              }
            }
            n364 = Merge Errors(w891, w892) -> (w890:errorcluster)
          }
          frame "---------- Utility ----------" {
            # "Template Separator\n(You can make a copy of, or modify, this frame)"
          }
          frame "delay" {
            # "Delays for some number of milliseconds\n(Usage: delay >>  TIME)"
            n365 = Index Array(array=w921) -> (element=w920:string)  [unwired: 1 in]
            n366 = Decimal String To Number(string=w920) -> (number=w924:i32)  [unwired: 2 in, 1 out]
            n367 = To Unsigned Long Integer(number=w924) -> (unsigned 32bit integer=w923:u32)
            n368 = Wait (ms)(milliseconds to wait=w923) -> ()  [unwired: 1 out]
          }
          frame "stdout" {
            # "Prints a message to the labview stdout control\n(Usage: stdout >> TEXT)"
            n369 = for {
              tunnel: w927 -> [w934] mode=indexing
              n370 = Format Date/Time String(time format string (%c)="%y%m%d %H:%M:%S") -> (date/time string=w932:string)  [unwired: 2 in]
              n371 = Concatenate Strings(w932, ": " ("string"), w934) -> (w933:string)
              n372 = flat-sequence {
                tunnel: w933 -> [w938]
                frame #0 {
                  n373 = local read "stdout"() -> (w939:string)
                  n374 = Concatenate Strings(w939, "\r\n", w938) -> (→"stdout":string)
                }
                frame #1 {
                  n375 = property on="stdout" class="Str"("Text.Scroll Position"=u32 4294967295) -> ()  [unwired: 2 in, 2 out]
                }
              }
            }
          }
          frame "Abort" {
            # "Clears the queue\n(Usage: abort)"
            n376 = Flush Queue(queue=w952, error in (no error)=w951) -> (queue out=w950:refnum<queue>, remaining elements=w941:string[], error out=w948:errorcluster)
            n377 = Array Size(array=w941) -> (size(s)=w942:i32)
            n378 = Number To Decimal String(number=w942) -> (decimal integer string=w943:string)  [unwired: 1 in]
            n379 = Concatenate Strings("stdout >> Clearing queue with " ("element"), w943, " elements remaining" ("element")) -> (w945:string)
            n380 = Enqueue Element At Opposite End(queue=w950, element=w945, error in (no error)=w948) -> (queue out=w949:refnum<queue>, error out=w947:errorcluster)  [unwired: 1 in, 1 out]
          }
          frame "Test" {
            # "Runs the test sequence\n(Usage: Test)"
            n381 = Current VI's Menubar() -> (w958:refnum<k9>)
            n382 = Get Menu Item Info(7:"Test" ("item tag"), 8:w956, 11:w958) -> (0:w955:errorcluster, 4:w954:bool)  [unwired: 5 out]
            n383 = case shown="True" w954 {
              tunnel: w961 -> [w964 w971]
              tunnel: [w964 w970] -> w960
              tunnel: [w963 w969] -> w959
              tunnel: w955 -> [w963 w965]
              frame False {
              }
              frame True {
                n384 = call "string_to_array.vi"("string"="test commands") -> ("array"=w967:string[])
                n385 = Build Array (concatenate)(w967, "Test" ("regular expression")) -> (w966:string[])
                n386 = call "queue_array_front.vi"("error in"=w965, "array"=w966, "queue in"=w971) -> ("error out"=w969:errorcluster, "queue out"=w970:refnum<queue>)  [unwired: 7 in]
              }
            }
          }
          frame "Pause" {
            # "Pauses the state machine\n(swaps out the queue to memory)"
            n387 = Current VI's Menubar() -> (w974:refnum<k9>)
            n388 = Get Menu Item Info(7:"Pause" ("item tag"), 11:w974) -> (4:w973:bool)  [unwired: 1 in, 6 out]
            n389 = case shown="False" w973 {
              tunnel: w980 -> [w986 w997]
              tunnel: w979 -> [w983 w996]
              tunnel: [w981 w995] -> w978
              tunnel: w977 -> [w985 w993]
              tunnel: [w984 w992] -> w976
              frame False {
                n390 = Bundle By Name(cluster=w983, "pause queue"=string[] []) -> (w981:T24)
                n391 = Unbundle By Name(w983) -> ("pause queue"=w987:string[])
                n392 = for {
                  tunnel: w987 -> [w990] mode=indexing
                  tunnel: w986 -> [w991]
                  shift-right: [w988] -> w984
                  shift-left: w985 -> [w989]
                  n393 = Enqueue Element At Opposite End(queue=w991, element=w990, error in (no error)=w989) -> (error out=w988:errorcluster)  [unwired: 1 in, 2 out]
                }
              }
              frame True {
                n394 = Flush Queue(queue=w997, error in (no error)=w993) -> (remaining elements=w994:string[], error out=w992:errorcluster)  [unwired: 1 out]
                n395 = Bundle By Name(cluster=w996, "pause queue"=w994) -> (w995:T24)
              }
            }
          }
          frame "Sync" {
            # "Waits for Sync\n(Creates a Rendezvous and waits for Matlab to send the Sync command. )"
            n396 = call <vilib>:"Create Rendezvous.vi"("error in (no error)"=w1001, "name (unnamed)"="sync") -> ("error out"=w1002:errorcluster, "rendezvous"=w1003:T16)  [unwired: 3 in, 1 out]
            n397 = call <vilib>:"Wait at Rendezvous.vi"("error in (no error)"=w1002, "rendezvous"=w1003) -> ("error out"=w999:errorcluster, "rendezvous out"=w1000:T16)  [unwired: 3 in, 1 out]
            n398 = call <vilib>:"Destroy Rendezvous.vi"("error in (no error)"=w999, "rendezvous"=w1000) -> ("error out"=w998:errorcluster)  [unwired: 4 in, 1 out]
          }
          frame "uBinary: Save" {
            # "Save every control to a ubin file"
            n399 = call "File Dialog2"("button label"="Save", "error in"=w1011, "pattern (all files)"="*.ubin", "pattern label"="uBinary") -> ("selected path"=w1012:path, "error out"=w1010:errorcluster)  [unwired: 8 in, 2 out]
            n400 = control-ref of="This VI"() -> (w1013:refnum<vi>)
            n401 = call "ubinary_save.vi"("error in"=w1010, "file (use dialog)"=w1012, "VI"=w1013) -> ("error out"=w1014:errorcluster)  [unwired: 8 in]
          }
          frame "uBinary: Load" {
            # "Loads a ubin file\n(will overwrite every control)"
            n402 = Index Array(array=w1018) -> (element=w1017:string)  [unwired: 1 in]
            n403 = call "File Dialog"("button label"="Load", "error in"=w1022, "pattern (all files)"="*.ubin", "pattern label"="uBinary") -> ("selected path"=w1025:path, "error out"=w1023:errorcluster)  [unwired: 8 in, 2 out]
            n404 = control-ref of="This VI"() -> (w1026:refnum<vi>)
            n405 = call "ubinary_load.vi"("error in"=w1023, "control"=w1017, "file (use dialog)"=w1025, "VI"=w1026) -> ("error out"=w1024:errorcluster)  [unwired: 7 in]
          }
          frame "---------- DIO64 ----------" {
            # "Template Separator\n(You can make a copy of, or modify, this frame)"
          }
          frame "DIO64: Initialize" {
            # "Initialize the DIO64"
            # "Initialize DIO64 Board"
            n406 = case shown="\"Windows 95/NT\"" T23."Windows x64" ("App.TargetOS") {
              tunnel: [w1044 w1051 w1059] -> w1040
              tunnel: w1037 -> [w1043 w1052 w1060]
              tunnel: "dio64:resource name" -> [w1042 _ _]
              frame "Windows x64" {
                n407 = call "DIO64 OpenResource.vi"("board in"=u16 0, "resourceName"=w1042, "error in (no error)"=w1043) -> ("board out"=w1045:u16, "error out"=w1047:errorcluster)  [unwired: 11 in]
                n408 = call "DIO64 Load.vi"("board in"=w1045, "input hint"=0, "output hint"=4, "filename"=path "C:/DIO64/DIO64.CAT", "error in (no error)"=w1047) -> ("error out"=w1044:errorcluster)  [unwired: 9 in, 1 out]
              }
              frame "Windows 95/NT" {
                n409 = call "DIO64 Open.vi"("board in"=u16 0, "error in (no error)"=w1052) -> ("board out"=w1053:u16, "error out"=w1055:errorcluster)  [unwired: 12 in]
                n410 = call "DIO64 Load.vi"("board in"=w1053, "input hint"=0, "output hint"=4, "error in (no error)"=w1055) -> ("error out"=w1051:errorcluster)  [unwired: 10 in, 1 out]
              }
              frame "invalid OS target", Default {
                n411 = Merge Errors(errorcluster {"status"=TRUE, "code"=0, "source"="DIO64: Unknown OS!!"} ("error constant"), w1060) -> (w1059:errorcluster)
              }
            }
            n412 = case shown="No Error" w1040 {
              tunnel: w1040 -> [w1061 w1065]
              tunnel: [w1061 w1062] -> w1033
              frame No Error {
              }
              frame Error {
                n413 = call <vilib>:"Error Cluster From Error Code.vi"("error in (no error)"=w1065, "error message (\"\")"="DIO64 Not Found!" ("error message (\"\")"), "error code (0)"=0) -> ("error out"=w1062:errorcluster)  [unwired: 6 in]
              }
            }
            n414 = Enqueue Element(queue=w1036, element="stdout >> Initializing DIO64", error in (no error)=w1033) -> (queue out=w1035:refnum<queue>, error out=w1032:errorcluster)  [unwired: 1 in, 1 out]
          }
          frame "DIO64: Prepare" {
            # "Parses the DIO64\n(Usage: DIO64: Prepare >> CHOP)"
            n415 = Index Array(array=w1073) -> (element=w1069:string)  [unwired: 1 in]
            n416 = local read "repetition rate"() -> (w1068:dbl)
            n417 = Decimal String To Number(string=w1069) -> (number=w1070:i32)  [unwired: 2 in, 1 out]
            n418 = local read "dio64"() -> (w1072:T2)
            n419 = local read "dio64:tasks"() -> (w1071:T3)
            n420 = call "Parse DIO64.vi"("error in"=w1075, "DIO64"=w1072) -> ("error out"=w1074:errorcluster, "times"=w1067:T7)  [unwired: 7 in]
            n421 = call "Prepare DIO64.vi"("Repetition Rate"=w1068, "chop"=w1070, "times"=w1067, "DIO64 Tasks"=w1071) -> ("DIO64 Debug"=→"dio64:debug1":T8)  [unwired: 6 in]
          }
          frame "DIO64: Update Graph" {
            # "Updates the DIO64 Timing Graph\n(Usage: call whenever the DIO64 changes)"
            n422 = local read "repetition rate"() -> (w1080:dbl)
            n423 = local read "dio64"() -> (w1107:T2)
            n424 = local read "dio64:tasks"() -> (w1106:T3)
            n425 = call "Parse DIO64.vi"("error in"=w1109, "DIO64"=w1107) -> ("error out"=w1108:errorcluster, "times"=w1079:T7)  [unwired: 7 in]
            "dio64:debug2" <- w1079
            n426 = local read "dio64:channel labels"() -> (w1087:T5)
            n427 = call "Prepare DIO64.vi"("Repetition Rate"=w1080, "chop"="dio64:display chop", "times"=w1079, "DIO64 Tasks"=w1106) -> ("DIO64 Debug"=w1092:T8)  [unwired: 6 in]
            n428 = for {
              tunnel: w1092 -> [w1172] mode=indexing
              tunnel: [w1171] -> w1093 mode=indexing
              tunnel: [w1170] -> w1098 mode=indexing
              tunnel: [w1169] -> w1100 mode=indexing
              tunnel: [w1168] -> w1102 mode=indexing
              tunnel: [w1167] -> w1104 mode=indexing
              workers-P: _ -> [_]
              n429 = Unbundle By Name(w1172) -> ("Begin (ms)"=w1171:dbl, "DIO64 Line 1"=w1170:bool[], "DIO64 Line 2"=w1169:bool[], "DIO64 Line 3"=w1168:bool[], "DIO64 Line 4"=w1167:bool[])
            }
            n430 = Transpose 2D Array(2D array=w1087) -> (transposed array=w1085:T5)
            n431 = Reshape Array(w1085, 64 ("dimension size")) -> (w1088:T27)
            n432 = Transpose 2D Array(2D array=w1098) -> (transposed array=w1099:bool[][])
            n433 = Transpose 2D Array(2D array=w1100) -> (transposed array=w1101:bool[][])
            n434 = Transpose 2D Array(2D array=w1102) -> (transposed array=w1103:bool[][])
            n435 = Transpose 2D Array(2D array=w1104) -> (transposed array=w1105:bool[][])
            n436 = for {
              tunnel: w1099 -> [w1164] mode=indexing
              tunnel: w1093 -> [w1153]
              tunnel: [w1166] -> w1094 mode=indexing
              tunnel: w1101 -> [w1161] mode=indexing
              tunnel: w1103 -> [w1159] mode=indexing
              tunnel: w1105 -> [w1157] mode=indexing
              tunnel: [w1152] -> w1095 mode=indexing
              tunnel: [w1151] -> w1096 mode=indexing
              tunnel: [w1150] -> w1097 mode=indexing
              workers-P: _ -> [_]
              n437 = Boolean To (0,1)(Boolean=w1164) -> (0, 1=w1163:i16[])
              n438 = Boolean To (0,1)(Boolean=w1161) -> (0, 1=w1162:i16[])
              n439 = Boolean To (0,1)(Boolean=w1159) -> (0, 1=w1160:i16[])
              n440 = Boolean To (0,1)(Boolean=w1157) -> (0, 1=w1158:i16[])
              n441 = To Double Precision Float(number=w1163) -> (double precision float=w1165:dbl[])
              n442 = To Double Precision Float(number=w1162) -> (double precision float=w1154:dbl[])
              n443 = To Double Precision Float(number=w1160) -> (double precision float=w1155:dbl[])
              n444 = To Double Precision Float(number=w1158) -> (double precision float=w1156:dbl[])
              n445 = Bundle(w1153, w1165) -> (w1166:cluster{dbl[], dbl[]})  [unwired: 1 in]
              n446 = Bundle(w1153, w1154) -> (w1152:cluster{dbl[], dbl[]})  [unwired: 1 in]
              n447 = Bundle(w1153, w1155) -> (w1151:cluster{dbl[], dbl[]})  [unwired: 1 in]
              n448 = Bundle(w1153, w1156) -> (w1150:cluster{dbl[], dbl[]})  [unwired: 1 in]
            }
            n449 = Build Array (concatenate)(w1094, w1095, w1096, w1097) -> (w1081:cluster{dbl[], dbl[]}[])
            n450 = for {
              tunnel: w1081 -> [w1133] mode=indexing
              tunnel: w1088 -> [w1132] mode=indexing
              shift-right: [w1127] -> _
              shift-left: 0.0 -> [w1128]
              shift-right: [w1122] -> w1089
              shift-left: cluster{dbl[], dbl[]}[] [] -> [w1126]
              shift-right: [w1124] -> w1090
              shift-left: string[] [] -> [w1123]
              n451 = Unbundle By Name(w1132) -> ("plot"=w1129:bool, "Channel"=w1131:string, "Name"=w1130:string)
              n452 = Concatenate Strings(w1131, w1130) -> (w1125:string)
              n453 = case shown="True" w1129 {
                tunnel: w1133 -> [_ w1148]
                tunnel: [w1135 w1143] -> w1122
                tunnel: w1125 -> [_ w1142]
                tunnel: w1128 -> [w1136 w1139]
                tunnel: [w1136 w1138] -> w1127
                tunnel: w1126 -> [w1135 w1145]
                tunnel: [w1134 w1141] -> w1124
                tunnel: w1123 -> [w1134 w1140]
                frame False {
                }
                frame True {
                  n454 = Unbundle(w1148) -> (w1146:dbl[], w1149:dbl[])
                  n455 = Add(x=w1149, y=w1139) -> (x+y=w1147:dbl[])
                  n456 = Bundle(cluster=w1148, w1146, w1147) -> (w1144:cluster{dbl[], dbl[]})
                  n457 = Subtract(x=w1139, y=1.2) -> (x-y=w1138:dbl)
                  n458 = Build Array (concatenate)(w1145, w1144) -> (w1143:cluster{dbl[], dbl[]}[])
                  n459 = Build Array (concatenate)(w1140, w1142) -> (w1141:string[])
                }
              }
            }
            n460 = for {
              tunnel: w1091 -> [w1114] mode=indexing
              i -> [w1113]
              n461 = flat-sequence {
                tunnel: w1114 -> [w1115]
                tunnel: [w1115] -> w1112
                tunnel: w1113 -> [w1116]
                tunnel: w1112 -> [w1117]
                frame #0 {
                  n462 = property on="dio64:timing graph" class="MixedGraph (strict)"("Active Plot"=w1116) -> ()  [unwired: 2 in, 2 out]
                }
                frame #1 {
                  n463 = property on="dio64:timing graph" class="MixedGraph (strict)"("Plot.Line Width"=u8 3, "Plot.Plot Interpolation"=u8 3, "Plot.Plot Name"=w1117) -> ()  [unwired: 2 in, 2 out]
                }
              }
            }
            n464 = flat-sequence {
              tunnel: w1089 -> [w1120]
              tunnel: w1090 -> [w1121]
              tunnel: [w1121] -> w1091
              frame #0 {
                "dio64:timing graph" <- w1120
              }
            }
          }
          frame "DIO64: Run" {
            # "Runs the DIO64\n(Usage: DIO64: Run )\n(Usage: DIO64: Run >> Chop,CHOP to run CHOP a number of times in the frame control)\n(Usage: DIO64: Run >> Repeat,N, to run the prepared sequence N times)"
            n465 = Index Array(array=w1179, index=0) -> (element=w1178:string)
            n466 = Index Array(array=w1179, index=1) -> (element=w1175:string)
            n467 = Index Array(array=w1179, index=2) -> (element=w1174:string)
            n468 = case shown="\"Chop\"" w1178 {
              tunnel: w1183 -> [w1192 w1229 _]
              tunnel: [w1189 w1227 w1249] -> w1176
              tunnel: w1177 -> [w1190 w1228 w1248]
              tunnel: w1175 -> [w1188 w1225 _]
              tunnel: w1174 -> [w1186 _ _]
              tunnel: "repetition rate" -> [w1185 w1224 w1247]
              frame "Chop" {
                n469 = case shown="\"0\", Default" w1186 {
                  selector: w1186 -> [w1194 _]
                  tunnel: [w1193 "frames"] -> w1191
                  frame "" {
                    n470 = Decimal String To Number(string=w1194) -> (number=w1193:i32)  [unwired: 2 in, 1 out]
                  }
                  frame "0", Default {
                  }
                }
                n471 = Decimal String To Number(string=w1188) -> (number=w1187:i32)  [unwired: 2 in, 1 out]
                n472 = for {
                  N: w1191 -> [_]
                  tunnel: w1192 -> [w1222]
                  shift-right: [w1199] -> w1189
                  shift-left: w1190 -> [w1200]
                  tunnel: w1187 -> [w1198]
                  tunnel: w1185 -> [w1197]
                  i -> [w1210]
                  stop <- w1218 stop-if-true
                  n473 = Index Array(array="dio64:chops", index=w1198) -> (element=w1202:cluster{"Chops":u16[]})
                  n474 = Unbundle By Name(w1202) -> ("Chops"=w1201:u16[])
                  n475 = Array Size(array=w1201) -> (size(s)=w1209:i32)
                  n476 = local read "dio64"() -> (w1208:T2)
                  n477 = local read "dio64:tasks"() -> (w1207:T3)
                  n478 = Quotient & Remainder(x=w1210, y=w1209) -> (x-y*floor(x/y)=w1204:i32)  [unwired: 1 out]
                  n479 = Index Array(array=w1201, index=w1204) -> (element=w1203:u16)
                  n480 = call "Parse DIO64.vi"("error in"=w1200, "DIO64"=w1208) -> ("error out"=w1211:errorcluster, "times"=w1206:T7)  [unwired: 7 in]
                  n481 = call "Prepare DIO64.vi"("Repetition Rate"=w1197, "chop"=w1203, "times"=w1206, "DIO64 Tasks"=w1207) -> ("DIO64 Debug"=w1212:T8)  [unwired: 6 in]
                  n482 = local write "dio64:debug2"(w1206) -> ()
                  n483 = case shown="True" "dio64:update display" {
                    tunnel: w1212 -> [_ w1223]
                    frame False {
                    }
                    frame True {
                      n484 = local write "dio64:debug1"(w1223) -> ()
                    }
                  }
                  n485 = Get Queue Status(queue=w1222, return elements? (F)=TRUE) -> (elements=w1221:string[])  [unwired: 1 in, 7 out]
                  n486 = call "dt_i to 0-t_i.vi"("DIO64 Debug"=w1212) -> ("output cluster"=w1214:cluster{bool[][], bool[][], bool[][], bool[][]}, "DIOArray out 1"=w1215:bool[][], "ti"=w1216:dbl[])  [unwired: 2 in]
                  n487 = Search 1D Array(1D array=w1221, element="Abort") -> (index of element=w1219:i32)  [unwired: 1 in]
                  n488 = Greater Or Equal To 0?(x=w1219) -> (x >= 0?=w1218:bool)
                  n489 = call "DIO64 Sequence.vi"("DIO64Addr (0)"=u16 0, "RepRate (Hz)"=w1197, "Time Array (ms)"=w1216, "Set DIO line .."=w1215, "output cluster"=w1214, "error in"=w1211) -> ("error out"=w1199:errorcluster)  [unwired: 9 in]
                  "current frame" <- w1210
                }
              }
              frame "Repeat" {
                n490 = case shown="\"0\", Default" w1225 {
                  selector: w1225 -> [w1231]
                  tunnel: [w1230] -> w1226
                  frame "0", Default {
                    n491 = Decimal String To Number(string=w1231) -> (number=w1230:i32)  [unwired: 2 in, 1 out]
                  }
                }
                n492 = for {
                  N: w1226 -> [_]
                  tunnel: w1229 -> [w1246]
                  shift-right: [w1235] -> w1227
                  shift-left: w1228 -> [w1234]
                  tunnel: w1224 -> [w1232]
                  i -> [w1233]
                  stop <- w1242 stop-if-true
                  n493 = local read "dio64:debug1"() -> (w1236:T8)
                  n494 = local write "current frame"(w1233) -> ()
                  n495 = Get Queue Status(queue=w1246, return elements? (F)=TRUE) -> (elements=w1245:string[])  [unwired: 1 in, 7 out]
                  n496 = call "dt_i to 0-t_i.vi"("DIO64 Debug"=w1236) -> ("output cluster"=w1238:cluster{bool[][], bool[][], bool[][], bool[][]}, "DIOArray out 1"=w1239:bool[][], "ti"=w1240:dbl[])  [unwired: 2 in]
                  n497 = Search 1D Array(1D array=w1245, element="Abort") -> (index of element=w1243:i32)  [unwired: 1 in]
                  n498 = Greater Or Equal To 0?(x=w1243) -> (x >= 0?=w1242:bool)
                  n499 = call "DIO64 Sequence.vi"("DIO64Addr (0)"=u16 0, "RepRate (Hz)"=w1232, "Time Array (ms)"=w1240, "Set DIO line .."=w1239, "output cluster"=w1238, "error in"=w1234) -> ("error out"=w1235:errorcluster)  [unwired: 9 in]
                }
              }
              frame Default {
                n500 = local read "dio64:debug1"() -> (w1250:T8)
                n501 = call "dt_i to 0-t_i.vi"("DIO64 Debug"=w1250) -> ("output cluster"=w1252:cluster{bool[][], bool[][], bool[][], bool[][]}, "DIOArray out 1"=w1253:bool[][], "ti"=w1254:dbl[])  [unwired: 2 in]
                n502 = call "DIO64 Sequence.vi"("DIO64Addr (0)"=u16 0, "RepRate (Hz)"=w1247, "Time Array (ms)"=w1254, "Set DIO line .."=w1253, "output cluster"=w1252, "error in"=w1248) -> ("error out"=w1249:errorcluster)  [unwired: 9 in]
              }
            }
          }
          frame "DIO64: Override" {
            w1270 = bool[] [FALSE, FALSE, FALSE, FALSE, FALSE, FALSE, FALSE, FALSE, FALSE, FALSE, FALSE, FALSE, FALSE, FALSE, FALSE, FALSE] ("DIO64 Line 4")
            w1261 = 10.0 ("Begin (ms)")
            # "DIO64: Override\n(Usage: DIO64: Override >> CHANNEL, to run a channel like A0 or C6)"
            n503 = Index Array(array=w1282, index=0) -> (element=w1256:string)
            n504 = String Subset(string=w1256, length (rest)=1 ("length (rest)")) -> (substring=w1264:string)  [unwired: 1 in]
            n505 = Decimal String To Number(string=w1256, offset=1 ("offset (0)")) -> (number=w1266:i32)  [unwired: 1 in, 1 out]
            n506 = In Range and Coerce(upper limit=15, x=w1266, lower limit=0) -> (coerced(x)=w1269:i32)  [unwired: 1 out]
            n507 = case shown="\"C\"" w1264 {
              tunnel: w1269 -> [w1289 w1293 w1297 w1301]
              tunnel: w1270 -> [w1286 w1290 w1294 w1298]
              tunnel: [w1287 w1290 w1294 w1298] -> w1271
              tunnel: [w1286 w1291 w1294 w1298] -> w1272
              tunnel: [w1286 w1290 w1295 w1298] -> w1273
              tunnel: [w1286 w1290 w1294 w1299] -> w1274
              frame "A", Default {
                n508 = Replace Array Subset(array=w1286, new element=TRUE ("new element/subarray"), index=w1289) -> (w1287:bool[])
              }
              frame "B" {
                n509 = Replace Array Subset(array=w1290, new element=TRUE ("new element/subarray"), index=w1293) -> (w1291:bool[])
              }
              frame "C" {
                n510 = Replace Array Subset(array=w1294, new element=TRUE ("new element/subarray"), index=w1297) -> (w1295:bool[])
              }
              frame "D" {
                n511 = Replace Array Subset(array=w1298, new element=TRUE ("new element/subarray"), index=w1301) -> (w1299:bool[])
              }
            }
            n512 = Bundle("Begin (ms)"=0.0, "Begin (ms)"=w1261, "DIO64 Line 4"=w1270, "DIO64 Line 4"=w1270, "DIO64 Line 4"=w1270, "DIO64 Line 4"=w1270) -> (w1259:T28)  [unwired: 1 in]
            n513 = Bundle("Begin (ms)"=w1261, "Begin (ms)"=w1261, "DIO64 Line 4"=w1271, "DIO64 Line 4"=w1272, "DIO64 Line 4"=w1273, "DIO64 Line 4"=w1274) -> (w1257:T28)  [unwired: 1 in]
            n514 = Bundle("Begin (ms)"=20.0, "Begin (ms)"=w1261, "DIO64 Line 4"=w1270, "DIO64 Line 4"=w1270, "DIO64 Line 4"=w1270, "DIO64 Line 4"=w1270) -> (w1260:T28)  [unwired: 1 in]
            n515 = Build Array(w1259, w1257, w1260) -> (w1255:T29)
            n516 = call "dt_i to 0-t_i.vi"("DIO64 Debug"=w1255) -> ("output cluster"=w1277:cluster{bool[][], bool[][], bool[][], bool[][]}, "DIOArray out 1"=w1278:bool[][], "ti"=w1279:dbl[])  [unwired: 2 in]
            n517 = call "DIO64 Sequence.vi"("DIO64Addr (0)"=u16 0, "RepRate (Hz)"=10000.0, "Time Array (ms)"=w1279, "Set DIO line .."=w1278, "output cluster"=w1277, "error in"=w1281) -> ("error out"=w1280:errorcluster)  [unwired: 9 in]
          }
          frame "DIO64: Close" {
            # "Closes the DIO64\n(Usage: DIO64: Close)"
            n518 = call "DIO64 Close.vi"("board in"=u16 0, "error in (no error)"=w1303) -> ("error out"=w1302:errorcluster)  [unwired: 12 in, 1 out]
          }
          frame "---------- DAC ----------" {
          }
          frame "---------- Scope ----------" {
          }
          frame "Scope: Initialize" {
            # "Initalize the Scope\n(Usage: Scope: Initialize >> SCOPE, where SCOPE can be DPO)"
            n519 = Index Array(array=w1317) -> (element=w1316:string)  [unwired: 1 in]
            n520 = case shown="\"DPO\"" w1316 {
              tunnel: w1315 -> [_ w1323]
              tunnel: w1314 -> [w1319 w1321]
              tunnel: [w1319 w1320] -> w1313
              frame "", Default {
              }
              frame "DPO" {
                w1324 = FALSE  # Reset
                n521 = Unbundle By Name(w1323) -> ("scope:resource"=w1322:refnum<visa-resource-name>)
                n522 = call <instrlib>:"Initialize.vi"("error in (no error)"=w1321, "Reset (True)"=w1324, "VISA resource name"=w1322) -> ("error out"=w1320:errorcluster)  [unwired: 7 in, 1 out]
              }
            }
          }
          frame "Scope: Settings" {
            # "Updates Scope Settings\n(Usage: Scope: Settings >> SCOPE, where SCOPE can be DPO)"
            n523 = Index Array(array=w1329) -> (element=w1328:string)  [unwired: 1 in]
            n524 = case shown="\"DPO\"" w1328 {
              tunnel: w1327 -> [_ w1342]
              tunnel: w1326 -> [w1331 w1338]
              tunnel: [w1331 w1333] -> w1325
              frame "", Default {
              }
              frame "DPO" {
                w1332 = u32 10 items=["1000 points"=1, "10k points"=10, "100k points"=100, "1M points"=1000, "5M points"=5000, "10M points"=10000] ("Record Length (10: 10k points)")
                w1337 = u16 0 items=["Channel 1", "Channel 2", "Channel 3", "Channel 4", "AC Line", "Aux", "Digital Channel 0", "Digital Channel 1", "Digital Channel 2", "Digital Channel 3", "Digital Channel 4", "Digital Channel 5", "Digital Channel 6", "Digital Channel 7", "Digital Channel 8", "Digital Channel 9", "Digital Channel 10", "Digital Channel 11", "Digital Channel 12", "Digital Channel 13", "Digital Channel 14", "Digital Channel 15", "RF"] ("Trigger Source (0: Channel 1)")
                n525 = Unbundle By Name(w1342) -> ("scope:resource"=w1341:refnum<visa-resource-name>)
                n526 = call <instrlib>:"Configure Acquisition.vi"("error in (no error)"=w1338, "VISA resource name"=w1341) -> ("error out"=w1339:errorcluster, "VISA resource name out"=w1340:refnum<visa-resource-name>)  [unwired: 8 in]
                n527 = call-poly <instrlib>:"Configure Trigger.vi"("VISA resource name"=w1340, "Trigger Source (0: Channel 1)"=w1337, "Trigger Level (0.0 V)"=1.4, "error in (no error)"=w1339) -> ("VISA resource name out"=w1335:refnum<visa-resource-name>, "error out"=w1334:errorcluster)  [unwired: 10 in]
                n528 = call <instrlib>:"Configure Timebase.vi"("Record Length (10: 10k points)"=w1332, "error in (no error)"=w1334, "VISA resource name"=w1335) -> ("error out"=w1333:errorcluster)  [unwired: 7 in, 1 out]
              }
            }
          }
          frame "Scope: Read" {
            # "Reads a frame from the Scope\n(Usage: Scope: Read >> SCOPE, where SCOPE can be DPO)"
            n529 = Index Array(array=w1347) -> (element=w1346:string)  [unwired: 1 in]
            n530 = case shown="\"DPO\"" w1346 {
              tunnel: w1345 -> [_ w1355]
              tunnel: w1344 -> [w1349 w1354]
              tunnel: [w1349 w1353] -> w1343
              frame "", Default {
              }
              frame "DPO" {
                n531 = Unbundle By Name(w1355) -> ("scope:resource"=w1352:refnum<visa-resource-name>)
                n532 = for {
                  tunnel: w1352 -> [w1358]
                  shift-right: [w1359] -> w1353
                  shift-left: w1354 -> [w1360]
                  tunnel: "scope:channels" -> [w1357] mode=indexing
                  tunnel: [w1356] -> w1350 mode=indexing
                  n533 = call-poly <instrlib>:"Fetch Waveform.vi"("error in (no error)"=w1360, "Channel (0: Channel 1)"=w1357, "VISA resource name"=w1358) -> ("error out"=w1359:errorcluster, "Waveform Data"=w1356:waveform(dbl))  [unwired: 6 in, 1 out]
                }
                "scope" <- w1350
              }
            }
          }
          frame "Scope: Close" {
            # "Close the Scope\n(Usage: Scope: Close >> SCOPE, where SCOPE can be DPO)"
            n534 = Index Array(array=w1365) -> (element=w1364:string)  [unwired: 1 in]
            n535 = case shown="\"DPO\"" w1364 {
              tunnel: w1363 -> [_ w1371]
              tunnel: w1362 -> [w1367 w1369]
              tunnel: [w1367 w1368] -> w1361
              frame "", Default {
              }
              frame "DPO" {
                n536 = Unbundle By Name(w1371) -> ("scope:resource"=w1370:refnum<visa-resource-name>)
                n537 = call <instrlib>:"Close.vi"("error in (no error)"=w1369, "VISA resource name"=w1370) -> ("error out"=w1368:errorcluster)  [unwired: 9 in]
              }
            }
          }
        }
      }
      frame #2 {
        n538 = Unbundle By Name(w1378) -> ("case labels"=w1377:string[])
        n539 = Tick Count (ms)() -> (millisecond timer value=w1380:u32)
        n540 = Subtract(x=w1380, y=w1379) -> (x-y=w1376:u32)
        n541 = Search 1D Array(1D array=w1377, element=w1374) -> (index of element=w1372:i32)  [unwired: 1 in]
        n542 = Bundle("Current State"=w1374, w1376) -> (w1375:cluster{"Current State":string, u32})  [unwired: 1 in]
        n543 = Greater Or Equal To 0?(x=w1372) -> (x >= 0?=w1373:bool)
        n544 = case shown="True" w1373 {
          tunnel: w1372 -> [_ w1383]
          tunnel: w1375 -> [_ w1382]
          frame False {
          }
          frame True {
            n545 = local read "debug timing"() -> (w1381:cluster{"command":string, "time":dbl}[])
            n546 = in-place {
              in-place-border: w1382 -> [w1385]
              n547 = in-place-array #1(w1381, w1383) -> ()  [unwired: 1 out]
              n548 = in-place-array #1(w1385) -> (→"debug timing":cluster{"command":string, "time":dbl}[])  [unwired: 1 out]
            }
          }
        }
      }
    }
  }
  n549 = Release Queue(queue=w5, error in (no error)=w4) -> (error out=w3:errorcluster)  [unwired: 1 in, 2 out]
  n550 = call <vilib>:"Simple Error Handler.vi"("error in (no error)"=w3) -> ()  [unwired: 4 in, 5 out]
